vi "myRIO_BRig_RT_v0,75__PortC.vi"() -> ()   [LabVIEW 2014]
uses:
  <vilib>/Platform/TimedLoop/XDataNode/XDataNode.xnode
  <vilib>/Platform/TimedLoop/XDataNode/nitl_modes.ctl
  <vilib>/Platform/TimedLoop/XDataNode/XDNodeRunTimeDep.lvlib
  <vilib>/Platform/TimedLoop/XDataNode/wakeup.ctl
  <vilib>/Platform/TimedLoop/XDataNode/timing_clust.ctl
  <vilib>/rvi/interface/nirviReadWriteControl/nirviReadWriteControl.xnode
  <vilib>/rvi/interface/Simulation/niFpgaSimulationCallBeginRW.vi
  <vilib>/rvi/errors/niLvFpgaAdjustHostInterfaceError.vi
  <vilib>/rvi/interface/nirviCloseFPGA/nirviCloseFPGA.xnode
  <vilib>/myRIO/Instrument Drivers/Utilities/Utilities.lvlib
  <vilib>/rvi/interface/nirviOpenFPGA/nirviOpenFPGA.xnode
  myRIO_BRig_RT__Case_Exp_stateList.ctl
  <vilib>/WebDAVClient/Advanced/SessionHandle.ctl
  <vilib>/WebDAVClient/NI_WebDAV.lvlib
  myRIO_BRig_RT__Case_NonExp_stateList.ctl
  NiFpgaLv.dll
  <vilib>/Utility/error.llb/Error Cluster From Error Code.vi
  myRIO_BRig_FPGA_v3,60__PortC__build.lvbitx
  myRIO_BRig_FPGA_v3,60__PortC.vi
  <vilib>/FPGAPlugInAG/myRIO-1900/niLvFpga_Open_myRIO-1900.vi
  <vilib>/rvi/interface/common/dynamic/niFpgaDynamicAddResources.vi
  <vilib>/FPGAPlugInAG/Dynamic/niLvFpga_Close_Dynamic.vi
panel:
  in  "LC_Sel_All_Count":u16
  in  "LC_Sel_First_Count":u16
  in  "LC_Sel_All_Probability":u16
  in  "LC_Sel_All_Block":u16(slide) max=2 step=1 scale=0.0..2.0
  in  "LC_Sel_All_OnOff":bool
  in  "LC_Sel_First_Probability":u16
  in  "LC_Sel_First_Block":u16(slide) max=2 step=1 scale=0.0..2.0
  in  "LC_Sel_First_OnOff":bool
  in  "LC_Sel_All_Tdelay":u16
  in  "LC_Sel_First_Tdelay":u16
  out "I_connect_TCP":bool
  out "error out 5":errorcluster
  in  "get_countPerMS":bool
  in  "count_warmup_R_reset":bool
  in  "count_warmup_L_reset":bool
  out "count_warmup_R":u16
  out "count_warmup_L":u16
  out "SolenoidReward":bool
  in  "SolenoidProbability_L":u16=50 caption="Reward Time [ms]" min=1 max=1000 step=1
  in  "SolenoidProbability_R":u16=50 caption="Reward Time [ms]" min=1 max=1000 step=1
  out "output_PortA":dbl caption="LaserPower"
  out "error out 4":errorcluster
  in  "laser_power_step":dbl
  in  "laser_power_max":dbl
  in  "Recording":bool
  out "error out 3":errorcluster
  out "error out 2":errorcluster
  in  "laser_power_min":dbl
  in  "f_millisec2count":dbl=159.0
  in  "laser_Tshutter":dbl=2.0
  in  "laser_Freq":dbl=10.0
  in  "laser_Tpeak":dbl=2.0
  in  "laser_duration":u16
  out "error out":errorcluster
  in  "LC_Cue1_All_Count":u16
  in  "LC_Cue1_First_Count":u16
  in  "LC_Cue1_All_delayOpt":bool
  in  "LC_ENL1_All_delayOpt":bool
  in  "LC_ENL1_All_Count":u16
  in  "LC_ENL1_First_Count":u16
  in  "LC_Cue1_First_delayOpt":bool
  in  "LC_ENL1_First_delayOpt":bool
  in  "Tcycle_Cue_max":u16=1000 caption="Max" min=5 max=5000 step=5
  in  "Tcycle_Cue_min":u16=1000 caption="Min" min=5 max=5000 step=5
  in  "SendData":bool
  out "cSpout":enum16{"Left", "Right"}(ring) caption="Left or Right Spout"
  out "A4":u32 caption="LickCounter_Right"
  out "A2":u32 caption="LickCounter_Left"
  in  "laserResponse_wrong_LED":bool
  out "error_initTrial":errorcluster
  out "error_Selection_pre":errorcluster
  out "error_Selection":errorcluster
  out "SelectWrong":bool
  out "SelectReward":bool
  in  "Left(F)_or_Right(T)":bool
  in  "ignoreWrong":bool
  in  "SelectionState":bool
  in  "laserResponse_wrong":bool
  in  "laserResponse_reward":bool
  in  "laserResponse_reward_LED":bool
  out "nRewards_Right":u16 caption="# Rewards Total (Right)"
  out "nRewards_Left":u16 caption="# Rewards Total (Left)"
  out "nRewards_cur":u16 caption="# Rewards in Current Block"
  out "TpB_target":u16 caption="Target Trials Per Block"
  out "cState_NonExp":T1 caption="WarmUp State"
  out "iBlock":u16 caption="Current Block"
  out "cState":T2 caption="Experimental State"
  out "iTrial":u16 caption="Current Trial"
  in  "warmupType":u8(slide) max=2 step=1 scale=0.0..2.0
  in  "TestConnection":bool
  in  "warmup":bool caption="WarmUp"
  in  "Data Set Prefix":string="Exp1_TM2"
  out "Connected To Host?":bool
  in  "Host Password":string="sabalab"
  in  "Host UserName":string="Test2"
  in  "sp_RightSpout":u16(slide)=2 max=2 step=1 scale=0.0..2.0
  in  "sp_LeftSpout":u16(slide)=2 max=2 step=1 scale=0.0..2.0
  in  "BUR_max":u16 caption="Count Reward Structure  (0 = off)"
  in  "LC_Wrong_Probability":u16
  in  "LC_Wrong_Trial":u16(slide) max=2 step=1 scale=0.0..2.0
  in  "LC_Wrong_Block":u16(slide) max=2 step=1 scale=0.0..2.0
  in  "LC_Wrong_OnOff":bool
  in  "LC_Reward_Probability":u16
  in  "LC_Reward_Trial":u16(slide) max=2 step=1 scale=0.0..2.0
  in  "LC_Reward_Block":u16(slide) max=2 step=1 scale=0.0..2.0
  in  "LC_Reward_OnOff":bool
  in  "LC_Cue1_All_Probability":u16
  in  "LC_Cue1_All_Block":u16(slide) max=2 step=1 scale=0.0..2.0
  in  "LC_Cue1_All_OnOff":bool
  in  "LC_Cue1_First_Probability":u16
  in  "LC_Cue1_First_Block":u16(slide) max=2 step=1 scale=0.0..2.0
  in  "LC_Cue1_First_OnOff":bool
  in  "LC_ENL1_All_Probability":u16 max=100 step=1
  in  "LC_ENL1_All_Block":u16(slide) max=2 step=1 scale=0.0..2.0
  in  "LC_ENL1_All_OnOff":bool
  in  "LC_ENL1_First_Probability":u16 max=100 step=1
  in  "LC_ENL1_First_Block":u16(slide) max=2 step=1 scale=0.0..2.0
  in  "Tcycle_Timeout":u16=1000 caption="Timeout Time [ms]" min=10 max=10000 step=1
  in  "Tcycle_Wrong":u16=1000 caption="Wrong Time [ms]" min=10 max=10000 step=1
  in  "Tcycle_Selection":u16=1000 caption="Answer Time [ms]" min=1 max=10000 step=1
  in  "Tcycle_RewardPost":u16=1000 caption="Consumption Time [ms]" min=250 max=10000 step=250
  in  "Tcycle_Reward_L":u16=500 caption="Reward Time [ms]" min=1 max=1000 step=1
  in  "Tcycle_Reward_R":u16=500 caption="Reward Time [ms]" min=1 max=1000 step=1
  in  "TpB_Max_R":u16=4 caption="Max TrialsPerBlock" min=1 max=12 step=1
  in  "TpB_Min_R":u16=4 caption="Min TrialsPerBlock" min=1 max=12 step=1
  in  "TpB_Max_L":u16=4 caption="Max TrialsPerBlock" min=1 max=12 step=1
  in  "TpB_Min_L":u16=4 caption="Min TrialsPerBlock" min=1 max=12 step=1
  in  "BUR_min":u16 caption="Count Reward Structure\n(0 = off)"
  in  "TrialUntilReward":bool caption="Ignore Wrong Selection"
  in  "CueCycles":u16=1 caption="Cue Structure" min=1 max=1 step=1
  in  "MTrig_Laser_Tcycle":u16=10 caption="Time [ms]"
  in  "MTrig_Laser_trig":bool
  in  "MTrig_Audio_trig__R":bool caption="Trigger Audio"
  in  "MTrig_Audio_trig__L":bool caption="Trigger Audio"
  in  "RewCalib_Trig_R":bool caption="Calibrate_R"
  in  "RewCalib_Trig_L":bool caption="Calibrate_L"
  in  "MTrig_Solenoid_Tcycle__R":u16=300 caption="Time [ms]"
  in  "MTrig_Solenoid_Tcycle__L":u16=300 caption="Time [ms]"
  in  "MTrig_Solenoid_trig__R":bool caption="Solenoid"
  in  "MTrig_Solenoid_trig__L":bool caption="Solenoid"
  in  "STOP_abort":bool caption="Stop LabView\n(Stops myRio and FPGA)"
  in  "STOP_endBlock":bool caption="Stop Experiment\n@ End of Block"
  in  "STOP_endTrial":bool caption="Stop Experiment\n@ End of Trial"
  in  "START":bool caption="Start Experiment"
  in  "Tcycle_CuePenalty":u16=1000 caption="Penalty" min=1 max=10000 step=1
  in  "Audio_Amp__R":u16=100 caption="Amp"
  in  "Audio_Freq__R":u8=5 caption="Freq [kHz]" max=14 step=1
  in  "Audio_Amp__L":u16=100 caption="Amp"
  in  "Audio_Freq__L":u8=5 caption="Freq [kHz]" max=14 step=1
  in  "LC_Wrong_Tdelay":u16
  in  "LC_Cue1_All_Tdelay":u16
  in  "LC_ENL1_All_Tdelay":u16
  in  "LC_Reward_Tdelay":u16
  in  "LC_Cue1_First_Tdelay":u16
  in  "LC_ENL1_First_Tdelay":u16
  in  "LC_ENL1_First_OnOff":bool
  in  "Tcycle_ENLPenalty":u16=100 caption="Penalty" min=10 max=10000 step=10
  in  "Tcycle_ENL_max":u16=1000 caption="Max" min=250 max=10000 step=250
  in  "Tcycle_ENL_min":u16=1000 caption="Min" min=250 max=10000 step=250
  # "Communication (Host PC)"
  # "Recording Rig"
  # "Experimental Run"
  # "Current State"
  # "STOP experiment at"
  # "Global Parameters                                                         Trial Parameters"
  # "Left/Right        Give Reward?        Laser Power [V]"
  # "FPGA Count per [ms]"
  # "Experiment Task Structure"
  # "Timing [ms]"
  # "Block                   Trial            Target Trials       # Rewards \n                                                            Per Block             Current"
  # "Min            Max            Penalty"
  # "(1) = Switching\n(2) = Two Choice"
  # "WarmUp State"
  # "Lick Counter"
  # "Enforced\nNonLick"
  # "WarmUp"
  # "Left           Right"
  # "Cue then reward (no lick)\n \nLeft                    Right"
  # "# Rewards Total\n                                                                  Left                    Right"
  # "Cue"
  # "Experimental State"
  # "Selection\n \n\n \nReward\n    Dispense\n    Time\n \n    Dispense\n    Probability\n \n\n    Consumption\n    Time\n\nWrong Choice\n \n \nTimeout Penalty"
  # "Laser Control\n                               On/Off      Block        Probability [%]   Delay [ms]                              Count"
  # "Left                  Right"
  # "Manual Control"
  # "Enforced\nNonLick\n      1"
  # "Min"
  # "Max"
  # "from end"
  # "Solenoid\n \nLeft              Right"
  # "Switch\nTrial"
  # "Speaker\n \nLeft                    Right"
  # "Laser"
  # "from start"
  # "Trial Per Block Structure \n               Left                        Right"
  # "from end"
  # "NonSwitch\nTrials"
  # "from start"
  # "Time\n[ms]"
  # "Time\n[ms]"
  # "Time = Cue Min"
  # "Min"
  # "Cue 1"
  # "Power = Min"
  # "from end"
  # "Switch\nTrial"
  # "Max"
  # "from start"
  # "Speaker Parameters"
  # "Laser Parameters"
  # "Left                  Right"
  # "from end"
  # "Laser Response\n                               On/Off      Block       Trial       Probability [%]   Delay [ms]"
  # "Frequency\n[Hz]"
  # "NonSwitch\nTrials"
  # "Frequency\n[kHz]"
  # "from start"
  # "Timing [ms]\n Duration     Peak Width   Shutter"
  # "Selection Reward"
  # "Selection"
  # "Amp\n(0 - 32,000)"
  # "from start"
  # "Switch\nTrial"
  # "Laser Power [V]\nMin          Max              Step"
  # "Speaker\nPattern\nDuring Cue"
  # "Selection Wrong"
  # "from start"
  # "NonSwitch\nTrials"
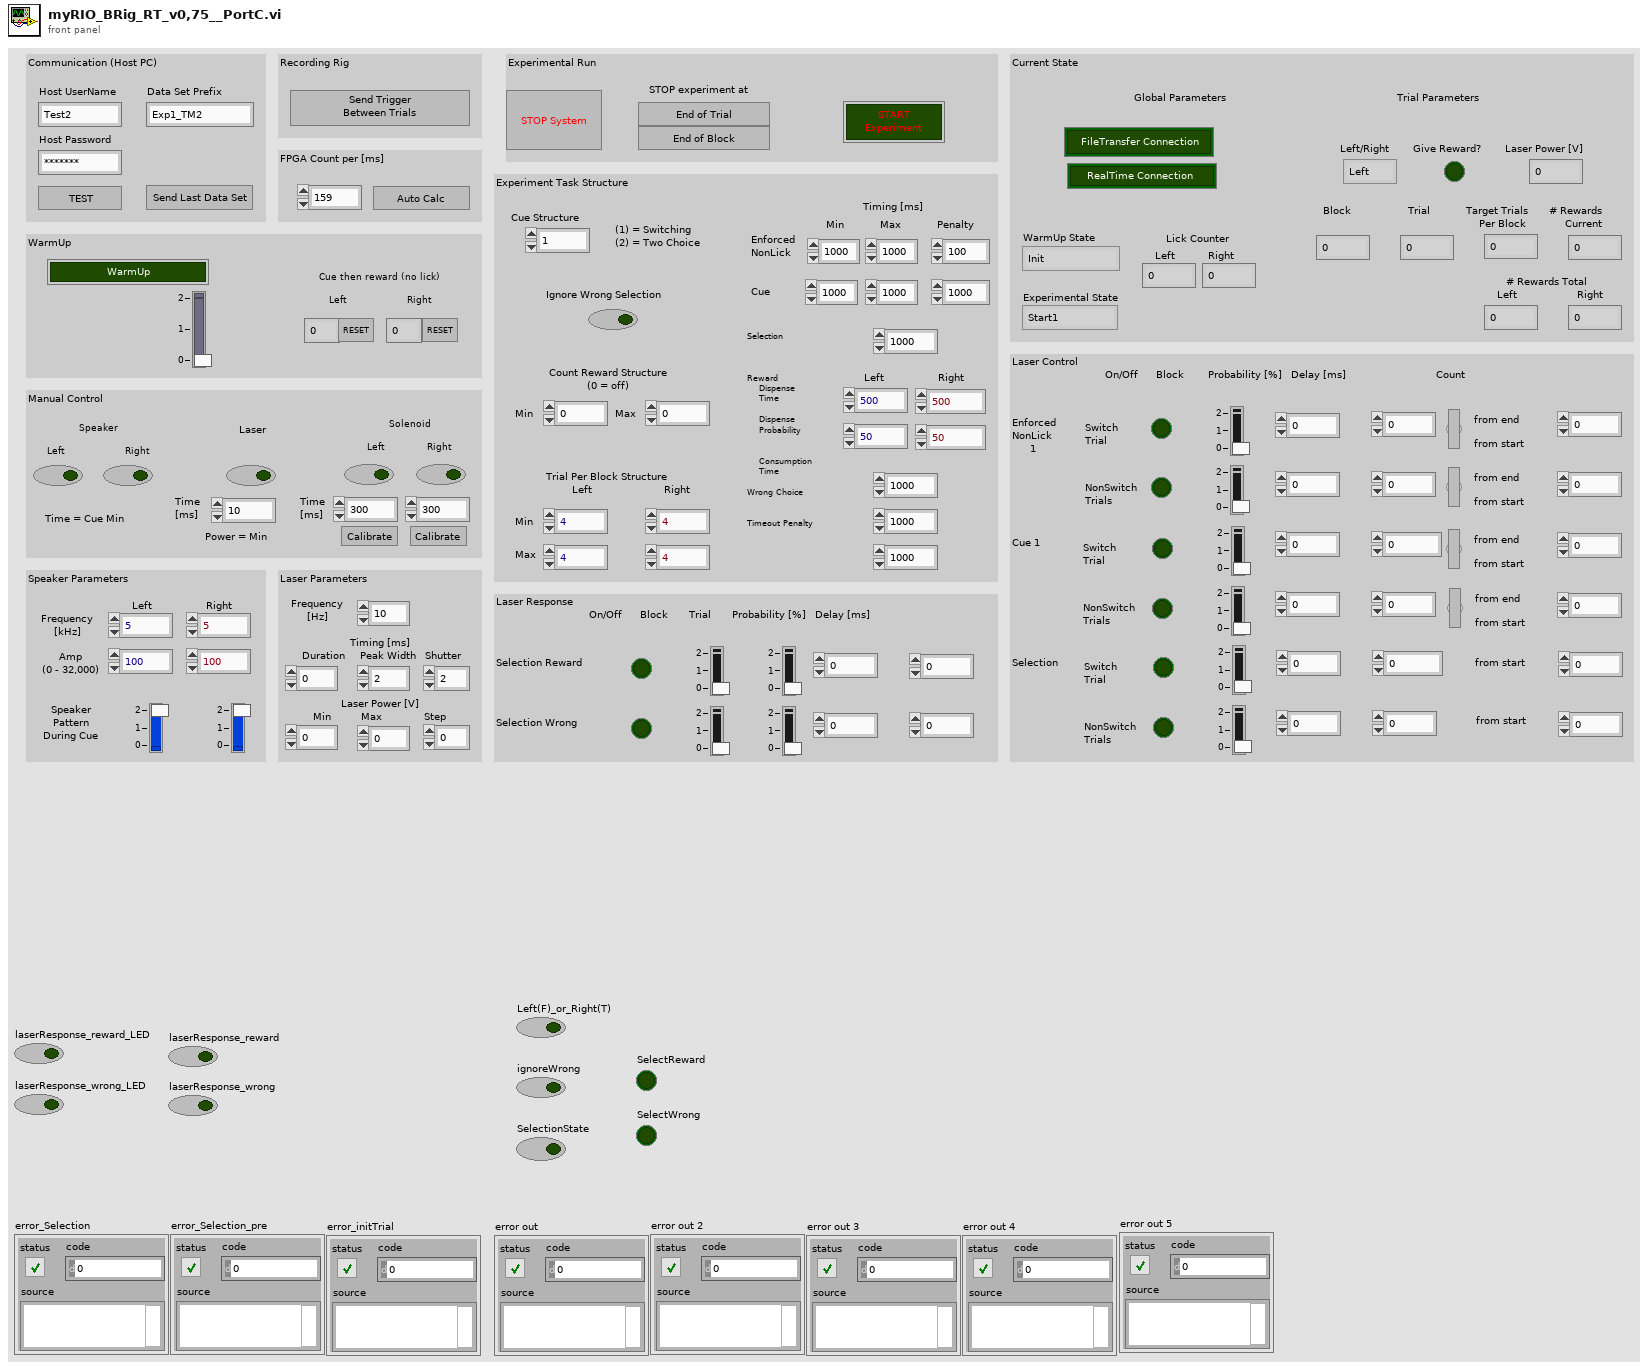
[diagram p1: front panel]
types:
  T1 = typedef "myRIO_BRig_RT__Case_NonExp_stateList.ctl" = enum16{"Init", "UploadSettings_pre", "UploadSettings_Read_dataExp", "UploadSettings_dataExp_1", "UploadSettings_Read_dataLC", "UploadSettings_dataLC_1", "UploadSettings_dataLC_2", "UploadSettings_Read_dataMTrig", "UploadSettings_dataMTrig_1", "UploadSettings_post", "Idle_pre", "IdleEmpty", "IdleEmpty2", "IdleEmpty3", "IdleEmpty4", "Idle", "Idle_2", "Idle_3", "Idle_4", "Idle_post", "Cue_pre__pre", "Cue_pre", "Cue", "Cue_post", "RewardCalibration_pre", "DispenseWater_pre__pre", "DispenseWater_pre", "DispenseWater", "DispenseWater_post", "TestConnection", "SendData", "Get_FPGA_count_per_ms", "End"}
  T2 = typedef "myRIO_BRig_RT__Case_Exp_stateList.ctl" = enum16{"Start1", "Start2", "Start3", "saveSettings1", "saveSettings2", "saveSettings3", "saveSettings4_LC_l1_ENL", "saveSettings4_LC_l2_ENL", "saveSettings5_LC_l1_Cue", "saveSettings5_LC_l2_Cue", "saveSettings6_LC_l1_Other", "SaveSettings6_LC_l2_Other", "setSettings_Audio", "setSettings_Laser", "initBlock_pre", "initBlock", "initBlock2", "initBlock_post", "initTrial_pre", "initTrial", "initTrial2", "initTrial3", "initTrial4", "initTrial_LC_ENL1", "initTrial_LC_Cue1", "initTrial_LC_Sel", "initTrial_post", "ENL1_pre", "ENL1", "ENL1_post", "ENL1Penalty_pre", "ENL1Penalty", "ENL2_pre", "ENL2", "ENL2Penalty_pre", "ENL2Penalty", "Cue1_pre", "Cue1", "Cue1_post", "Cue1Penalty_pre", "Cue1Penalty", "Cue2_pre", "Cue2", "Cue2Penalty_pre", "Cue2Penalty", "Selection_pre", "Selection", "Select_post", "SelectReward_pre", "SelectReward", "SelectRewardPost_pre", "SelectRewardPost", "SelectWrong_pre", "SelectWrong", "SelectWrong_post", "SelectTimeout_pre", "SelectTimeout", "SelectTimeout_post", "endTrial_pre", "endTrial1", "endTrial2", "endTrial3", "endTrial_post", "endBlock_pre", "endBlock", "endBlock_post", "endExp", "commConnect", "commUpload_pre", "commUpload_dataBlock", "commUpload_dataCurrent", "commUpload_dataExp", "commUpload_dataLC", "commUpload_dataTrial", "commUpload_post", "saveData_pre", "saveData_dataBlock", "saveData_dataCurrent", "saveData_dataExp", "saveData_dataLC", "saveData_dataTrial", "saveData_post", "empty_endBlock1", "empty_endBlock2", "empty_endTrial1", "empty_endTrial2", "empty_endTrial3", "empty_endTrial4", "empty_endTrial5", "dummyState", "dummyState_endBlock"}
  T3 = typedef "XDNodeRunTimeDep.lvlib/timing_clust.ctl" = cluster{"Expected End [f-1]":u64, "Actual End [f-1]":u64, "Finished Late? [f-1]":bool, "Expected End [i-1]":u64, "Actual End [i-1]":u64, "Finished Late? [i-1]":bool, "Expected Start [i]":u64, "Actual Start [i]":u64, "Expected Start [f]":u64, "Actual Start [f]":u64, "Source Name":string, "Structure Name":string, "Period":i64, "Deadline":i64, "Offset":i64, "Start":i64, "Priority":i32, "Timeout":i32, "Mode":T4, "Wakeup Reason":T5, "Error":errorcluster, "Source Type":string, "Secondary Source Type":string, "Global End Time":u64, "Global Start Time":u64, "Frame Duration":u64, "Iteration Duration":u64, "Assigned CPU":i32, "I/O Scan Engine Mode":u32}
  T4 = typedef "XDNodeRunTimeDep.lvlib/nitl_modes.ctl" = enum32{"No Change", "Process missed periods, maintain original phase", "Discard missed periods, maintain original phase", "Process missed periods, ignore original phase", "Discard missed periods, ignore original phase"}
  T5 = typedef "XDNodeRunTimeDep.lvlib/wakeup.ctl" = enum32{"Normal", "Aborted", "Asynchronous wakeup", "Timing source error", "Timed loop error", "Timeout"}
  T6 = typedef "myRIO_BRig_RT__Case_Exp_stateList.ctl" = enum16{"Start1", "Start2", "Start3", "saveSettings1", "saveSettings2", "saveSettings3", "saveSettings4_LC_ENL", "saveSettings5_LC_Cue", "saveSettings6_LC_Other", "setSettings_Audio", "setSettings_Laser", "initBlock_pre", "initBlock", "initBlock2", "initBlock_post", "initTrial_pre", "initTrial", "initTrial2", "initTrial3", "initTrial4", "initTrial_LC_ENL1", "initTrial_LC_Cue1", "initTrial_LC_Sel", "initTrial_post", "ENL1_pre", "ENL1", "ENL1_post", "ENL1Penalty_pre", "ENL1Penalty", "ENL2_pre", "ENL2", "ENL2Penalty_pre", "ENL2Penalty", "Cue1_pre", "Cue1", "Cue1_post", "Cue1Penalty_pre", "Cue1Penalty", "Cue2_pre", "Cue2", "Cue2Penalty_pre", "Cue2Penalty", "Selection_pre", "Selection", "Select_post", "SelectReward_pre", "SelectReward", "SelectRewardPost_pre", "SelectRewardPost", "SelectWrong_pre", "SelectWrong", "SelectWrong_post", "SelectTimeout_pre", "SelectTimeout", "SelectTimeout_post", "endTrial_pre", "endTrial1", "endTrial2", "endTrial3", "endTrial_post", "endBlock_pre", "endBlock", "endBlock_post", "endExp", "commConnect", "commUpload_pre", "commUpload_dataBlock", "commUpload_dataCurrent", "commUpload_dataExp", "commUpload_dataLC", "commUpload_dataTrial", "commUpload_post", "saveData_pre", "saveData_dataBlock", "saveData_dataCurrent", "saveData_dataExp", "saveData_dataLC", "saveData_dataTrial", "saveData_post", "empty_endBlock1", "empty_endBlock2", "empty_endTrial1", "empty_endTrial2", "empty_endTrial3", "empty_endTrial4", "empty_endTrial5", "dummyState", "dummyState_endBlock"}
  T7 = typedef "NI_WebDAV.lvlib/SessionHandle.ctl" = refnum<k1>
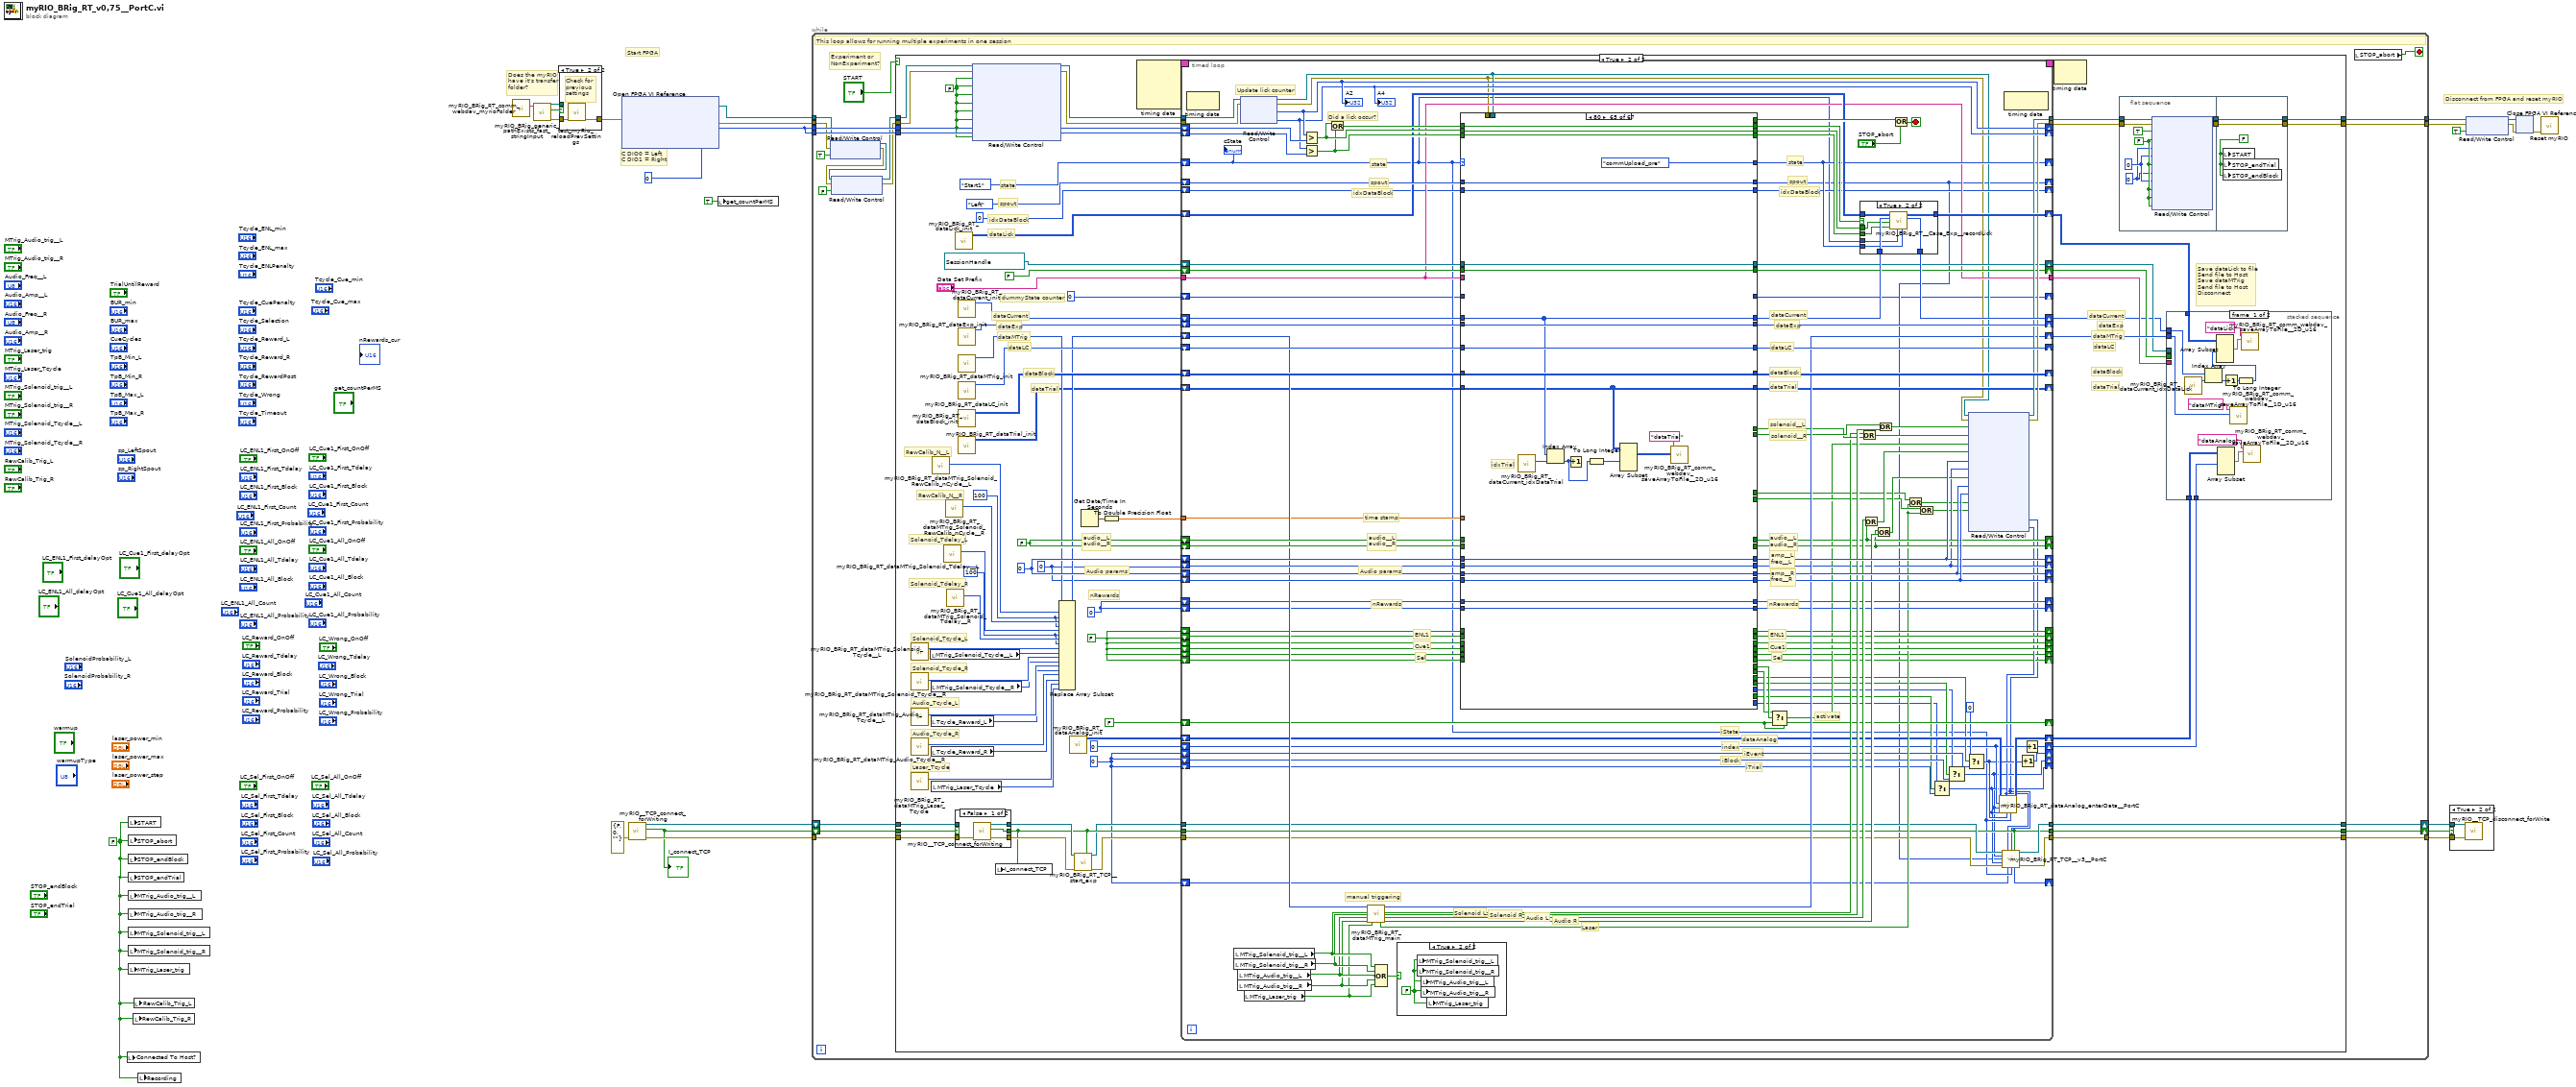
[diagram p0: block diagram]
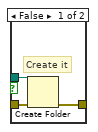
[diagram p3: hidden frame]
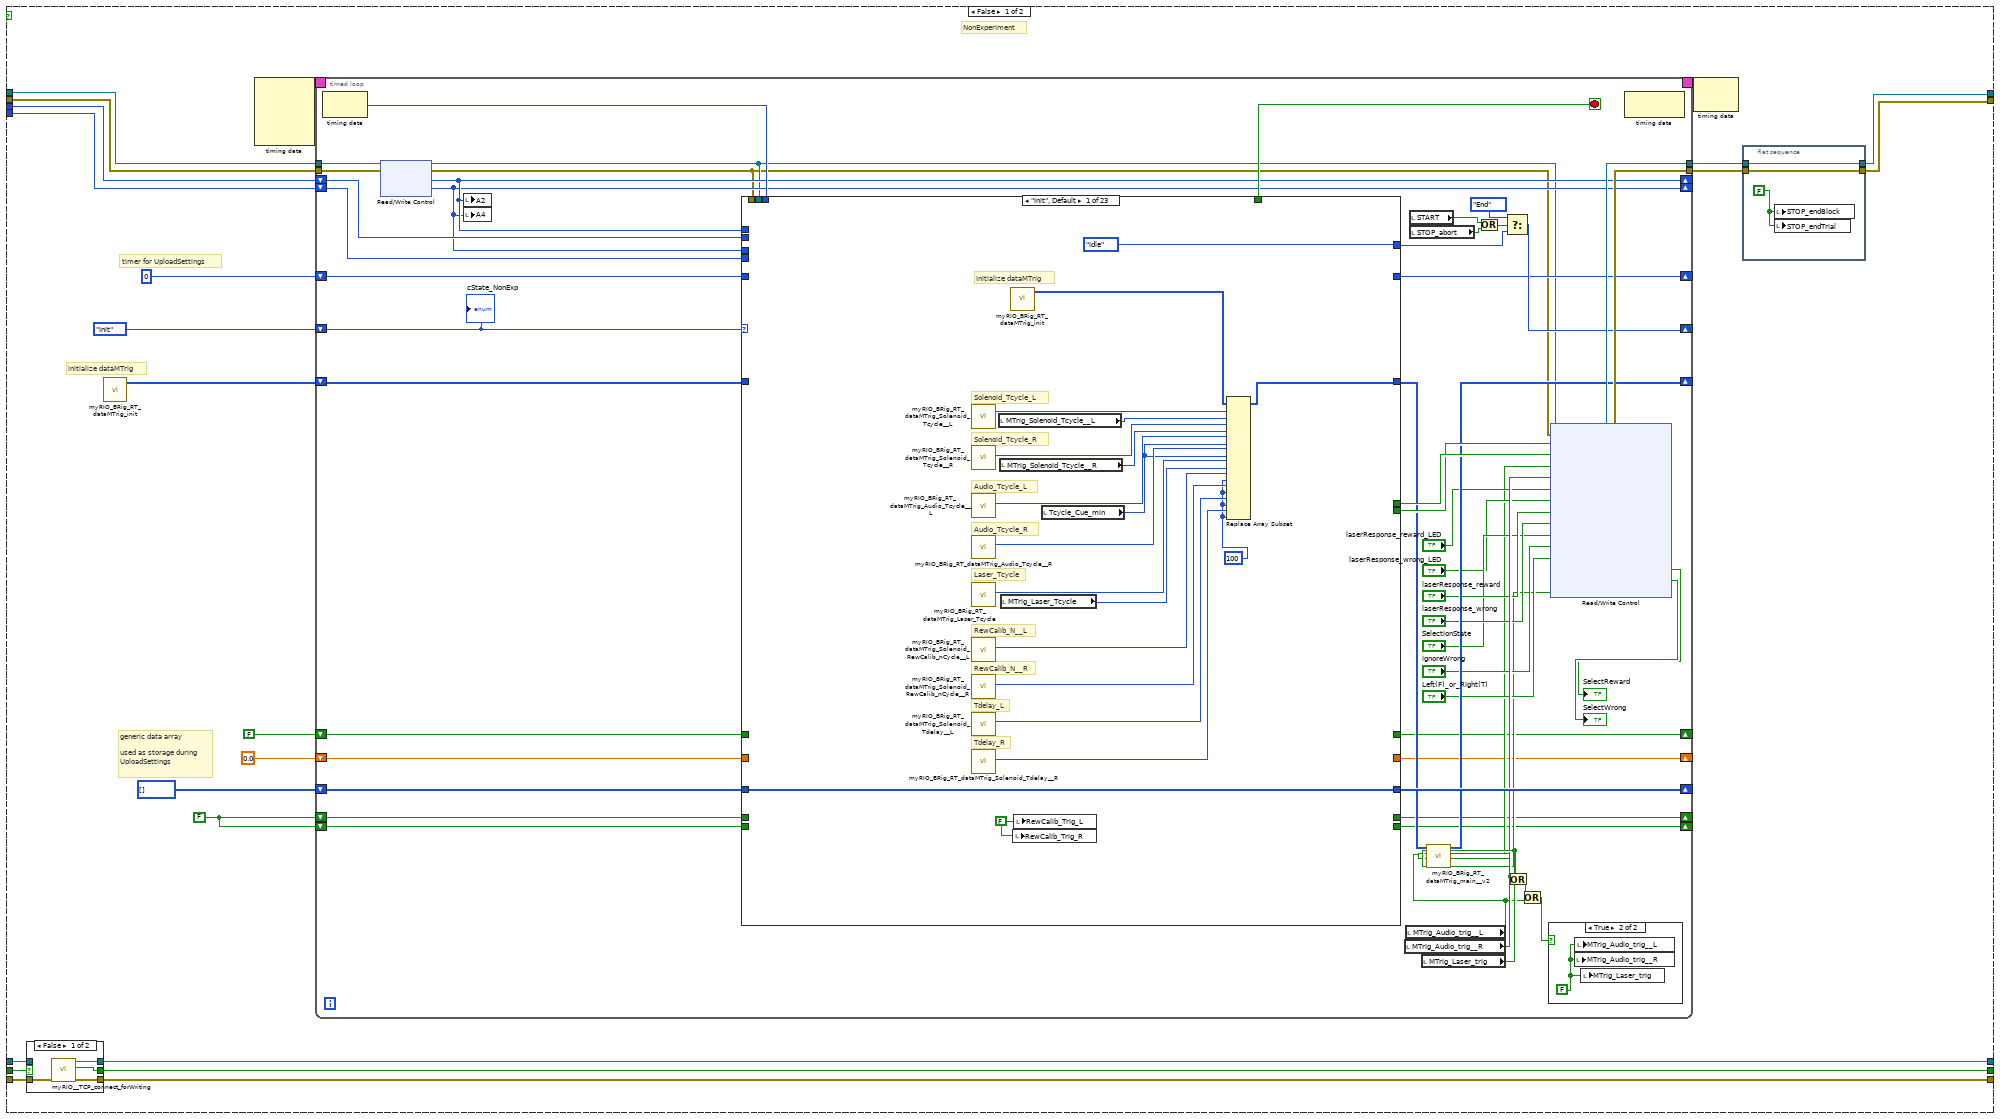
[diagram p4: hidden frame]
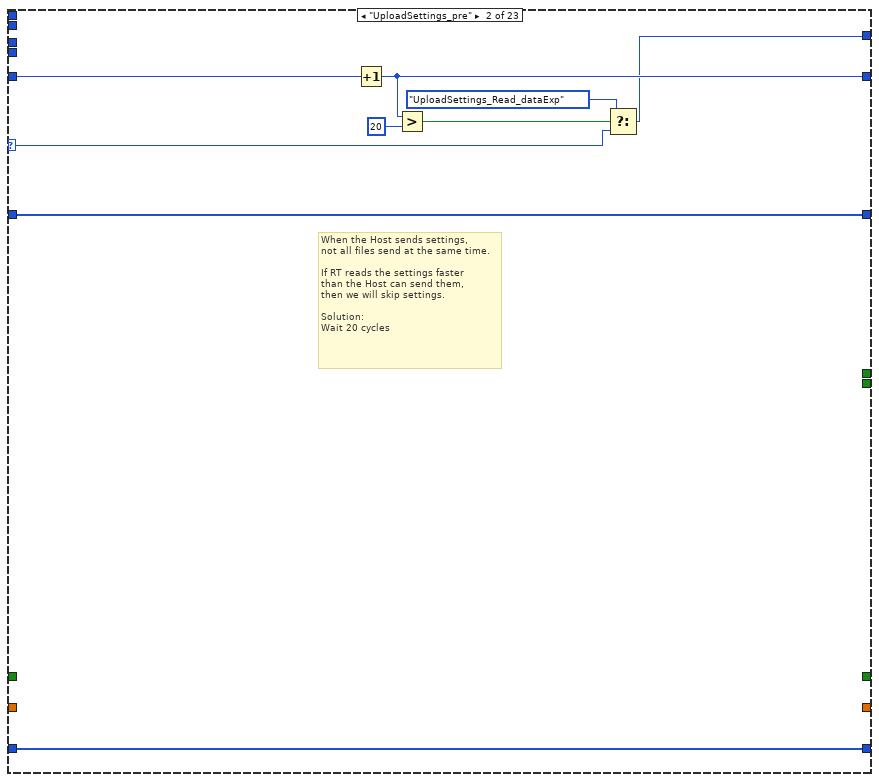
[diagram p7: hidden frame]
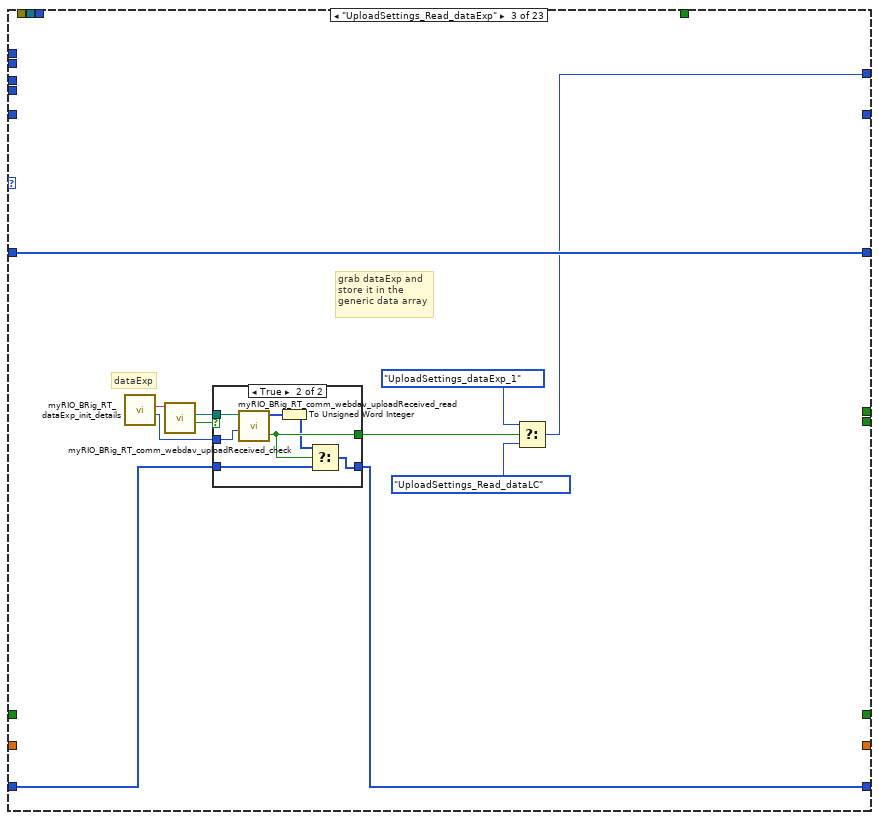
[diagram p8: hidden frame]
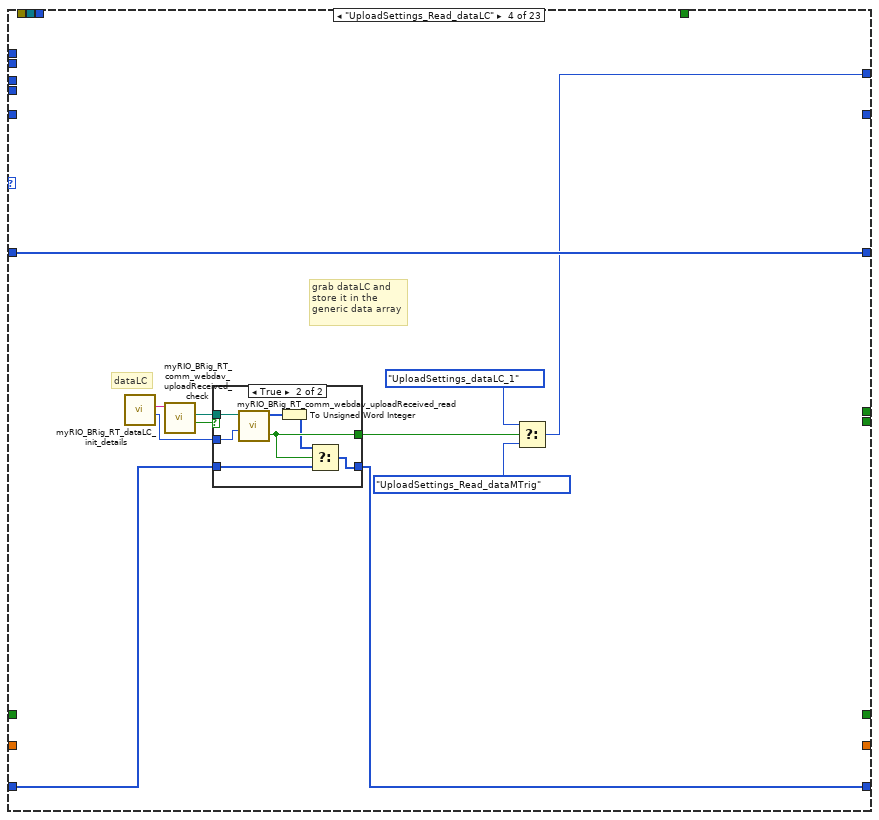
[diagram p10: hidden frame]
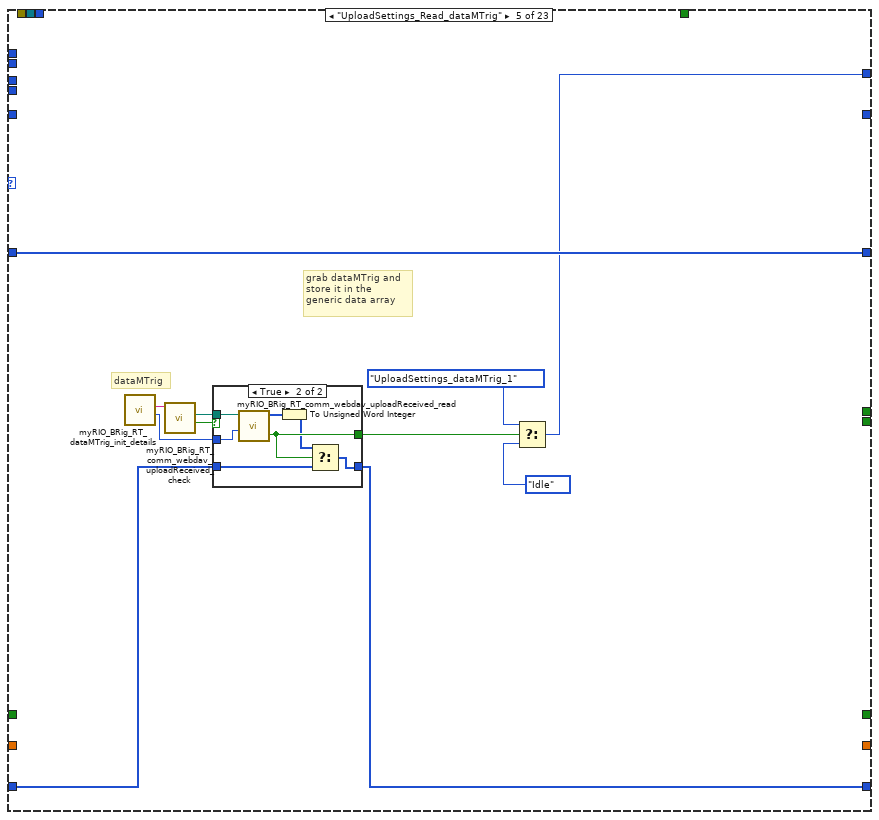
[diagram p12: hidden frame]
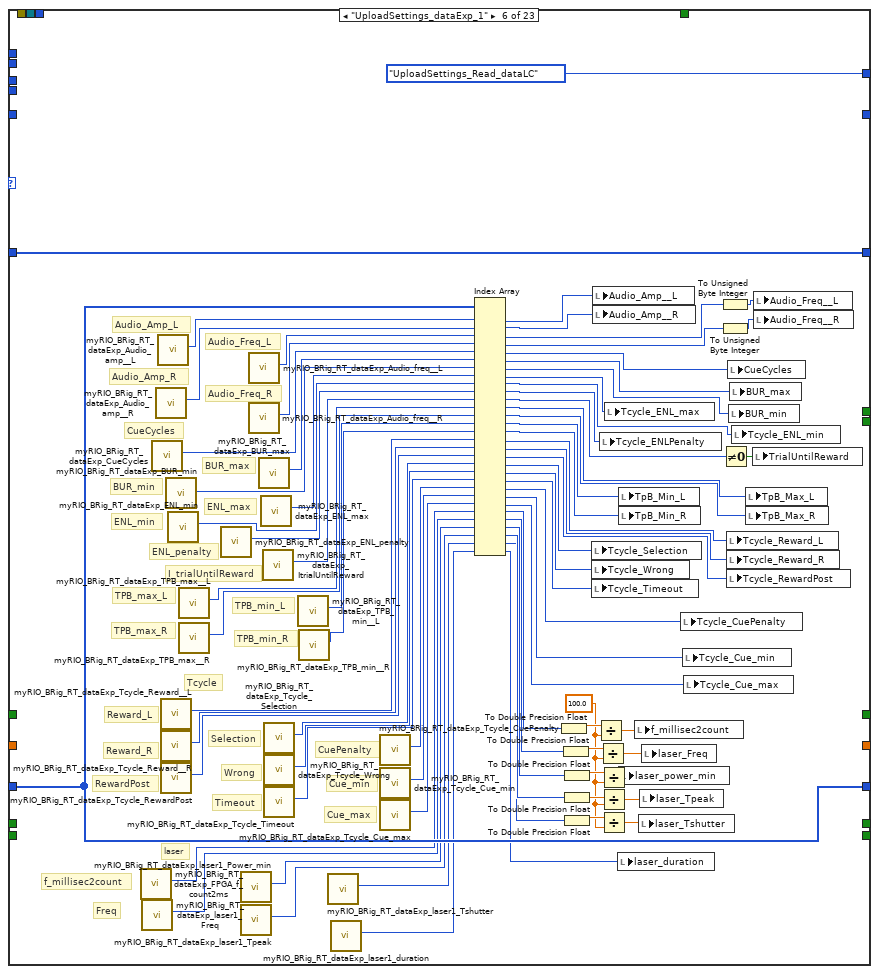
[diagram p14: hidden frame]
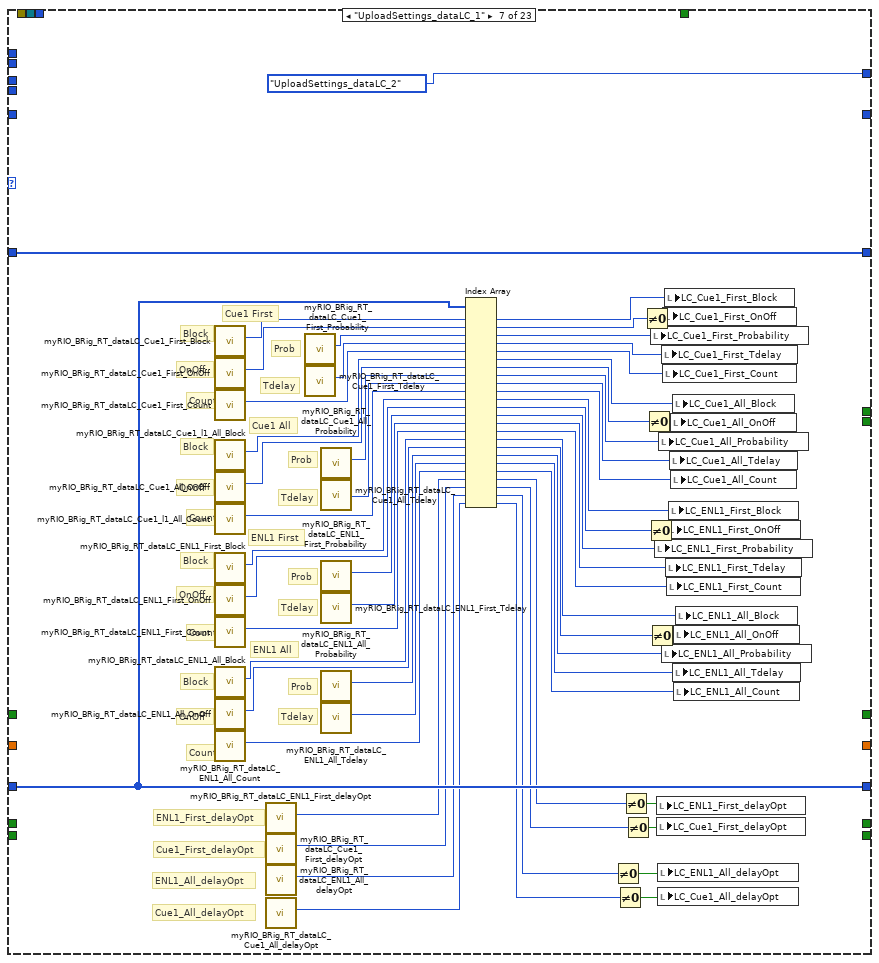
[diagram p15: hidden frame]
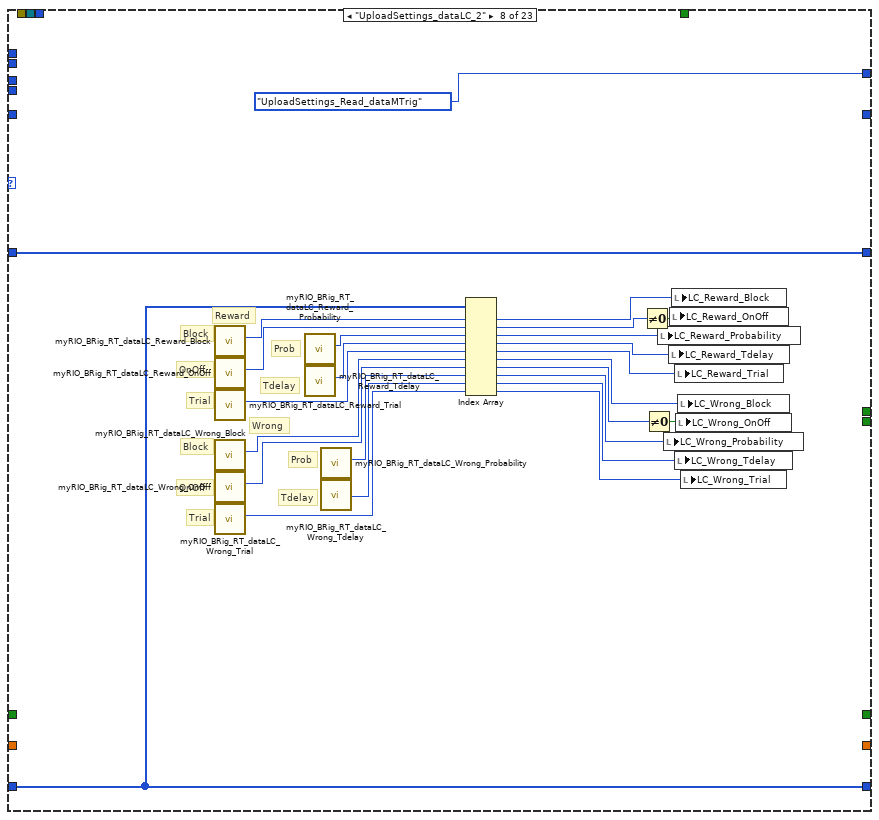
[diagram p16: hidden frame]
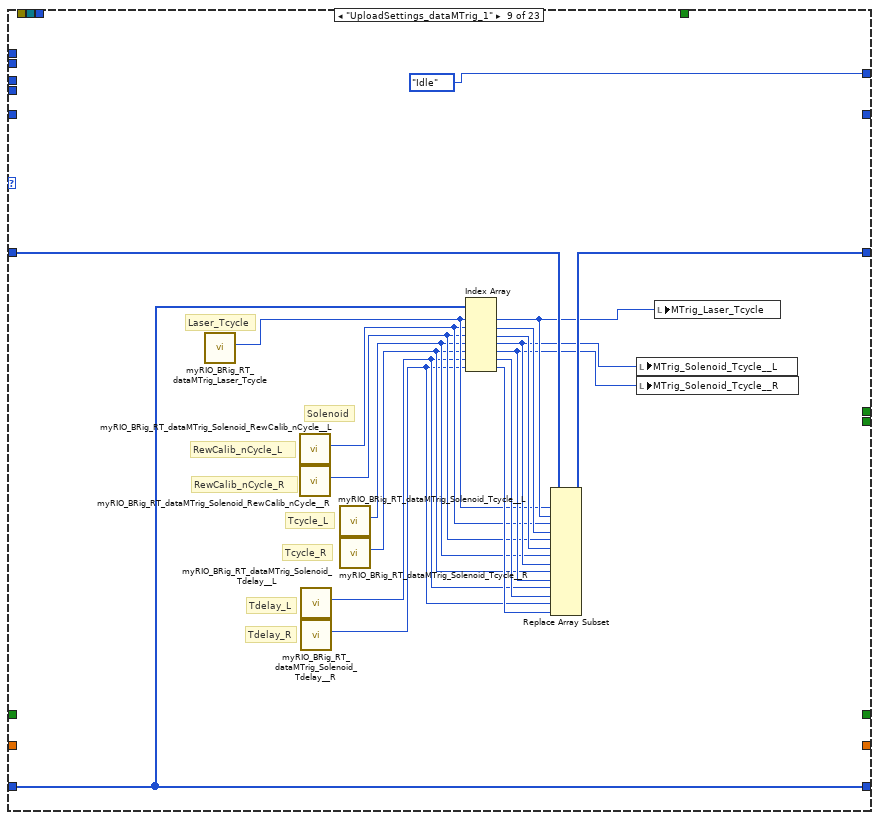
[diagram p17: hidden frame]
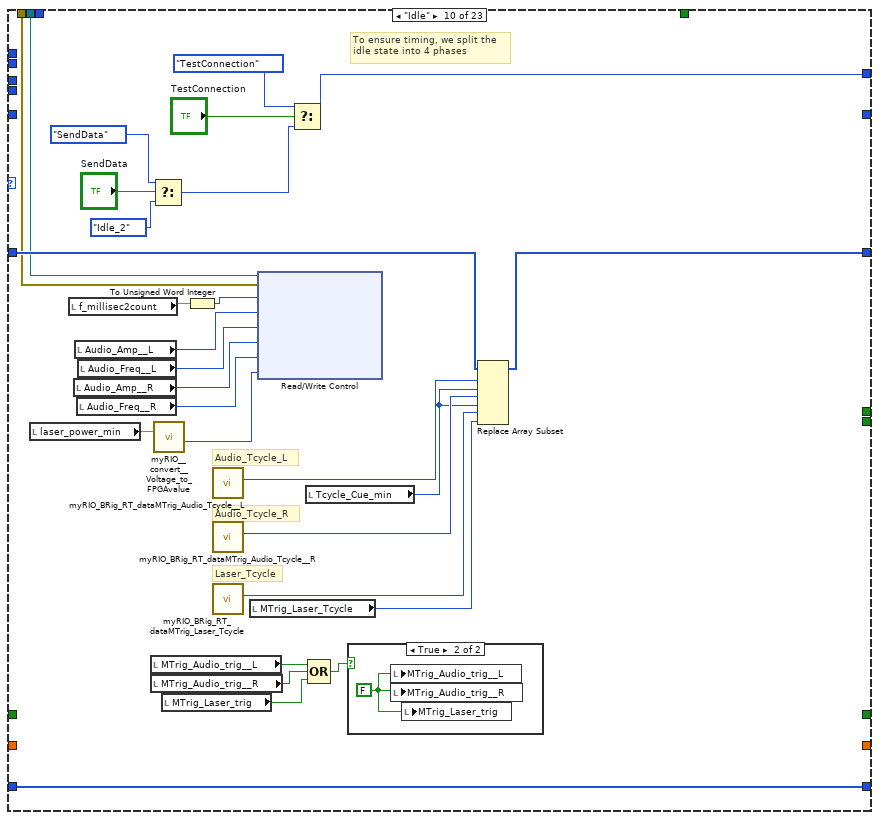
[diagram p18: hidden frame]
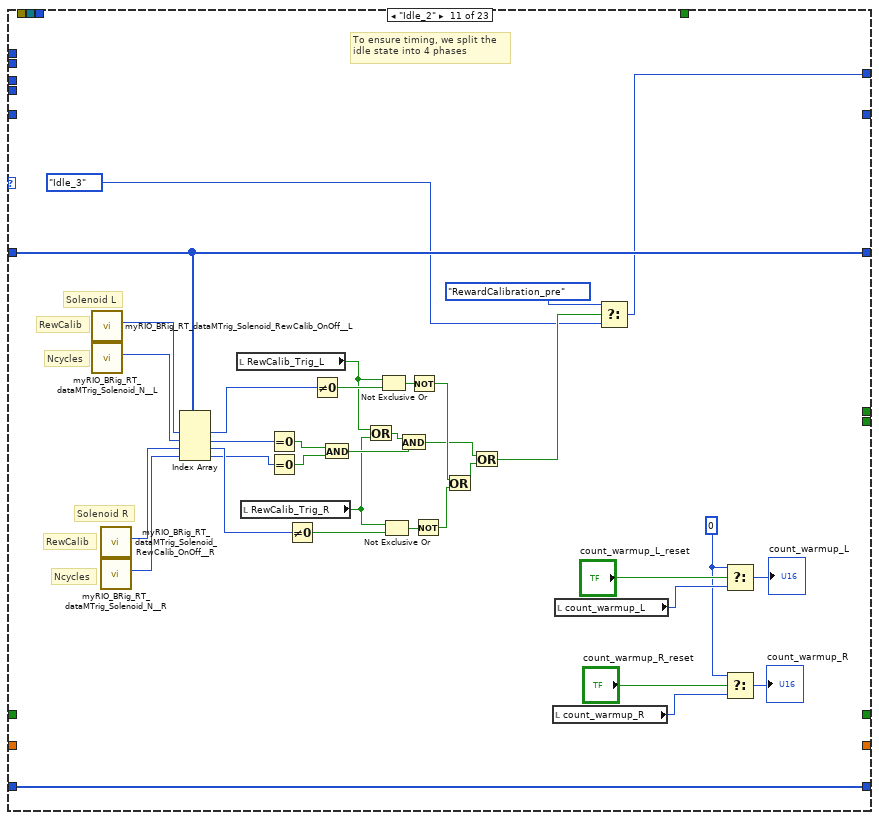
[diagram p20: hidden frame]
diagram:
  w17 = u32 0
  w1 = FALSE
  # "Does the myRIO\nhave it's transfer\nfolder?"
  # "C DIO0 = Left\nC DIO1 = Right"
  # "Start FPGA"
  # "Disconnect from FPGA and reset myRIO"
  n1 = local write "Connected To Host?"(w1) -> ()
  n2 = local write "START"(w1) -> ()
  n3 = local write "STOP_abort"(w1) -> ()
  n4 = local write "STOP_endBlock"(w1) -> ()
  n5 = local write "STOP_endTrial"(w1) -> ()
  n6 = local write "MTrig_Audio_trig__L"(w1) -> ()
  n7 = local write "MTrig_Audio_trig__R"(w1) -> ()
  n8 = local write "MTrig_Solenoid_trig__L"(w1) -> ()
  n9 = local write "MTrig_Solenoid_trig__R"(w1) -> ()
  n10 = local write "MTrig_Laser_trig"(w1) -> ()
  n11 = local write "RewCalib_Trig_R"(w1) -> ()
  n12 = local write "RewCalib_Trig_L"(w1) -> ()
  n13 = local write "Recording"(w1) -> ()
  n14 = call "myRIO_BRig_RT_comm_webdav_myrioFolder.vi"() -> ("output_myrioFolder"=w14:string)  [unwired: 11 in]
  n15 = call "myRIO_BRig_generic_pathExists_fast_stringInput.vi"("input_filePath"=w14) -> ("output_error"=w13:errorcluster, "output_Iexist"=w12:bool, "output_filePath"=w11:path)  [unwired: 8 in]
  n16 = case shown="True" w12 {
    tunnel: w11 -> [w26 _]
    tunnel: w13 -> [w25 w28]
    tunnel: [w24 w27] -> w9
    frame False {
      # "Create it"
      n17 = Create Folder(path (use dialog)=w26, error in=w25) -> (error out=w24:errorcluster)  [unwired: 1 in, 2 out]
    }
    frame True {
      # "Check for\nprevious\nsettings"
      n18 = call "test_myRio_reloadPrevSettings.vi"("input_error"=w28) -> ("output_error"=w27:errorcluster)  [unwired: 10 in]
    }
  }
  n19 = xnode "Open FPGA VI Reference"("error in"=w9) -> ("FPGA VI Reference Out"=w19:refnum<k20>, "error out"=w18:errorcluster)  [unwired: 1 in]
  n20 = call "myRIO__TCP_connect_forWriting.vi"("input_error"=errorcluster {"status"=FALSE, "code"=0, "source"=""}) -> ("output_error"=w7:errorcluster, "output_connected"=w6:bool, "output_hTCP"=w10:refnum<k5>)  [unwired: 8 in]
  "I_connect_TCP" <- w6
  n21 = local write "get_countPerMS"(TRUE ("get_countPerMS")) -> ()
  n22 = while {
    tunnel: w19 -> [w38]
    tunnel: w18 -> [w43]
    tunnel: w17 -> [w46]
    tunnel: w17 -> [w45]
    tunnel: [w36] -> w16
    tunnel: [w35] -> w15
    shift-right: [w32] -> w5
    shift-left: w6 -> [w33]
    tunnel: w7 -> [w31]
    shift-right: [w30] -> w4
    shift-left: w10 -> [w34]
    tunnel: [w29] -> w3
    stop <- w44 stop-if-true
    # "Experiment or\nNonExperiment?"
    # "This loop allows for running multiple experiments in one session"
    n23 = xnode "Read/Write Control"("FPGA VI Reference In"=w38, "error in"=w43, "Counts_Reset"=TRUE) -> ("FPGA VI Reference Out"=w40:refnum<k20>, "error out"=w41:errorcluster)
    n24 = xnode "Read/Write Control"("FPGA VI Reference In"=w40, "error in"=w41, "Counts_Reset"=FALSE) -> ("FPGA VI Reference Out"=w37:refnum<k20>, "error out"=w39:errorcluster)
    n25 = case shown="True" "START" {
      tunnel: w46 -> [w67 w995]
      tunnel: w45 -> [w66 w994]
      tunnel: w39 -> [w64 w945]
      tunnel: w37 -> [w65 w944]
      tunnel: [w62 w991] -> w36
      tunnel: [w60 w986] -> w35
      tunnel: w34 -> [w53 w932]
      tunnel: [w51 w936] -> w30
      tunnel: w33 -> [w52 w934]
      tunnel: [w50 w935] -> w32
      tunnel: w31 -> [w54 w933]
      tunnel: [w49 w931] -> w29
      frame False {
        w57 = FALSE
        # "generic data array\n\nused as storage during\nUploadSettings"
        # "timer for UploadSettings"
        # "initialize dataMTrig"
        # "NonExperiment"
        n26 = case shown="False" w52 {
          selector: w52 -> [_ w76]
          tunnel: w54 -> [w73 w78]
          tunnel: [w74 w78] -> w49
          tunnel: w53 -> [_ w77]
          tunnel: [w75 w77] -> w51
          tunnel: [w72 w76] -> w50
          frame False {
            n27 = call "myRIO__TCP_connect_forWriting.vi"("input_error"=w73) -> ("output_error"=w74:errorcluster, "output_connected"=w72:bool, "output_hTCP"=w75:refnum<k5>)  [unwired: 8 in]
          }
          frame True {
          }
        }
        n28 = call "myRIO_BRig_RT_dataMTrig_init.vi"() -> ("output_dataMTrig"=w68:u16[])  [unwired: 5 in]
        n29 = node-c288() -> (w71:T3)  [unwired: 4 in]
        n30 = timed-loop {
          timing: w71 -> [_]
          timing-out: [_] -> w70
          shift-right: [w121] -> _
          shift-left: w68 -> [w133]
          shift-right: [w110] -> _
          shift-left: myRIO_BRig_RT__Case_NonExp_stateList."Init" ("Enum") -> [w127]
          shift-right: [w94] -> _
          shift-left: w67 -> [w95]
          shift-right: [w92] -> _
          shift-left: w66 -> [w93]
          tunnel: [w129] -> w63
          tunnel: [w128] -> w61
          tunnel: w64 -> [w131]
          tunnel: w65 -> [w130]
          shift-right: [w126] -> _
          shift-left: u16[] [] ("output_data") -> [w125]
          shift-right: [w96] -> _
          shift-left: u16 0 ("Audio_Amp__L") -> [w97]
          shift-right: [w89] -> _
          shift-left: w57 -> [w91]
          shift-right: [w88] -> _
          shift-left: w57 -> [w90]
          shift-right: [w84] -> _
          shift-left: FALSE -> [w85]
          shift-right: [w82] -> _
          shift-left: 0.0 -> [w83]
          stop <- w134 stop-if-true
          n31 = node-c288() -> (w132:i64)  [unwired: 1 in]
          n32 = xnode "Read/Write Control"("FPGA VI Reference In"=w130, "error in"=w131) -> ("FPGA VI Reference Out"=w87:refnum<k20>, "error out"=w86:errorcluster, "A2_LickL"=w94:u32, "A4_LickR"=w92:u32)
          n33 = local write "A2"(w94) -> ()
          n34 = local write "A4"(w92) -> ()
          n35 = case shown="\"Init\", Default" w127 {
            selector: w127 -> [_ w159 _ _ _ _ _ _ _ _ _ _ _ _ w590 _ _ w798 _ _ _ w873 w917]
            tunnel: [myRIO_BRig_RT__Case_NonExp_stateList."Idle" ("Enum") w157 w164 w183 w202 myRIO_BRig_RT__Case_NonExp_stateList."UploadSettings_Read_dataLC" ("Enum") myRIO_BRig_RT__Case_NonExp_stateList."UploadSettings_dataLC_2" ("Enum") myRIO_BRig_RT__Case_NonExp_stateList."UploadSettings_Read_dataMTrig" ("f") myRIO_BRig_RT__Case_NonExp_stateList."Idle" ("Enum") w421 w438 w477 w558 myRIO_BRig_RT__Case_NonExp_stateList."Cue" ("t") w585 myRIO_BRig_RT__Case_NonExp_stateList."DispenseWater_pre" ("Enum") w743 w796 w819 myRIO_BRig_RT__Case_NonExp_stateList."Idle" ("Enum") myRIO_BRig_RT__Case_NonExp_stateList."Idle" ("Enum") w872 w917] -> w111
            tunnel: [w146 w156 w174 w193 w212 w297 w356 w381 w397 w425 w453 w482 w556 w574 w591 w653 w780 w803 w830 w865 w871 w884 w915] -> w122
            tunnel: [_ _ _ _ _ _ _ _ _ _ _ _ _ _ _ _ _ _ _ _ _ _ TRUE] -> w134
            tunnel: w133 -> [_ w156 w174 w193 w212 w297 w356 w381 w398 w424 w453 w483 w556 w575 w592 w639 w776 w804 w831 w865 w871 w884 w915]
            tunnel: w132 -> [_ _ _ _ _ _ _ _ _ _ _ _ _ _ _ _ _ w808 _ _ _ _ _]
            tunnel: [w139 w155 w165 w184 w203 w246 w312 w357 w382 w416 w437 w471 w555 w564 w599 w634 w728 w781 w812 w857 w869 w883 w914] -> w126
            tunnel: w125 -> [w139 w155 w166 w185 w204 w246 w312 w357 w382 w416 w437 w471 w555 w564 w599 w634 w728 w781 w812 w857 w869 w883 w914]
            tunnel: [_ _ _ _ _ _ _ _ _ _ _ _ _ _ _ _ _ w805 _ _ _ _ _] -> w124
            tunnel: [_ _ _ _ _ _ _ _ _ _ _ _ _ _ _ _ _ w787 _ _ _ _ _] -> w123
            tunnel: w97 -> [_ w163 _ _ _ _ _ _ _ _ _ _ _ _ _ _ _ _ _ _ _ _ _]
            tunnel: [_ w162 _ _ _ _ _ _ _ _ _ _ _ _ _ _ _ _ _ _ _ _ _] -> w96
            tunnel: w95 -> [_ _ _ _ _ _ _ _ _ _ _ _ _ _ w596 _ _ _ _ _ _ _ _]
            tunnel: w94 -> [_ _ _ _ _ _ _ _ _ _ _ _ _ _ w597 _ _ _ _ _ _ _ _]
            tunnel: w93 -> [_ _ _ _ _ _ _ _ _ _ _ _ _ _ w594 _ _ _ _ _ _ _ _]
            tunnel: w92 -> [_ _ _ _ _ _ _ _ _ _ _ _ _ _ w595 _ _ _ _ _ _ _ _]
            tunnel: w91 -> [_ _ _ _ _ _ _ _ _ _ _ _ _ _ w582 _ _ _ _ _ _ _ _]
            tunnel: w90 -> [_ _ _ _ _ _ _ _ _ _ _ _ _ _ w581 _ _ _ _ _ _ _ _]
            tunnel: [_ _ _ _ _ _ _ _ _ _ _ _ _ w563 w582 _ _ _ _ _ _ _ _] -> w89
            tunnel: [_ _ _ _ _ _ _ _ _ _ _ _ _ w562 w581 _ _ _ _ _ _ _ _] -> w88
            tunnel: w87 -> [_ _ _ _ _ _ _ _ _ w407 _ _ _ _ _ _ _ _ _ _ _ w878 _]
            tunnel: w86 -> [_ _ _ _ _ _ _ _ _ w406 _ _ _ _ _ _ _ _ _ _ _ w877 _]
            tunnel: w85 -> [_ _ _ _ _ _ _ _ _ _ _ _ _ _ _ _ _ _ _ _ _ w882 _]
            tunnel: [_ _ _ _ _ _ _ _ _ _ _ _ _ _ _ _ _ _ _ _ _ TRUE _] -> w84
            tunnel: w83 -> [_ _ _ _ _ _ _ _ _ _ _ _ _ _ _ _ _ _ _ _ _ w880 _]
            tunnel: [_ _ _ _ _ _ _ _ _ _ _ _ _ _ _ _ _ _ _ _ _ w879 _] -> w82
            frame "Init", Default {
              w140 = FALSE ("RewCalib_Trig_L")
              w136 = u16 100 ("new element/subarray")
              # "Tdelay_R"
              # "Tdelay_L"
              # "RewCalib_N__R"
              # "RewCalib_N__L"
              # "Solenoid_Tcycle_R"
              # "Solenoid_Tcycle_L"
              # "Laser_Tcycle"
              # "Audio_Tcycle_R"
              # "Audio_Tcycle_L"
              # "initialize dataMTrig"
              n36 = call "myRIO_BRig_RT_dataMTrig_Solenoid_Tcycle__L.vi"() -> ("output_Solenoid_Tcycle__L"=w148:i32)  [unwired: 11 in]
              n37 = call "myRIO_BRig_RT_dataMTrig_Solenoid_Tcycle__R.vi"() -> ("output_Solenoid_Tcycle__R"=w149:i32)  [unwired: 11 in]
              n38 = call "myRIO_BRig_RT_dataMTrig_Audio_Tcycle__L.vi"() -> ("output_Audio_Tcycle__L"=w150:i32)  [unwired: 11 in]
              n39 = call "myRIO_BRig_RT_dataMTrig_Audio_Tcycle__R.vi"() -> ("output_Audio_Tcycle__R"=w151:i32)  [unwired: 11 in]
              n40 = call "myRIO_BRig_RT_dataMTrig_Laser_Tcycle.vi"() -> ("output_Laser_Tcycle"=w152:i32)  [unwired: 11 in]
              n41 = call "myRIO_BRig_RT_dataMTrig_Solenoid_RewCalib_nCycle__L.vi"() -> ("output_Solenoid_RewCalib_nCycle__L"=w144:i32)  [unwired: 11 in]
              n42 = call "myRIO_BRig_RT_dataMTrig_Solenoid_RewCalib_nCycle__R.vi"() -> ("output_Solenoid_RewCalib_nCycle__R"=w143:i32)  [unwired: 11 in]
              n43 = call "myRIO_BRig_RT_dataMTrig_Solenoid_Tdelay__L.vi"() -> ("output_Solenoid_Tdelay__L"=w142:i32)  [unwired: 11 in]
              n44 = call "myRIO_BRig_RT_dataMTrig_Solenoid_Tdelay__R.vi"() -> ("output_Solenoid_Tdelay__R"=w141:i32)  [unwired: 11 in]
              n45 = local read "MTrig_Solenoid_Tcycle__L"() -> (w153:u16)
              n46 = local read "MTrig_Solenoid_Tcycle__R"() -> (w154:u16)
              n47 = local read "MTrig_Laser_Tcycle"() -> (w137:u16)
              n48 = call "myRIO_BRig_RT_dataMTrig_init.vi"() -> ("output_dataMTrig"=w147:u16[])  [unwired: 5 in]
              n49 = local write "RewCalib_Trig_R"(w140) -> ()
              n50 = local write "RewCalib_Trig_L"(w140) -> ()
              n51 = local read "Tcycle_Cue_min"() -> (w138:u16)
              n52 = Replace Array Subset(array=w147, new element #1=w153, index #1=w148, new element #2=w154, index #2=w149, new element #3=w138, index #3=w150, new element #4=w138, index #4=w151, new element #5=w137, index #5=w152, new element #6=w136, index #6=w144, new element #7=w136, index #7=w143, new element #8=w136, index #8=w142, new element #9=w136, index #9=w141) -> (w146:u16[])
            }
            frame "UploadSettings_pre" {
              # "When the Host sends settings,\nnot all files send at the same time.\n\nIf RT reads the settings faster\nthan the Host can send them,\nthen we will skip settings.\n\nSolution:\nWait 20 cycles"
              n53 = Increment(x=w163) -> (x+1=w162:u16)
              n54 = Greater?(x=w162, y=u16 20) -> (0:w160:bool)
              n55 = Select(t=myRIO_BRig_RT__Case_NonExp_stateList."UploadSettings_Read_dataExp", s=w160, f=w159) -> (s? t:f=w157:T1)
            }
            frame "UploadSettings_Read_dataExp" {
              # "grab dataExp and\nstore it in the\ngeneric data array"
              # "dataExp"
              n56 = call "myRIO_BRig_RT_dataExp_init_details.vi"() -> ("output_dataSize"=w170:i32, "output_dataName"=w173:string)  [unwired: 10 in]
              n57 = call "myRIO_BRig_RT_comm_webdav_uploadReceived_check.vi"("input_dataName"=w173) -> ("output_Iexist"=w172:bool, "output_dataPath"=w171:path)  [unwired: 9 in]
              n58 = case shown="True" w172 {
                tunnel: w171 -> [_ w182]
                tunnel: w170 -> [_ w181]
                tunnel: [_ w180] -> w169
                tunnel: w166 -> [w175 w179]
                tunnel: [w175 w176] -> w165
                frame False {
                }
                frame True {
                  n59 = call "myRIO_BRig_RT_comm_webdav_uploadReceived_read.vi"("input_dataSize"=w181, "input_filePath"=w182) -> ("output_Ivalid"=w180:bool, "output_data"=w178:i64[])  [unwired: 8 in]
                  n60 = To Unsigned Word Integer(number=w178) -> (unsigned 16bit integer=w177:u16[])
                  n61 = Select(t=w177, s=w180, f=w179) -> (s? t:f=w176:u16[])
                }
              }
              n62 = Select(t=myRIO_BRig_RT__Case_NonExp_stateList."UploadSettings_dataExp_1", s=w169, f=myRIO_BRig_RT__Case_NonExp_stateList."UploadSettings_Read_dataLC" ("t")) -> (s? t:f=w164:T1)
            }
            frame "UploadSettings_Read_dataLC" {
              # "grab dataLC and\nstore it in the\ngeneric data array"
              # "dataLC"
              n63 = call "myRIO_BRig_RT_dataLC_init_details.vi"() -> ("output_dataSize"=w189:i32, "output_dataName"=w192:string)  [unwired: 10 in]
              n64 = call "myRIO_BRig_RT_comm_webdav_uploadReceived_check.vi"("input_dataName"=w192) -> ("output_Iexist"=w191:bool, "output_dataPath"=w190:path)  [unwired: 9 in]
              n65 = case shown="True" w191 {
                tunnel: w190 -> [_ w201]
                tunnel: w189 -> [_ w200]
                tunnel: [_ w199] -> w188
                tunnel: w185 -> [w194 w198]
                tunnel: [w194 w195] -> w184
                frame False {
                }
                frame True {
                  n66 = call "myRIO_BRig_RT_comm_webdav_uploadReceived_read.vi"("input_dataSize"=w200, "input_filePath"=w201) -> ("output_Ivalid"=w199:bool, "output_data"=w197:i64[])  [unwired: 8 in]
                  n67 = To Unsigned Word Integer(number=w197) -> (unsigned 16bit integer=w196:u16[])
                  n68 = Select(t=w196, s=w199, f=w198) -> (s? t:f=w195:u16[])
                }
              }
              n69 = Select(t=myRIO_BRig_RT__Case_NonExp_stateList."UploadSettings_dataLC_1", s=w188, f=myRIO_BRig_RT__Case_NonExp_stateList."UploadSettings_Read_dataMTrig" ("t")) -> (s? t:f=w183:T1)
            }
            frame "UploadSettings_Read_dataMTrig" {
              # "grab dataMTrig and\nstore it in the\ngeneric data array"
              # "dataMTrig"
              n70 = call "myRIO_BRig_RT_dataMTrig_init_details.vi"() -> ("output_dataSize"=w208:i32, "output_dataName"=w211:string)  [unwired: 10 in]
              n71 = call "myRIO_BRig_RT_comm_webdav_uploadReceived_check.vi"("input_dataName"=w211) -> ("output_Iexist"=w210:bool, "output_dataPath"=w209:path)  [unwired: 9 in]
              n72 = case shown="True" w210 {
                tunnel: w209 -> [_ w220]
                tunnel: w208 -> [_ w219]
                tunnel: [_ w218] -> w207
                tunnel: w204 -> [w213 w217]
                tunnel: [w213 w214] -> w203
                frame False {
                }
                frame True {
                  n73 = call "myRIO_BRig_RT_comm_webdav_uploadReceived_read.vi"("input_dataSize"=w219, "input_filePath"=w220) -> ("output_Ivalid"=w218:bool, "output_data"=w216:i64[])  [unwired: 8 in]
                  n74 = To Unsigned Word Integer(number=w216) -> (unsigned 16bit integer=w215:u16[])
                  n75 = Select(t=w215, s=w218, f=w217) -> (s? t:f=w214:u16[])
                }
              }
              n76 = Select(t=myRIO_BRig_RT__Case_NonExp_stateList."UploadSettings_dataMTrig_1", s=w207, f=myRIO_BRig_RT__Case_NonExp_stateList."Idle" ("t")) -> (s? t:f=w202:T1)
            }
            frame "UploadSettings_dataExp_1" {
              w229 = 100.0 ("y")
              # "Freq"
              # "f_millisec2count"
              # "laser"
              # "Cue_max"
              # "Cue_min"
              # "CuePenalty"
              # "Timeout"
              # "Wrong"
              # "Selection"
              # "RewardPost"
              # "Reward_R"
              # "Reward_L"
              # "Tcycle"
              # "TPB_min_R"
              # "TPB_min_L"
              # "TPB_max_R"
              # "TPB_max_L"
              # "I_trialUntilReward"
              # "ENL_penalty"
              # "ENL_min"
              # "ENL_max"
              # "BUR_max"
              # "BUR_min"
              # "CueCycles"
              # "Audio_Freq_R"
              # "Audio_Freq_L"
              # "Audio_Amp_R"
              # "Audio_Amp_L"
              n77 = call "myRIO_BRig_RT_dataExp_FPGA_f_count2ms.vi"() -> ("output_FPGA_f_count2ms"=w243:i32)  [unwired: 11 in]
              n78 = call "myRIO_BRig_RT_dataExp_laser1_Freq.vi"() -> ("output_laser1_Freq"=w242:i32)  [unwired: 11 in]
              n79 = call "myRIO_BRig_RT_dataExp_CueCycles.vi"() -> ("output_CueCycles"=w289:i32)  [unwired: 11 in]
              n80 = call "myRIO_BRig_RT_dataExp_Audio_amp__R.vi"() -> ("output_Audio_amp__R"=w293:i32)  [unwired: 11 in]
              n81 = call "myRIO_BRig_RT_dataExp_Audio_amp__L.vi"() -> ("output_Audio_amp__L"=w295:i32)  [unwired: 11 in]
              n82 = call "myRIO_BRig_RT_dataExp_Tcycle_Reward__L.vi"() -> ("output_Tcycle_Reward__L"=w266:i32)  [unwired: 11 in]
              n83 = call "myRIO_BRig_RT_dataExp_Tcycle_Reward__R.vi"() -> ("output_Tcycle_Reward__R"=w265:i32)  [unwired: 11 in]
              n84 = call "myRIO_BRig_RT_dataExp_Tcycle_RewardPost.vi"() -> ("output_Tcycle_RewardPost"=w264:i32)  [unwired: 11 in]
              n85 = call "myRIO_BRig_RT_dataExp_BUR_min.vi"() -> ("output_BUR_min"=w286:i32)  [unwired: 11 in]
              n86 = call "myRIO_BRig_RT_dataExp_ENL_min.vi"() -> ("output_ENL_min"=w282:i32)  [unwired: 11 in]
              n87 = call "myRIO_BRig_RT_dataExp_TPB_max__L.vi"() -> ("output_TPB_max__L"=w274:i32)  [unwired: 11 in]
              n88 = call "myRIO_BRig_RT_dataExp_TPB_max__R.vi"() -> ("output_TPB_max__R"=w273:i32)  [unwired: 11 in]
              n89 = call "myRIO_BRig_RT_dataExp_ENL_penalty.vi"() -> ("output_ENL_penalty"=w281:i32)  [unwired: 11 in]
              n90 = call "myRIO_BRig_RT_dataExp_laser1_Power_min.vi"() -> ("output_laser1_Power_min"=w241:i32)  [unwired: 11 in]
              n91 = call "myRIO_BRig_RT_dataExp_laser1_Tpeak.vi"() -> ("output_laser1_Tpeak"=w240:i32)  [unwired: 11 in]
              n92 = call "myRIO_BRig_RT_dataExp_Audio_freq__L.vi"() -> ("output_Audio_freq__L"=w291:i32)  [unwired: 11 in]
              n93 = call "myRIO_BRig_RT_dataExp_Audio_freq__R.vi"() -> ("output_Audio_freq__R"=w290:i32)  [unwired: 11 in]
              n94 = call "myRIO_BRig_RT_dataExp_BUR_max.vi"() -> ("output_BUR_max"=w287:i32)  [unwired: 11 in]
              n95 = call "myRIO_BRig_RT_dataExp_ENL_max.vi"() -> ("output_ENL_max"=w283:i32)  [unwired: 11 in]
              n96 = call "myRIO_BRig_RT_dataExp_ItrialUntilReward.vi"() -> ("output_I_trialUntilReward"=w277:i32)  [unwired: 11 in]
              n97 = call "myRIO_BRig_RT_dataExp_Tcycle_Selection.vi"() -> ("output_Tcycle_Selection"=w263:i32)  [unwired: 11 in]
              n98 = call "myRIO_BRig_RT_dataExp_Tcycle_Wrong.vi"() -> ("output_Tcycle_Wrong"=w262:i32)  [unwired: 11 in]
              n99 = call "myRIO_BRig_RT_dataExp_Tcycle_Timeout.vi"() -> ("output_Tcycle_Timeout"=w261:i32)  [unwired: 11 in]
              n100 = call "myRIO_BRig_RT_dataExp_TPB_min__L.vi"() -> ("output_TPB_min__L"=w272:i32)  [unwired: 11 in]
              n101 = call "myRIO_BRig_RT_dataExp_TPB_min__R.vi"() -> ("output_TPB_min__R"=w271:i32)  [unwired: 11 in]
              n102 = call "myRIO_BRig_RT_dataExp_laser1_Tshutter.vi"() -> ("output_laser1_Tshutter"=w239:i32)  [unwired: 11 in]
              n103 = call "myRIO_BRig_RT_dataExp_laser1_duration.vi"() -> ("output_laser1_duration"=w238:i32)  [unwired: 11 in]
              n104 = call "myRIO_BRig_RT_dataExp_Tcycle_CuePenalty.vi"() -> ("output_Tcycle_CuePenalty"=w254:i32)  [unwired: 11 in]
              n105 = call "myRIO_BRig_RT_dataExp_Tcycle_Cue_min.vi"() -> ("output_Tcycle_Cue_min"=w253:i32)  [unwired: 11 in]
              n106 = call "myRIO_BRig_RT_dataExp_Tcycle_Cue_max.vi"() -> ("output_Tcycle_Cue_max"=w252:i32)  [unwired: 11 in]
              n107 = Index Array(array=w246, index #1=w295, index #2=w293, index #3=w291, index #4=w290, index #5=w289, index #6=w287, index #7=w286, index #8=w283, index #9=w282, index #10=w281, index #11=w277, index #12=w274, index #13=w273, index #14=w272, index #15=w271, index #16=w266, index #17=w265, index #18=w264, index #19=w263, index #20=w262, index #21=w261, index #22=w254, index #23=w253, index #24=w252, index #25=w243, index #26=w242, index #27=w241, index #28=w240, index #29=w239, index #30=w238) -> (element #1=w294:u16, element #2=w292:u16, element #3=w249:u16, element #4=w248:u16, element #5=w288:u16, element #6=w285:u16, element #7=w284:u16, element #8=w280:u16, element #9=w279:u16, element #10=w278:u16, element #11=w275:u16, element #12=w270:u16, element #13=w269:u16, element #14=w268:u16, element #15=w267:u16, element #16=w260:u16, element #17=w259:u16, element #18=w258:u16, element #19=w257:u16, element #20=w256:u16, element #21=w255:u16, element #22=w251:u16, element #23=w245:u16, element #24=w244:u16, element #25=w237:u16, element #26=w228:u16, element #27=w227:u16, element #28=w226:u16, element #29=w225:u16, element #30=w221:u16)
              n108 = To Double Precision Float(number=w237) -> (double precision float=w236:dbl)
              n109 = To Double Precision Float(number=w228) -> (double precision float=w234:dbl)
              n110 = To Double Precision Float(number=w227) -> (double precision float=w232:dbl)
              n111 = To Double Precision Float(number=w226) -> (double precision float=w231:dbl)
              n112 = To Double Precision Float(number=w225) -> (double precision float=w230:dbl)
              n113 = local write "Tcycle_Selection"(w257) -> ()
              n114 = local write "Tcycle_Wrong"(w256) -> ()
              n115 = local write "Tcycle_Timeout"(w255) -> ()
              n116 = local write "Audio_Amp__L"(w294) -> ()
              n117 = local write "Audio_Amp__R"(w292) -> ()
              n118 = Divide(x=w236, y=w229) -> (x/y=w235:dbl)
              n119 = Divide(x=w234, y=w229) -> (x/y=w233:dbl)
              n120 = Divide(x=w232, y=w229) -> (x/y=w224:dbl)
              n121 = Divide(x=w231, y=w229) -> (x/y=w223:dbl)
              n122 = Divide(x=w230, y=w229) -> (x/y=w222:dbl)
              n123 = local write "Tcycle_ENLPenalty"(w278) -> ()
              n124 = local write "Tcycle_ENL_max"(w280) -> ()
              n125 = local write "laser_duration"(w221) -> ()
              n126 = local write "TpB_Min_L"(w268) -> ()
              n127 = local write "TpB_Min_R"(w267) -> ()
              n128 = local write "laser_power_min"(w224) -> ()
              n129 = local write "f_millisec2count"(w235) -> ()
              n130 = local write "laser_Tshutter"(w222) -> ()
              n131 = local write "laser_Tpeak"(w223) -> ()
              n132 = local write "laser_Freq"(w233) -> ()
              n133 = local write "Tcycle_CuePenalty"(w251) -> ()
              n134 = local write "Tcycle_Cue_min"(w245) -> ()
              n135 = local write "Tcycle_Cue_max"(w244) -> ()
              n136 = To Unsigned Byte Integer(number=w249) -> (unsigned 8bit integer=w250:u8)
              n137 = To Unsigned Byte Integer(number=w248) -> (unsigned 8bit integer=w247:u8)
              n138 = Not Equal To 0?(x=w275) -> (x != 0?=w276:bool)
              n139 = local write "Tcycle_Reward_L"(w260) -> ()
              n140 = local write "Tcycle_Reward_R"(w259) -> ()
              n141 = local write "Tcycle_RewardPost"(w258) -> ()
              n142 = local write "CueCycles"(w288) -> ()
              n143 = local write "BUR_min"(w284) -> ()
              n144 = local write "BUR_max"(w285) -> ()
              n145 = local write "Tcycle_ENL_min"(w279) -> ()
              n146 = local write "TpB_Max_L"(w270) -> ()
              n147 = local write "TpB_Max_R"(w269) -> ()
              n148 = local write "TrialUntilReward"(w276) -> ()
              n149 = local write "Audio_Freq__L"(w250) -> ()
              n150 = local write "Audio_Freq__R"(w247) -> ()
            }
            frame "UploadSettings_dataLC_1" {
              # "Cue1_All_delayOpt"
              # "ENL1_All_delayOpt"
              # "Cue1_First_delayOpt"
              # "ENL1_First_delayOpt"
              # "ENL1 First"
              # "Cue1 All"
              # "Cue1 First"
              # "Count"
              # "Tdelay"
              # "Prob"
              # "OnOff"
              # "Block"
              # "ENL1 All"
              # "Count"
              # "Tdelay"
              # "Prob"
              # "OnOff"
              # "Block"
              # "Count"
              # "Tdelay"
              # "Prob"
              # "Block"
              # "OnOff"
              # "Count"
              # "Tdelay"
              # "Prob"
              # "OnOff"
              # "Block"
              n151 = call "myRIO_BRig_RT_dataLC_Cue1_First_Block.vi"() -> ("output_Cue1_First_Block"=w354:i32)  [unwired: 11 in]
              n152 = call "myRIO_BRig_RT_dataLC_Cue1_First_OnOff.vi"() -> ("output_Cue1_First_OnOff"=w352:i32)  [unwired: 11 in]
              n153 = call "myRIO_BRig_RT_dataLC_Cue1_First_Count.vi"() -> ("output_Cue1_First_Count"=w349:i32)  [unwired: 11 in]
              n154 = call "myRIO_BRig_RT_dataLC_Cue1_l1_All_Block.vi"() -> ("output_Cue1_l1_All_Block"=w336:i32)  [unwired: 11 in]
              n155 = call "myRIO_BRig_RT_dataLC_Cue1_All_OnOff.vi"() -> ("output_Cue1_All_OnOff"=w335:i32)  [unwired: 11 in]
              n156 = call "myRIO_BRig_RT_dataLC_Cue1_l1_All_Count.vi"() -> ("output_Cue1_All_Count"=w346:i32)  [unwired: 11 in]
              n157 = call "myRIO_BRig_RT_dataLC_ENL1_First_Block.vi"() -> ("output_ENL1_First_Block"=w334:i32)  [unwired: 11 in]
              n158 = call "myRIO_BRig_RT_dataLC_ENL1_First_OnOff.vi"() -> ("output_ENL1_First_OnOff"=w345:i32)  [unwired: 11 in]
              n159 = call "myRIO_BRig_RT_dataLC_ENL1_First_Count.vi"() -> ("output_ENL1_First_Count"=w342:i32)  [unwired: 11 in]
              n160 = call "myRIO_BRig_RT_dataLC_ENL1_All_Block.vi"() -> ("output_ENL1_All_Block"=w341:i32)  [unwired: 11 in]
              n161 = call "myRIO_BRig_RT_dataLC_ENL1_All_OnOff.vi"() -> ("output_ENL1_All_OnOff"=w340:i32)  [unwired: 11 in]
              n162 = call "myRIO_BRig_RT_dataLC_ENL1_All_Count.vi"() -> ("output_ENL1_All_Count"=w337:i32)  [unwired: 11 in]
              n163 = call "myRIO_BRig_RT_dataLC_ENL1_First_delayOpt.vi"() -> ("output_ENL1_First_delayOpt"=w311:i32)  [unwired: 11 in]
              n164 = call "myRIO_BRig_RT_dataLC_Cue1_First_delayOpt.vi"() -> ("output_Cue1_First_delayOpt"=w310:i32)  [unwired: 11 in]
              n165 = call "myRIO_BRig_RT_dataLC_ENL1_All_delayOpt.vi"() -> ("output_ENL1_All_delayOpt"=w303:i32)  [unwired: 11 in]
              n166 = call "myRIO_BRig_RT_dataLC_Cue1_All_delayOpt.vi"() -> ("output_Cue1_All_delayOpt"=w302:i32)  [unwired: 11 in]
              n167 = call "myRIO_BRig_RT_dataLC_Cue1_First_Probability.vi"() -> ("output_Cue1_First_Probability"=w351:i32)  [unwired: 11 in]
              n168 = call "myRIO_BRig_RT_dataLC_Cue1_First_Tdelay.vi"() -> ("output_Cue1_First_Tdelay"=w350:i32)  [unwired: 11 in]
              n169 = call "myRIO_BRig_RT_dataLC_Cue1_All_Probability.vi"() -> ("output_Cue1_All_Probability"=w348:i32)  [unwired: 11 in]
              n170 = call "myRIO_BRig_RT_dataLC_Cue1_All_Tdelay.vi"() -> ("output_Cue1_All_Tdelay"=w347:i32)  [unwired: 11 in]
              n171 = call "myRIO_BRig_RT_dataLC_ENL1_First_Probability.vi"() -> ("output_ENL1_First_Probability"=w344:i32)  [unwired: 11 in]
              n172 = call "myRIO_BRig_RT_dataLC_ENL1_First_Tdelay.vi"() -> ("output_ENL1_First_Tdelay"=w343:i32)  [unwired: 11 in]
              n173 = call "myRIO_BRig_RT_dataLC_ENL1_All_Probability.vi"() -> ("output_ENL1_All_Probability"=w339:i32)  [unwired: 11 in]
              n174 = call "myRIO_BRig_RT_dataLC_ENL1_All_Tdelay.vi"() -> ("output_ENL1_All_Tdelay"=w338:i32)  [unwired: 11 in]
              n175 = Index Array(array=w312, index #1=w354, index #2=w352, index #3=w351, index #4=w350, index #5=w349, index #6=w336, index #7=w335, index #8=w348, index #9=w347, index #10=w346, index #11=w334, index #12=w345, index #13=w344, index #14=w343, index #15=w342, index #16=w341, index #17=w340, index #18=w339, index #19=w338, index #20=w337, index #21=w311, index #22=w310, index #23=w303, index #24=w302) -> (element #1=w353:u16, element #2=w332:u16, element #3=w331:u16, element #4=w330:u16, element #5=w329:u16, element #6=w325:u16, element #7=w324:u16, element #8=w323:u16, element #9=w322:u16, element #10=w321:u16, element #11=w320:u16, element #12=w319:u16, element #13=w318:u16, element #14=w317:u16, element #15=w304:u16, element #16=w316:u16, element #17=w315:u16, element #18=w314:u16, element #19=w313:u16, element #20=w305:u16, element #21=w308:u16, element #22=w306:u16, element #23=w299:u16, element #24=w298:u16)
              n176 = Not Equal To 0?(x=w299) -> (x != 0?=w301:bool)
              n177 = Not Equal To 0?(x=w298) -> (x != 0?=w300:bool)
              n178 = Not Equal To 0?(x=w308) -> (x != 0?=w309:bool)
              n179 = Not Equal To 0?(x=w306) -> (x != 0?=w307:bool)
              n180 = Not Equal To 0?(x=w332) -> (x != 0?=w333:bool)
              n181 = Not Equal To 0?(x=w324) -> (x != 0?=w328:bool)
              n182 = Not Equal To 0?(x=w319) -> (x != 0?=w327:bool)
              n183 = Not Equal To 0?(x=w315) -> (x != 0?=w326:bool)
              n184 = local write "LC_Cue1_First_Probability"(w331) -> ()
              n185 = local write "LC_ENL1_First_Probability"(w318) -> ()
              n186 = local write "LC_ENL1_First_delayOpt"(w309) -> ()
              n187 = local write "LC_Cue1_First_delayOpt"(w307) -> ()
              n188 = local write "LC_ENL1_All_delayOpt"(w301) -> ()
              n189 = local write "LC_Cue1_All_delayOpt"(w300) -> ()
              n190 = local write "LC_Cue1_All_Probability"(w323) -> ()
              n191 = local write "LC_Cue1_First_Tdelay"(w330) -> ()
              n192 = local write "LC_ENL1_All_Probability"(w314) -> ()
              n193 = local write "LC_Cue1_First_OnOff"(w333) -> ()
              n194 = local write "LC_Cue1_First_Count"(w329) -> ()
              n195 = local write "LC_Cue1_First_Block"(w353) -> ()
              n196 = local write "LC_ENL1_First_Tdelay"(w317) -> ()
              n197 = local write "LC_ENL1_First_OnOff"(w327) -> ()
              n198 = local write "LC_ENL1_First_Count"(w304) -> ()
              n199 = local write "LC_ENL1_First_Block"(w320) -> ()
              n200 = local write "LC_Cue1_All_Tdelay"(w322) -> ()
              n201 = local write "LC_Cue1_All_OnOff"(w328) -> ()
              n202 = local write "LC_Cue1_All_Count"(w321) -> ()
              n203 = local write "LC_Cue1_All_Block"(w325) -> ()
              n204 = local write "LC_ENL1_All_Tdelay"(w313) -> ()
              n205 = local write "LC_ENL1_All_OnOff"(w326) -> ()
              n206 = local write "LC_ENL1_All_Count"(w305) -> ()
              n207 = local write "LC_ENL1_All_Block"(w316) -> ()
            }
            frame "UploadSettings_dataLC_2" {
              # "Wrong"
              # "Reward"
              # "Trial"
              # "Tdelay"
              # "Prob"
              # "Block"
              # "OnOff"
              # "Trial"
              # "Tdelay"
              # "Prob"
              # "OnOff"
              # "Block"
              n208 = call "myRIO_BRig_RT_dataLC_Reward_Block.vi"() -> ("output_Reward_Block"=w379:i32)  [unwired: 11 in]
              n209 = call "myRIO_BRig_RT_dataLC_Reward_OnOff.vi"() -> ("output_Reward_OnOff"=w377:i32)  [unwired: 11 in]
              n210 = call "myRIO_BRig_RT_dataLC_Reward_Trial.vi"() -> ("output_Reward_Trial"=w374:i32)  [unwired: 11 in]
              n211 = call "myRIO_BRig_RT_dataLC_Wrong_Block.vi"() -> ("output_Wrong_Block"=w370:i32)  [unwired: 11 in]
              n212 = call "myRIO_BRig_RT_dataLC_Wrong_OnOff.vi"() -> ("output_Wrong_OnOff"=w369:i32)  [unwired: 11 in]
              n213 = call "myRIO_BRig_RT_dataLC_Wrong_Trial.vi"() -> ("output_Wrong_Trial"=w371:i32)  [unwired: 11 in]
              n214 = call "myRIO_BRig_RT_dataLC_Reward_Probability.vi"() -> ("output_Reward_Probability"=w376:i32)  [unwired: 11 in]
              n215 = call "myRIO_BRig_RT_dataLC_Reward_Tdelay.vi"() -> ("output_Reward_Tdelay"=w375:i32)  [unwired: 11 in]
              n216 = call "myRIO_BRig_RT_dataLC_Wrong_Probability.vi"() -> ("output_Wrong_Probability"=w373:i32)  [unwired: 11 in]
              n217 = call "myRIO_BRig_RT_dataLC_Wrong_Tdelay.vi"() -> ("output_Wrong_Tdelay"=w372:i32)  [unwired: 11 in]
              n218 = Index Array(array=w357, index #1=w379, index #2=w377, index #3=w376, index #4=w375, index #5=w374, index #6=w370, index #7=w369, index #8=w373, index #9=w372, index #10=w371) -> (element #1=w378:u16, element #2=w367:u16, element #3=w366:u16, element #4=w365:u16, element #5=w364:u16, element #6=w362:u16, element #7=w361:u16, element #8=w360:u16, element #9=w359:u16, element #10=w358:u16)
              n219 = Not Equal To 0?(x=w367) -> (x != 0?=w368:bool)
              n220 = Not Equal To 0?(x=w361) -> (x != 0?=w363:bool)
              n221 = local write "LC_Reward_Probability"(w366) -> ()
              n222 = local write "LC_Wrong_Probability"(w360) -> ()
              n223 = local write "LC_Reward_Tdelay"(w365) -> ()
              n224 = local write "LC_Reward_OnOff"(w368) -> ()
              n225 = local write "LC_Reward_Block"(w378) -> ()
              n226 = local write "LC_Reward_Trial"(w364) -> ()
              n227 = local write "LC_Wrong_Tdelay"(w359) -> ()
              n228 = local write "LC_Wrong_OnOff"(w363) -> ()
              n229 = local write "LC_Wrong_Block"(w362) -> ()
              n230 = local write "LC_Wrong_Trial"(w358) -> ()
            }
            frame "UploadSettings_dataMTrig_1" {
              # "Tdelay_R"
              # "Tdelay_L"
              # "Tcycle_R"
              # "Tcycle_L"
              # "RewCalib_nCycle_R"
              # "RewCalib_nCycle_L"
              # "Solenoid"
              # "Laser_Tcycle"
              n231 = call "myRIO_BRig_RT_dataMTrig_Laser_Tcycle.vi"() -> ("output_Laser_Tcycle"=w389:i32)  [unwired: 11 in]
              n232 = call "myRIO_BRig_RT_dataMTrig_Solenoid_RewCalib_nCycle__L.vi"() -> ("output_Solenoid_RewCalib_nCycle__L"=w388:i32)  [unwired: 11 in]
              n233 = call "myRIO_BRig_RT_dataMTrig_Solenoid_RewCalib_nCycle__R.vi"() -> ("output_Solenoid_RewCalib_nCycle__R"=w387:i32)  [unwired: 11 in]
              n234 = call "myRIO_BRig_RT_dataMTrig_Solenoid_Tdelay__L.vi"() -> ("output_Solenoid_Tdelay__L"=w384:i32)  [unwired: 11 in]
              n235 = call "myRIO_BRig_RT_dataMTrig_Solenoid_Tdelay__R.vi"() -> ("output_Solenoid_Tdelay__R"=w383:i32)  [unwired: 11 in]
              n236 = call "myRIO_BRig_RT_dataMTrig_Solenoid_Tcycle__L.vi"() -> ("output_Solenoid_Tcycle__L"=w386:i32)  [unwired: 11 in]
              n237 = call "myRIO_BRig_RT_dataMTrig_Solenoid_Tcycle__R.vi"() -> ("output_Solenoid_Tcycle__R"=w385:i32)  [unwired: 11 in]
              n238 = Index Array(array=w382, index #1=w389, index #2=w388, index #3=w387, index #4=w386, index #5=w385, index #6=w384, index #7=w383) -> (element #1=w396:u16, element #2=w395:u16, element #3=w394:u16, element #4=w393:u16, element #5=w392:u16, element #6=w391:u16, element #7=w390:u16)
              n239 = Replace Array Subset(array=w398, new element #1=w396, index #1=w389, new element #2=w395, index #2=w388, new element #3=w394, index #3=w387, new element #4=w393, index #4=w386, new element #5=w392, index #5=w385, new element #6=w391, index #6=w384, new element #7=w390, index #7=w383) -> (w397:u16[])
              n240 = local write "MTrig_Solenoid_Tcycle__L"(w393) -> ()
              n241 = local write "MTrig_Solenoid_Tcycle__R"(w392) -> ()
              n242 = local write "MTrig_Laser_Tcycle"(w396) -> ()
            }
            frame "Idle" {
              # "To ensure timing, we split the\nidle state into 4 phases"
              # "Laser_Tcycle"
              # "Audio_Tcycle_R"
              # "Audio_Tcycle_L"
              n243 = local read "laser_power_min"() -> (w401:dbl)
              n244 = local read "f_millisec2count"() -> (w409:dbl)
              n245 = local read "Audio_Amp__R"() -> (w403:u16)
              n246 = local read "Audio_Amp__L"() -> (w405:u16)
              n247 = local read "Audio_Freq__R"() -> (w402:u8)
              n248 = local read "Audio_Freq__L"() -> (w404:u8)
              n249 = local read "MTrig_Audio_trig__L"() -> (w417:bool)
              n250 = local read "MTrig_Audio_trig__R"() -> (w419:bool)
              n251 = Select(t=myRIO_BRig_RT__Case_NonExp_stateList."SendData" ("Enum"), s="SendData", f=myRIO_BRig_RT__Case_NonExp_stateList."Idle_2" ("Enum")) -> (s? t:f=w412:T1)
              n252 = call "myRIO__convert__Voltage_to_FPGAvalue.vi"("input_voltage"=w401) -> ("output_PortC"=w400:i16)  [unwired: 9 in, 1 out]
              n253 = local read "MTrig_Laser_trig"() -> (w418:bool)
              n254 = To Unsigned Word Integer(number=w409) -> (unsigned 16bit integer=w408:u16)
              n255 = call "myRIO_BRig_RT_dataMTrig_Audio_Tcycle__L.vi"() -> ("output_Audio_Tcycle__L"=w428:i32)  [unwired: 11 in]
              n256 = call "myRIO_BRig_RT_dataMTrig_Audio_Tcycle__R.vi"() -> ("output_Audio_Tcycle__R"=w427:i32)  [unwired: 11 in]
              n257 = call "myRIO_BRig_RT_dataMTrig_Laser_Tcycle.vi"() -> ("output_Laser_Tcycle"=w426:i32)  [unwired: 11 in]
              n258 = local read "MTrig_Laser_Tcycle"() -> (w410:u16)
              n259 = xnode "Read/Write Control"("FPGA VI Reference In"=w407, "error in"=w406, "k1__counter_per_ms"=w408, "audioAmp_L"=w405, "audioFreq_L_kHz"=w404, "audioAmp_R"=w403, "audioFreq_R_kHz"=w402, "AnaOut_0"=w400) -> ()  [unwired: 2 out]
              n260 = Select(t=myRIO_BRig_RT__Case_NonExp_stateList."TestConnection" ("Enum"), s="TestConnection", f=w412) -> (s? t:f=w421:T1)
              n261 = local read "Tcycle_Cue_min"() -> (w411:u16)
              n262 = Compound Arithmetic op=OR(w417, w419, w418) -> (w420:bool)
              n263 = case shown="True" w420 {
                frame False {
                }
                frame True {
                  w429 = FALSE
                  n264 = local write "MTrig_Audio_trig__L"(w429) -> ()
                  n265 = local write "MTrig_Audio_trig__R"(w429) -> ()
                  n266 = local write "MTrig_Laser_trig"(w429) -> ()
                }
              }
              n267 = Replace Array Subset(array=w424, new element #1=w411, index #1=w428, new element #2=w411, index #2=w427, new element #3=w410, index #3=w426) -> (w425:u16[])
            }
            frame "Idle_2" {
              w431 = u16 0 ("t")
              # "To ensure timing, we split the\nidle state into 4 phases"
              # "Ncycles"
              # "Ncycles"
              # "RewCalib"
              # "RewCalib"
              # "Solenoid R"
              # "Solenoid L"
              n268 = call "myRIO_BRig_RT_dataMTrig_Solenoid_RewCalib_OnOff__L.vi"() -> ("output_Solenoid_RewCalib_OnOff__L"=w462:i32)  [unwired: 11 in]
              n269 = call "myRIO_BRig_RT_dataMTrig_Solenoid_N__L.vi"() -> ("output_Solenoid_N__L"=w450:i32)  [unwired: 11 in]
              n270 = call "myRIO_BRig_RT_dataMTrig_Solenoid_RewCalib_OnOff__R.vi"() -> ("output_Solenoid_RewCalib_OnOff__R"=w447:i32)  [unwired: 11 in]
              n271 = call "myRIO_BRig_RT_dataMTrig_Solenoid_N__R.vi"() -> ("output_Solenoid_N__R"=w446:i32)  [unwired: 11 in]
              n272 = Index Array(array=w453, index #1=w462, index #2=w450, index #3=w447, index #4=w446) -> (element #1=w449:u16, element #2=w444:u16, element #3=w445:u16, element #4=w443:u16)
              n273 = local read "RewCalib_Trig_L"() -> (w442:bool)
              n274 = local read "RewCalib_Trig_R"() -> (w441:bool)
              n275 = Equal To 0?(x=w444) -> (x = 0?=w452:bool)
              n276 = Equal To 0?(x=w443) -> (x = 0?=w451:bool)
              n277 = Not Equal To 0?(x=w445) -> (x != 0?=w463:bool)
              n278 = Not Equal To 0?(x=w449) -> (x != 0?=w464:bool)
              n279 = And(x=w452, y=w451) -> (x .and. y?=w456:bool)
              n280 = Or(x=w442, y=w441) -> (x .or. y?=w457:bool)
              n281 = Not Exclusive Or(1:w464, 2:w442) -> (0:w459:bool)
              n282 = Not Exclusive Or(1:w463, 2:w441) -> (0:w461:bool)
              n283 = And(x=w457, y=w456) -> (x .and. y?=w439:bool)
              n284 = Not(x=w459) -> (.not. x?=w458:bool)
              n285 = Not(x=w461) -> (.not. x?=w460:bool)
              n286 = Or(x=w458, y=w460) -> (x .or. y?=w440:bool)
              n287 = Or(x=w439, y=w440) -> (x .or. y?=w455:bool)
              n288 = local read "count_warmup_R"() -> (w430:u16)
              n289 = local read "count_warmup_L"() -> (w435:u16)
              n290 = Select(t=myRIO_BRig_RT__Case_NonExp_stateList."RewardCalibration_pre" ("Enum"), s=w455, f=myRIO_BRig_RT__Case_NonExp_stateList."Idle_3" ("Enum")) -> (s? t:f=w438:T1)
              n291 = Select(t=w431, s="count_warmup_L_reset", f=w435) -> (s? t:f=→"count_warmup_L":u16)
              n292 = Select(t=w431, s="count_warmup_R_reset", f=w430) -> (s? t:f=→"count_warmup_R":u16)
            }
            frame "Idle_3" {
              w487 = u8 0 ("f")
              # "To ensure timing, we split the\nidle state into 4 phases"
              n293 = local read "MTrig_Solenoid_trig__L"() -> (w478:bool)
              n294 = local read "MTrig_Solenoid_trig__R"() -> (w488:bool)
              n295 = local read "warmupType"() -> (w470:u8)
              n296 = local read "warmup"() -> (w480:bool)
              n297 = Not Equal To 0?(x=w470) -> (x != 0?=w469:bool)
              n298 = Not(x=w469) -> (.not. x?=w481:bool)
              n299 = Select(t=u8 1, s=w478, f=w487) -> (s? t:f=w486:u8)
              n300 = Select(t=u8 2, s=w488, f=w487) -> (s? t:f=w485:u8)
              n301 = And(x=w480, y=w481) -> (x .and. y?=w479:bool)
              n302 = And(x=w480, y=w469) -> (x .and. y?=w474:bool)
              n303 = Add(x=w486, y=w485) -> (x+y=w484:u8)
              n304 = case shown="3" w484 {
                tunnel: w483 -> [w491 w495 w513 w531]
                tunnel: [w491 w494 w512 w530] -> w482
                tunnel: w479 -> [_ w493 w511 w529]
                tunnel: [_ TRUE TRUE TRUE] -> w476
                frame 0, Default {
                }
                frame 1 {
                  n305 = case shown="True" w493 {
                    tunnel: w495 -> [w504 w509]
                    tunnel: [w503 w508] -> w494
                    frame True {
                      # "Audio_L"
                      # "Solenoid_L"
                      n306 = call "myRIO_BRig_RT_dataMTrig_Solenoid_N__L.vi"() -> ("output_Solenoid_N__L"=w500:i32)  [unwired: 11 in]
                      n307 = call "myRIO_BRig_RT_dataMTrig_Audio_N__L.vi"() -> ("output_Audio_N__L"=w498:i32)  [unwired: 11 in]
                      n308 = Index Array(array=w504, index #1=w500, index #2=w498) -> (element #1=w502:u16, element #2=w501:u16)
                      n309 = Increment(x=w502) -> (x+1=w499:u16)
                      n310 = Increment(x=w501) -> (x+1=w497:u16)
                      n311 = Replace Array Subset(array=w504, new element #1=w499, index #1=w500, new element #2=w497, index #2=w498) -> (w503:u16[])
                    }
                    frame False {
                      # "Solenoid_L"
                      n312 = call "myRIO_BRig_RT_dataMTrig_Solenoid_N__L.vi"() -> ("output_Solenoid_N__L"=w506:i32)  [unwired: 11 in]
                      n313 = Index Array(array=w509, index=w506) -> (element=w507:u16)
                      n314 = Increment(x=w507) -> (x+1=w505:u16)
                      n315 = Replace Array Subset(array=w509, new element=w505, index=w506) -> (w508:u16[])
                    }
                  }
                  n316 = local write "MTrig_Solenoid_trig__L"(FALSE) -> ()
                }
                frame 2 {
                  n317 = case shown="True" w511 {
                    tunnel: w513 -> [w522 w527]
                    tunnel: [w521 w526] -> w512
                    frame True {
                      # "Audio_R"
                      # "Solenoid_R"
                      n318 = call "myRIO_BRig_RT_dataMTrig_Solenoid_N__R.vi"() -> ("output_Solenoid_N__R"=w518:i32)  [unwired: 11 in]
                      n319 = call "myRIO_BRig_RT_dataMTrig_Audio_N__R.vi"() -> ("output_Audio_N__R"=w517:i32)  [unwired: 11 in]
                      n320 = Index Array(array=w522, index #1=w518, index #2=w517) -> (element #1=w520:u16, element #2=w519:u16)
                      n321 = Increment(x=w519) -> (x+1=w515:u16)
                      n322 = Increment(x=w520) -> (x+1=w516:u16)
                      n323 = Replace Array Subset(array=w522, new element #1=w516, index #1=w518, new element #2=w515, index #2=w517) -> (w521:u16[])
                    }
                    frame False {
                      # "Solenoid_R"
                      n324 = call "myRIO_BRig_RT_dataMTrig_Solenoid_N__R.vi"() -> ("output_Solenoid_N__R"=w523:i32)  [unwired: 11 in]
                      n325 = Index Array(array=w527, index=w523) -> (element=w525:u16)
                      n326 = Increment(x=w525) -> (x+1=w524:u16)
                      n327 = Replace Array Subset(array=w527, new element=w524, index=w523) -> (w526:u16[])
                    }
                  }
                  n328 = local write "MTrig_Solenoid_trig__R"(FALSE) -> ()
                }
                frame 3 {
                  w532 = FALSE
                  n329 = case shown="True" w529 {
                    tunnel: w531 -> [w546 w554]
                    tunnel: [w545 w553] -> w530
                    frame True {
                      # "Audio_R"
                      # "Solenoid_R"
                      # "Audio_L"
                      # "Solenoid_L"
                      n330 = call "myRIO_BRig_RT_dataMTrig_Solenoid_N__L.vi"() -> ("output_Solenoid_N__L"=w540:i32)  [unwired: 11 in]
                      n331 = call "myRIO_BRig_RT_dataMTrig_Audio_N__L.vi"() -> ("output_Audio_N__L"=w538:i32)  [unwired: 11 in]
                      n332 = call "myRIO_BRig_RT_dataMTrig_Solenoid_N__R.vi"() -> ("output_Solenoid_N__R"=w536:i32)  [unwired: 11 in]
                      n333 = call "myRIO_BRig_RT_dataMTrig_Audio_N__R.vi"() -> ("output_Audio_N__R"=w535:i32)  [unwired: 11 in]
                      n334 = Index Array(array=w546, index #1=w540, index #2=w538, index #3=w536, index #4=w535) -> (element #1=w544:u16, element #2=w543:u16, element #3=w542:u16, element #4=w541:u16)
                      n335 = Increment(x=w541) -> (x+1=w533:u16)
                      n336 = Increment(x=w544) -> (x+1=w539:u16)
                      n337 = Increment(x=w543) -> (x+1=w537:u16)
                      n338 = Increment(x=w542) -> (x+1=w534:u16)
                      n339 = Replace Array Subset(array=w546, new element #1=w539, index #1=w540, new element #2=w537, index #2=w538, new element #3=w534, index #3=w536, new element #4=w533, index #4=w535) -> (w545:u16[])
                    }
                    frame False {
                      # "Solenoid_R"
                      # "Solenoid_L"
                      n340 = call "myRIO_BRig_RT_dataMTrig_Solenoid_N__L.vi"() -> ("output_Solenoid_N__L"=w550:i32)  [unwired: 11 in]
                      n341 = call "myRIO_BRig_RT_dataMTrig_Solenoid_N__R.vi"() -> ("output_Solenoid_N__R"=w547:i32)  [unwired: 11 in]
                      n342 = Index Array(array=w554, index #1=w550, index #2=w547) -> (element #1=w552:u16, element #2=w551:u16)
                      n343 = Increment(x=w552) -> (x+1=w549:u16)
                      n344 = Increment(x=w551) -> (x+1=w548:u16)
                      n345 = Replace Array Subset(array=w554, new element #1=w549, index #1=w550, new element #2=w548, index #2=w547) -> (w553:u16[])
                    }
                  }
                  n346 = local write "MTrig_Solenoid_trig__L"(w532) -> ()
                  n347 = local write "MTrig_Solenoid_trig__R"(w532) -> ()
                }
              }
              n348 = local read "get_countPerMS"() -> (w468:bool)
              n349 = Select(t=myRIO_BRig_RT__Case_NonExp_stateList."Get_FPGA_count_per_ms" ("Enum"), s=w468, f=myRIO_BRig_RT__Case_NonExp_stateList."Idle_4" ("Enum")) -> (s? t:f=w466:T1)
              n350 = Select(t=myRIO_BRig_RT__Case_NonExp_stateList."Cue_pre", s=w474, f=myRIO_BRig_RT__Case_NonExp_stateList."DispenseWater_pre" ("Enum")) -> (s? t:f=w472:T1)
              n351 = Select(t=w472, s=w476, f=w466) -> (s? t:f=w477:T1)
            }
            frame "Idle_4" {
              # "use dataMTrig as it is one of the last to transfer"
              # "To ensure timing, we split the\nidle state into 4 phases"
              n352 = call "myRIO_BRig_RT_comm_webdav_uploadReceived_check_v2,0.vi"("input_dataName"="dataMTrig") -> ("output_Iexist"=w560:bool)  [unwired: 9 in, 1 out]
              n353 = Select(t=myRIO_BRig_RT__Case_NonExp_stateList."UploadSettings_pre" ("Enum"), s=w560, f=myRIO_BRig_RT__Case_NonExp_stateList."Idle") -> (s? t:f=w558:T1)
            }
            frame "Cue_pre" {
              w570 = u16 1 ("t")
              w569 = u16 0 ("new element/subarray")
              w566 = u16 0 ("new element/subarray")
              # "Ncycle"
              # "count"
              # "Audio_R"
              # "Solenoid_R"
              # "Solenoid_L"
              # "Ncycle"
              # "count"
              # "Audio_L"
              n354 = call "myRIO_BRig_RT_dataMTrig_Solenoid_N__L.vi"() -> ("output_Solenoid_N__L"=w579:i32)  [unwired: 11 in]
              n355 = call "myRIO_BRig_RT_dataMTrig_Solenoid_N__R.vi"() -> ("output_Solenoid_N__R"=w578:i32)  [unwired: 11 in]
              n356 = Index Array(array=w575, index #1=w579, index #2=w578) -> (element #1=w577:u16, element #2=w576:u16)
              n357 = Not Equal To 0?(x=w576) -> (x != 0?=w562:bool)
              n358 = Not Equal To 0?(x=w577) -> (x != 0?=w563:bool)
              n359 = Select(t=w570, s=w563, f=w569) -> (s? t:f=w571:u16)
              n360 = Select(t=w570, s=w562, f=w569) -> (s? t:f=w565:u16)
              n361 = call "myRIO_BRig_RT_dataMTrig_Audio_c__L.vi"() -> ("output_Audio_c__L"=w573:i32)  [unwired: 11 in]
              n362 = call "myRIO_BRig_RT_dataMTrig_Audio_N__L.vi"() -> ("output_Audio_N__L"=w572:i32)  [unwired: 11 in]
              n363 = call "myRIO_BRig_RT_dataMTrig_Audio_c__R.vi"() -> ("output_Audio_c__R"=w568:i32)  [unwired: 11 in]
              n364 = call "myRIO_BRig_RT_dataMTrig_Audio_N__R.vi"() -> ("output_Audio_N__R"=w567:i32)  [unwired: 11 in]
              n365 = Replace Array Subset(array=w575, new element #1=w566, index #1=w573, new element #2=w571, index #2=w572, new element #3=w566, index #3=w568, new element #4=w565, index #4=w567) -> (w574:u16[])
            }
            frame "Cue" {
              # "lick did not occur or warmupType==1"
              # "lick occurred?"
              # "Ncycle"
              # "Audio_R"
              # "Ncycle"
              # "Audio_L"
              n366 = local read "warmupType"() -> (w589:u8)
              n367 = Greater?(x=w595, y=w594) -> (0:w598:bool)
              n368 = Greater?(x=w597, y=w596) -> (0:w593:bool)
              n369 = Or(x=w593, y=w598) -> (x .or. y?=w587:bool)
              n370 = Equal?(x=w589, y=u8 1) -> (x = y?=w583:bool)
              n371 = Not(x=w587) -> (.not. x?=w586:bool)
              n372 = call "myRIO_BRig_RT_dataMTrig_Audio_N__L.vi"() -> ("output_Audio_N__L"=w601:i32)  [unwired: 11 in]
              n373 = call "myRIO_BRig_RT_dataMTrig_Audio_N__R.vi"() -> ("output_Audio_N__R"=w600:i32)  [unwired: 11 in]
              n374 = Or(x=w586, y=w583) -> (x .or. y?=w584:bool)
              n375 = case shown="True" w584 {
                tunnel: w601 -> [w607 w625]
                tunnel: w600 -> [w606 w624]
                tunnel: w592 -> [w609 w619]
                tunnel: [w608 w619] -> w591
                tunnel: w590 -> [_ w617]
                tunnel: [myRIO_BRig_RT__Case_NonExp_stateList."Idle" ("t") w616] -> w585
                tunnel: w583 -> [_ w615]
                tunnel: w582 -> [_ w611]
                tunnel: w581 -> [_ w610]
                frame False {
                  w602 = u16 0 ("new element/subarray")
                  # "lick occurred and warmupType==2"
                  n376 = call "myRIO_BRig_RT_dataMTrig_Solenoid_N__R.vi"() -> ("output_Solenoid_N__R"=w603:i32)  [unwired: 11 in]
                  n377 = call "myRIO_BRig_RT_dataMTrig_Solenoid_N__L.vi"() -> ("output_Solenoid_N__L"=w604:i32)  [unwired: 11 in]
                  n378 = Replace Array Subset(array=w609, new element #1=w602, index #1=w607, new element #2=w602, index #2=w606, new element #3=w602, index #3=w604, new element #4=w602, index #4=w603) -> (w608:u16[])
                }
                frame True {
                  n379 = Not(x=w615) -> (.not. x?=w614:bool)
                  n380 = Index Array(array=w619, index #1=w625, index #2=w624) -> (element #1=w623:u16, element #2=w622:u16)
                  n381 = Equal To 0?(x=w623) -> (x = 0?=w621:bool)
                  n382 = Equal To 0?(x=w622) -> (x = 0?=w620:bool)
                  n383 = And(x=w621, y=w620) -> (x .and. y?=w613:bool)
                  n384 = And(x=w613, y=w614) -> (x .and. y?=w612:bool)
                  n385 = case shown="True" w612 {
                    tunnel: w611 -> [_ w633]
                    tunnel: w610 -> [_ w628]
                    frame False {
                    }
                    frame True {
                      n386 = local read "count_warmup_R"() -> (w626:u16)
                      n387 = local read "count_warmup_L"() -> (w631:u16)
                      n388 = Increment(x=w626) -> (x+1=w629:u16)
                      n389 = Increment(x=w631) -> (x+1=w632:u16)
                      n390 = Select(t=w629, s=w628, f=w626) -> (s? t:f=w627:u16)
                      n391 = Select(t=w632, s=w633, f=w631) -> (s? t:f=w630:u16)
                      n392 = local write "count_warmup_R"(w627) -> ()
                      n393 = local write "count_warmup_L"(w630) -> ()
                    }
                  }
                  n394 = Select(t=myRIO_BRig_RT__Case_NonExp_stateList."DispenseWater_pre", s=w613, f=w617) -> (s? t:f=w616:T1)
                }
              }
            }
            frame "RewardCalibration_pre" {
              (unwired) FALSE
              w635 = FALSE
              w646 = u8 0
              w662 = u8 0
              # "Are we starting a RewardCalibration?\nOr are we stopping a RewardCalibration?\nOr is a RewardCalibration over?"
              # "RewCalib\nOnOff"
              # "N"
              # "Solenoid R"
              # "RewCalib\nOnOff"
              # "N"
              # "Solenoid L"
              n395 = local read "RewCalib_Trig_L"() -> (w669:bool)
              n396 = local read "RewCalib_Trig_R"() -> (w638:bool)
              n397 = call "myRIO_BRig_RT_dataMTrig_Solenoid_N__R.vi"() -> ("output_Solenoid_N__R"=w640:i32)  [unwired: 11 in]
              n398 = call "myRIO_BRig_RT_dataMTrig_Solenoid_RewCalib_OnOff__R.vi"() -> ("output_Solenoid_RewCalib_OnOff__R"=w637:i32)  [unwired: 11 in]
              n399 = call "myRIO_BRig_RT_dataMTrig_Solenoid_N__L.vi"() -> ("output_Solenoid_N__L"=w655:i32)  [unwired: 11 in]
              n400 = call "myRIO_BRig_RT_dataMTrig_Solenoid_RewCalib_OnOff__L.vi"() -> ("output_Solenoid_RewCalib_OnOff__L"=w656:i32)  [unwired: 11 in]
              n401 = Index Array(array=w639, index #1=w640, index #2=w637) -> (element #1=w650:u16, element #2=w645:u16)
              n402 = Index Array(array=w639, index #1=w655, index #2=w656) -> (element #1=w666:u16, element #2=w661:u16)
              n403 = Equal To 0?(x=w650) -> (x = 0?=w651:bool)
              n404 = Not Equal To 0?(x=w645) -> (x != 0?=w648:bool)
              n405 = Equal To 0?(x=w666) -> (x = 0?=w667:bool)
              n406 = Not Equal To 0?(x=w661) -> (x != 0?=w664:bool)
              n407 = local write "MTrig_Solenoid_trig__L"(w635) -> ()
              n408 = local write "MTrig_Solenoid_trig__R"(w635) -> ()
              n409 = Select(t=u8 1, s=w638, f=w646) -> (s? t:f=w642:u8)
              n410 = Select(t=u8 1, s=w669, f=w662) -> (s? t:f=w658:u8)
              n411 = Select(t=u8 2, s=w651, f=w646) -> (s? t:f=w643:u8)
              n412 = Select(t=u8 4, s=w648, f=w646) -> (s? t:f=w644:u8)
              n413 = Select(t=u8 2, s=w667, f=w662) -> (s? t:f=w659:u8)
              n414 = Select(t=u8 4, s=w664, f=w662) -> (s? t:f=w660:u8)
              n415 = Compound Arithmetic op=ADD(w642, w643, w644) -> (w641:u8)
              n416 = Compound Arithmetic op=ADD(w658, w659, w660) -> (w657:u8)
              n417 = case shown="7" w657 {
                tunnel: w639 -> [w699 w704 w706 w711 w716 w718 w721 w726]
                tunnel: [w699 w705 w706 w712 w717 w718 w722 w727] -> w654
                tunnel: w656 -> [_ w702 _ w709 w714 _ w720 w725]
                tunnel: w655 -> [_ w703 _ w710 w715 _ _ _]
                frame 0, Default {
                }
                frame 1 {
                  n418 = Replace Array Subset(array=w704, new element #1=u16 100 ("new element/subarray"), index #1=w703, new element #2=u16 1 ("new element/subarray"), index #2=w702) -> (w705:u16[])
                }
                frame 2 {
                }
                frame 3 {
                  n419 = Replace Array Subset(array=w711, new element #1=u16 100 ("new element/subarray"), index #1=w710, new element #2=u16 1 ("new element/subarray"), index #2=w709) -> (w712:u16[])
                }
                frame 4 {
                  w713 = u16 0 ("new element/subarray")
                  n420 = Replace Array Subset(array=w716, new element #1=w713, index #1=w715, new element #2=w713, index #2=w714) -> (w717:u16[])
                }
                frame 5 {
                }
                frame 6 {
                  n421 = Replace Array Subset(array=w721, new element=u16 0 ("new element/subarray"), index=w720) -> (w722:u16[])
                }
                frame 7 {
                  n422 = local write "RewCalib_Trig_L"(FALSE ("RewCalib_Trig_L")) -> ()
                  n423 = Replace Array Subset(array=w726, new element=u16 0 ("new element/subarray"), index=w725) -> (w727:u16[])
                }
              }
              n424 = case shown="7" w641 {
                tunnel: w654 -> [w670 w675 w677 w682 w687 w689 w692 w697]
                tunnel: [w670 w676 w677 w683 w688 w689 w693 w698] -> w653
                tunnel: w637 -> [_ w673 _ w680 w685 _ w691 w696]
                tunnel: w640 -> [_ w674 _ w681 w686 _ _ _]
                frame 0, Default {
                }
                frame 1 {
                  n425 = Replace Array Subset(array=w675, new element #1=u16 100 ("new element/subarray"), index #1=w674, new element #2=u16 1 ("new element/subarray"), index #2=w673) -> (w676:u16[])
                }
                frame 2 {
                }
                frame 3 {
                  n426 = Replace Array Subset(array=w682, new element #1=u16 100 ("new element/subarray"), index #1=w681, new element #2=u16 1 ("new element/subarray"), index #2=w680) -> (w683:u16[])
                }
                frame 4 {
                  w684 = u16 0 ("new element/subarray")
                  n427 = Replace Array Subset(array=w687, new element #1=w684, index #1=w686, new element #2=w684, index #2=w685) -> (w688:u16[])
                }
                frame 5 {
                }
                frame 6 {
                  n428 = Replace Array Subset(array=w692, new element=u16 0 ("new element/subarray"), index=w691) -> (w693:u16[])
                }
                frame 7 {
                  n429 = local write "RewCalib_Trig_R"(FALSE ("RewCalib_Trig_L")) -> ()
                  n430 = Replace Array Subset(array=w697, new element=u16 0 ("new element/subarray"), index=w696) -> (w698:u16[])
                }
              }
            }
            frame "DispenseWater_pre" {
              w734 = u16 0 ("t")
              w777 = u16 0 ("new element/subarray")
              # "just trust me on this one"
              # "RewCalib\nOnOff"
              # "RewCalib\nOnOff"
              # "nCycle"
              # "Solenoid__R"
              # "Tdelay"
              # "delay"
              # "nCycle"
              # "Solenoid__L"
              # "Tdelay"
              # "delay"
              # "Solenoid__R"
              # "count"
              # "Solenoid_Tcycle_R"
              # "Solenoid_Tcycle_L"
              # "Solenoid__L"
              # "count"
              n431 = call "myRIO_BRig_RT_dataMTrig_Solenoid_RewCalib_OnOff__L.vi"() -> ("output_Solenoid_RewCalib_OnOff__L"=w741:i32)  [unwired: 11 in]
              n432 = call "myRIO_BRig_RT_dataMTrig_Solenoid_N__L.vi"() -> ("output_Solenoid_N__L"=w732:i32)  [unwired: 11 in]
              n433 = call "myRIO_BRig_RT_dataMTrig_Solenoid_delay__L.vi"() -> ("output_Solenoid_delay__L"=w775:i32)  [unwired: 11 in]
              n434 = call "myRIO_BRig_RT_dataMTrig_Solenoid_Tdelay__L.vi"() -> ("output_Solenoid_Tdelay__L"=w774:i32)  [unwired: 11 in]
              n435 = call "myRIO_BRig_RT_dataMTrig_Solenoid_N__R.vi"() -> ("output_Solenoid_N__R"=w730:i32)  [unwired: 11 in]
              n436 = call "myRIO_BRig_RT_dataMTrig_Solenoid_delay__R.vi"() -> ("output_Solenoid_delay__R"=w764:i32)  [unwired: 11 in]
              n437 = call "myRIO_BRig_RT_dataMTrig_Solenoid_Tdelay__R.vi"() -> ("output_Solenoid_Tdelay__R"=w763:i32)  [unwired: 11 in]
              n438 = call "myRIO_BRig_RT_dataMTrig_Solenoid_RewCalib_OnOff__R.vi"() -> ("output_Solenoid_RewCalib_OnOff__R"=w737:i32)  [unwired: 11 in]
              n439 = Index Array(array=w776, index #1=w732, index #2=w775, index #3=w774, index #4=w730, index #5=w764, index #6=w763, index #7=w741, index #8=w737) -> (element #1=w733:u16, element #2=w773:u16, element #3=w768:u16, element #4=w736:u16, element #5=w758:u16, element #6=w757:u16, element #7=w742:u16, element #8=w739:u16)
              n440 = Equal To 0?(x=w773) -> (x = 0?=w772:bool)
              n441 = Equal To 0?(x=w758) -> (x = 0?=w762:bool)
              n442 = local read "RewCalib_Trig_L"() -> (w753:bool)
              n443 = local read "RewCalib_Trig_R"() -> (w748:bool)
              n444 = Not Equal To 0?(x=w733) -> (x != 0?=w771:bool)
              n445 = Not Equal To 0?(x=w736) -> (x != 0?=w761:bool)
              n446 = local read "MTrig_Solenoid_Tcycle__L"() -> (w770:u16)
              n447 = local read "MTrig_Solenoid_Tcycle__R"() -> (w756:u16)
              n448 = Not Equal To 0?(x=w742) -> (x != 0?=w752:bool)
              n449 = Not Equal To 0?(x=w739) -> (x != 0?=w750:bool)
              n450 = Not(x=w753) -> (.not. x?=w751:bool)
              n451 = Not(x=w748) -> (.not. x?=w749:bool)
              n452 = And(x=w752, y=w751) -> (x .and. y?=w747:bool)
              n453 = And(x=w750, y=w749) -> (x .and. y?=w746:bool)
              n454 = call "myRIO_BRig_RT_dataMTrig_Solenoid_c__L.vi"() -> ("output_Solenoid_c__L"=w779:i32)  [unwired: 11 in]
              n455 = call "myRIO_BRig_RT_dataMTrig_Solenoid_c__R.vi"() -> ("output_Solenoid_c__R"=w778:i32)  [unwired: 11 in]
              n456 = Select(t=w770, s=w771, f=u16 0) -> (s? t:f=w767:u16)
              n457 = Or(x=w747, y=w746) -> (x .or. y?=w735:bool)
              n458 = Select(t=w756, s=w761, f=u16 0) -> (s? t:f=w759:u16)
              n459 = Select(t=w767, s=w772, f=w768) -> (s? t:f=w765:u16)
              n460 = Select(t=w759, s=w762, f=w757) -> (s? t:f=w754:u16)
              n461 = call "myRIO_BRig_RT_dataMTrig_Solenoid_Tcycle__L.vi"() -> ("output_Solenoid_Tcycle__L"=w766:i32)  [unwired: 11 in]
              n462 = call "myRIO_BRig_RT_dataMTrig_Solenoid_Tcycle__R.vi"() -> ("output_Solenoid_Tcycle__R"=w755:i32)  [unwired: 11 in]
              n463 = Select(t=w734, s=w735, f=w733) -> (s? t:f=w731:u16)
              n464 = Select(t=w734, s=w735, f=w736) -> (s? t:f=w729:u16)
              n465 = Select(t=myRIO_BRig_RT__Case_NonExp_stateList."Idle" ("Enum"), s=w735, f=myRIO_BRig_RT__Case_NonExp_stateList."DispenseWater" ("Enum")) -> (s? t:f=w743:T1)
              n466 = Select(t=w734, s=w735, f=w742) -> (s? t:f=w740:u16)
              n467 = Select(t=w734, s=w735, f=w739) -> (s? t:f=w738:u16)
              n468 = Replace Array Subset(array=w776, new element #1=w777, index #1=w779, new element #2=w777, index #2=w778, new element #3=w765, index #3=w766, new element #4=w754, index #4=w755, new element #5=w740, index #5=w741, new element #6=w738, index #6=w737, new element #7=w731, index #7=w732, new element #8=w729, index #8=w730) -> (w780:u16[])
            }
            frame "DispenseWater" {
              # "D"
              # "C"
              # "B"
              # "A"
              # "(A) Add COUNT and INCREMENT\n(B) Is (A) smaller than Tcycle?\n(C) Are we dispensing water or in the delay phase?\n(D) If (A) is smaller than Tcycle   AND   if we are dispensing water\n      then send TRUE to solenoid"
              # "delay"
              # "Tcycle"
              # "Solenoid__R"
              # "count"
              # "delay"
              # "Tcycle"
              # "Solenoid__L"
              # "count"
              n469 = To Unsigned Word Integer(number=w808) -> (unsigned 16bit integer=w790:u16)
              n470 = call "myRIO_BRig_RT_dataMTrig_Solenoid_delay__R.vi"() -> ("output_Solenoid_delay__R"=w794:i32)  [unwired: 11 in]
              n471 = call "myRIO_BRig_RT_dataMTrig_Solenoid_c__R.vi"() -> ("output_Solenoid_c__R"=w793:i32)  [unwired: 11 in]
              n472 = call "myRIO_BRig_RT_dataMTrig_Solenoid_Tcycle__R.vi"() -> ("output_Solenoid_Tcycle__R"=w795:i32)  [unwired: 11 in]
              n473 = call "myRIO_BRig_RT_dataMTrig_Solenoid_delay__L.vi"() -> ("output_Solenoid_delay__L"=w810:i32)  [unwired: 11 in]
              n474 = call "myRIO_BRig_RT_dataMTrig_Solenoid_c__L.vi"() -> ("output_Solenoid_c__L"=w802:i32)  [unwired: 11 in]
              n475 = call "myRIO_BRig_RT_dataMTrig_Solenoid_Tcycle__L.vi"() -> ("output_Solenoid_Tcycle__L"=w811:i32)  [unwired: 11 in]
              n476 = Index Array(array=w804, index #1=w802, index #2=w811, index #3=w810, index #4=w793, index #5=w795, index #6=w794) -> (element #1=w809:u16, element #2=w799:u16, element #3=w807:u16, element #4=w789:u16, element #5=w786:u16, element #6=w785:u16)
              n477 = Add(x=w809, y=w790) -> (x+y=w800:u16)
              n478 = Add(x=w789, y=w790) -> (x+y=w791:u16)
              n479 = Less?(x=w800, y=w799) -> (x < y?=w783:bool)
              n480 = Equal To 0?(x=w807) -> (x = 0?=w806:bool)
              n481 = Less?(x=w791, y=w786) -> (x < y?=w784:bool)
              n482 = Equal To 0?(x=w785) -> (x = 0?=w792:bool)
              n483 = And(x=w783, y=w806) -> (x .and. y?=w805:bool)
              n484 = Or(x=w783, y=w784) -> (x .or. y?=w782:bool)
              n485 = And(x=w784, y=w792) -> (x .and. y?=w787:bool)
              n486 = Select(t=w800, s=w783, f=w799) -> (s? t:f=w801:u16)
              n487 = Select(t=w791, s=w784, f=w786) -> (s? t:f=w788:u16)
              n488 = Replace Array Subset(array=w804, new element #1=w801, index #1=w802, new element #2=w788, index #2=w793) -> (w803:u16[])
              n489 = Select(t=w798, s=w782, f=myRIO_BRig_RT__Case_NonExp_stateList."DispenseWater_post" ("Enum")) -> (s? t:f=w796:T1)
            }
            frame "DispenseWater_post" {
              # "nCycle"
              # "delay"
              # "Solenoid__R"
              # "nCycle"
              # "delay"
              # "Solenoid__L"
              n490 = call "myRIO_BRig_RT_dataMTrig_Solenoid_N__L.vi"() -> ("output_Solenoid_N__L"=w829:i32)  [unwired: 11 in]
              n491 = call "myRIO_BRig_RT_dataMTrig_Solenoid_delay__L.vi"() -> ("output_Solenoid_delay__L"=w828:i32)  [unwired: 11 in]
              n492 = call "myRIO_BRig_RT_dataMTrig_Solenoid_N__R.vi"() -> ("output_Solenoid_N__R"=w825:i32)  [unwired: 11 in]
              n493 = call "myRIO_BRig_RT_dataMTrig_Solenoid_delay__R.vi"() -> ("output_Solenoid_delay__R"=w824:i32)  [unwired: 11 in]
              n494 = Index Array(array=w831, index #1=w829, index #2=w828, index #3=w825, index #4=w824) -> (element #1=w833:u16, element #2=w832:u16, element #3=w816:u16, element #4=w818:u16)
              n495 = Not Equal To 0?(x=w833) -> (x != 0?=w834:bool)
              n496 = Not Equal To 0?(x=w816) -> (x != 0?=w817:bool)
              n497 = case shown="True" w817 {
                selector: w817 -> [_ w838]
                tunnel: w816 -> [w836 w844]
                tunnel: w818 -> [_ w845]
                tunnel: [w836 w842] -> w815
                tunnel: [u16 0 w841] -> w814
                tunnel: [_ w838] -> w813
                frame False {
                }
                frame True {
                  n498 = Equal To 0?(x=w845) -> (x = 0?=w837:bool)
                  n499 = Decrement(x=w844) -> (x-1=w843:u16)
                  n500 = Select(t=w843, s=w837, f=w844) -> (s? t:f=w842:u16)
                  n501 = Select(t=u16 1, s=w837, f=u16 0) -> (s? t:f=w841:u16)
                }
              }
              n502 = case shown="True" w834 {
                selector: w834 -> [_ w849]
                tunnel: w833 -> [w847 w855]
                tunnel: w832 -> [_ w856]
                tunnel: [w847 w853] -> w827
                tunnel: [u16 0 w852] -> w826
                tunnel: [_ w849] -> w823
                frame False {
                }
                frame True {
                  n503 = Equal To 0?(x=w856) -> (x = 0?=w848:bool)
                  n504 = Decrement(x=w855) -> (x-1=w854:u16)
                  n505 = Select(t=w854, s=w848, f=w855) -> (s? t:f=w853:u16)
                  n506 = Select(t=u16 1, s=w848, f=u16 0) -> (s? t:f=w852:u16)
                }
              }
              n507 = Or(x=w823, y=w813) -> (x .or. y?=w822:bool)
              n508 = Replace Array Subset(array=w831, new element #1=w827, index #1=w829, new element #2=w826, index #2=w828, new element #3=w815, index #3=w825, new element #4=w814, index #4=w824) -> (w830:u16[])
              n509 = Select(t=myRIO_BRig_RT__Case_NonExp_stateList."DispenseWater_pre" ("Enum"), s=w822, f=myRIO_BRig_RT__Case_NonExp_stateList."Idle" ("Enum")) -> (s? t:f=w819:T1)
            }
            frame "TestConnection" {
              n510 = local read "Host Password"() -> (w863:string)
              n511 = local read "Host UserName"() -> (w864:string)
              n512 = call "myRIO_BRig_RT_comm_webdav_testConnect.vi"("input_password"=w863, "input_username"=w864) -> ("output_Iconnected"=w861:bool)  [unwired: 9 in]
              n513 = Select(t="Connection accepted!" ("message"), s=w861, f="Error!") -> (s? t:f=w859:string)
              n514 = One Button Dialog(message=w859) -> ()  [unwired: 1 in, 1 out]
            }
            frame "SendData" {
              n515 = local read "Data Set Prefix"() -> (w866:string)
              n516 = local read "Host Password"() -> (w867:string)
              n517 = local read "Host UserName"() -> (w868:string)
              n518 = call "myRIO_BRig_RT_comm_webdav_sendData_all.vi"("Host Filename Prefix"=w866, "Host Password"=w867, "Host UserName"=w868) -> ()  [unwired: 9 in]
            }
            frame "Get_FPGA_count_per_ms" {
              n519 = case shown="False" w882 {
                selector: w882 -> [w885 _]
                tunnel: w880 -> [_ w898]
                tunnel: [w889 w898] -> w879
                tunnel: w878 -> [w888 w896]
                tunnel: w877 -> [w887 w895]
                tunnel: [w886 w893] -> w876
                tunnel: [w885 w892] -> w875
                frame False {
                  n520 = Get Date/Time In Seconds() -> (seconds since 1Jan1904=w890:timestamp)
                  n521 = xnode "Read/Write Control"("FPGA VI Reference In"=w888, "error in"=w887, "timeTrial"=TRUE) -> ("error out"=w886:errorcluster)  [unwired: 1 out]
                  n522 = To Double Precision Float(number=w890) -> (double precision float=w889:dbl)
                  n523 = local write "get_countPerMS"(w885) -> ()
                }
                frame True {
                  w894 = 1.0
                  n524 = Get Date/Time In Seconds() -> (seconds since 1Jan1904=w899:timestamp)
                  n525 = To Double Precision Float(number=w899) -> (double precision float=w900:dbl)
                  n526 = Subtract(x=w900, y=w898) -> (x-y=w897:dbl)
                  n527 = Less Or Equal?(x=w894, y=w897) -> (x <= y?=w892:bool)
                  n528 = case shown="True" w892 {
                    tunnel: w896 -> [_ w913]
                    tunnel: w895 -> [w901 w912]
                    tunnel: w894 -> [_ w903]
                    tunnel: [w901 w902] -> w893
                    frame False {
                    }
                    frame True {
                      n529 = xnode "Read/Write Control"("FPGA VI Reference In"=w913, "error in"=w912) -> ("FPGA VI Reference Out"=w910:refnum<k20>, "error out"=w909:errorcluster, "count_timeTrial"=w904:u32)
                      n530 = Multiply(x=w903, y=1000.0) -> (x*y=w907:dbl)
                      n531 = To Double Precision Float(number=w904) -> (double precision float=w906:dbl)
                      n532 = Divide(x=w906, y=w907) -> (x/y=w908:dbl)
                      n533 = local write "f_millisec2count"(w908) -> ()
                      n534 = xnode "Read/Write Control"("FPGA VI Reference In"=w910, "error in"=w909, "timeTrial"=FALSE) -> ("error out"=w902:errorcluster)  [unwired: 1 out]
                    }
                  }
                }
              }
              "error out 5" <- w876
              n535 = Select(t=myRIO_BRig_RT__Case_NonExp_stateList."Idle" ("Enum"), s=w875, f=w873) -> (s? t:f=w872:T1)
            }
            frame "End" {
            }
          }
          n536 = local read "MTrig_Audio_trig__R"() -> (w119:bool)
          n537 = local read "MTrig_Audio_trig__L"() -> (w118:bool)
          n538 = local read "START"() -> (w114:bool)
          n539 = local read "STOP_abort"() -> (w113:bool)
          n540 = local read "MTrig_Laser_trig"() -> (w120:bool)
          n541 = call "myRIO_BRig_RT_dataMTrig_main__v2.vi"("input_dataMTrig"=w122, "input_Audio_trig_L"=w118, "input_Audio_trig_R"=w119, "input_Laser_trig"=w120) -> ("output_dataMTrig"=w121:u16[], "output_Audio_L"=w98:bool, "output_Audio_R"=w109:bool, "output_Laser"=w101:bool)  [unwired: 12 in]
          n542 = Or(x=w114, y=w113) -> (x .or. y?=w112:bool)
          n543 = Select(t=myRIO_BRig_RT__Case_NonExp_stateList."End" ("Enum"), s=w112, f=w111) -> (s? t:f=w110:T1)
          n544 = Or(x=w119, y=w120) -> (x .or. y?=w117:bool)
          n545 = Or(x=w117, y=w118) -> (x .or. y?=w116:bool)
          n546 = case shown="True" w116 {
            frame False {
            }
            frame True {
              w135 = FALSE
              n547 = local write "MTrig_Audio_trig__R"(w135) -> ()
              n548 = local write "MTrig_Audio_trig__L"(w135) -> ()
              n549 = local write "MTrig_Laser_trig"(w135) -> ()
            }
          }
          n550 = xnode "Read/Write Control"("FPGA VI Reference In"=w87, "error in"=w86, "A1_SR"=w123, "A3_SL"=w124, "audioTrigger_L"=w98, "audioTrigger_R"=w109, "laserResponse_reward_LED"="laserResponse_reward_LED", "laserResponse_wrong_LED"="laserResponse_wrong_LED", "laserResponse_reward"="laserResponse_reward", "laserResponse_wrong"="laserResponse_wrong", "SelectionState"="SelectionState", "ignoreWrong"="ignoreWrong", "Left(F)_or_Right(T)"="Left(F)_or_Right(T)", "laserMTrig"=w101) -> ("FPGA VI Reference Out"=w129:refnum<k20>, "error out"=w128:errorcluster, "SelectReward"=→"SelectReward":bool, "SelectWrong"=→"SelectWrong":bool)
          n551 = node-c288() -> ()  [unwired: 1 in, 1 out]
          "cState_NonExp" <- w127
        }
        n552 = node-c288(w70) -> ()  [unwired: 1 out]
        n553 = flat-sequence {
          tunnel: w63 -> [w81]
          tunnel: [w81] -> w62
          tunnel: w61 -> [w80]
          tunnel: [w80] -> w60
          frame #0 {
            w79 = FALSE
            n554 = local write "STOP_endBlock"(w79) -> ()
            n555 = local write "STOP_endTrial"(w79) -> ()
          }
        }
      }
      frame True {
        w923 = u16 0
        w942 = u8 0
        w943 = FALSE ("SelectionState")
        w948 = u16 0 ("idxDataBlock")
        w950 = u16 100 ("new element/subarray")
        w951 = u16 100 ("new element/subarray")
        w971 = T7 refnum items=["Session NI_WebDAV"] ("output_hSession")
        w980 = FALSE
        w981 = u16 0
        w930 = FALSE
        # "dummyState counter"
        # "audio__L\naudio__R"
        # "Audio params"
        # "nRewards"
        # "idxDataBlock"
        # "Solenoid_Tdelay_R"
        # "Solenoid_Tdelay_L"
        # "RewCalib_N__R"
        # "RewCalib_N__L"
        # "Save dataLick to file\nSend file to Host\nSave dataMTrig\nSend file to Host\nDisconnect"
        # "dataTrial"
        # "dataTrial"
        # "Solenoid_Tcycle_R"
        # "Solenoid_Tcycle_L"
        # "Laser_Tcycle"
        # "Audio_Tcycle_R"
        # "Audio_Tcycle_L"
        # "dataLick"
        # "dataLC"
        # "dataLC"
        # "dataBlock"
        # "dataBlock"
        # "dataMTrig"
        # "dataMTrig"
        # "dataExp"
        # "dataCurrent"
        # "dataExp"
        # "dataCurrent"
        # "spout"
        # "state"
        n556 = call "myRIO_BRig_RT_dataMTrig_Solenoid_Tcycle__L.vi"() -> ("output_Solenoid_Tcycle__L"=w977:i32)  [unwired: 11 in]
        n557 = call "myRIO_BRig_RT_dataMTrig_Solenoid_Tcycle__R.vi"() -> ("output_Solenoid_Tcycle__R"=w976:i32)  [unwired: 11 in]
        n558 = call "myRIO_BRig_RT_dataMTrig_Audio_Tcycle__L.vi"() -> ("output_Audio_Tcycle__L"=w975:i32)  [unwired: 11 in]
        n559 = call "myRIO_BRig_RT_dataMTrig_Audio_Tcycle__R.vi"() -> ("output_Audio_Tcycle__R"=w974:i32)  [unwired: 11 in]
        n560 = call "myRIO_BRig_RT_dataMTrig_Laser_Tcycle.vi"() -> ("output_Laser_Tcycle"=w973:i32)  [unwired: 11 in]
        n561 = local read "MTrig_Solenoid_Tcycle__L"() -> (w956:u16)
        n562 = local read "MTrig_Solenoid_Tcycle__R"() -> (w955:u16)
        n563 = local read "Tcycle_Reward_L"() -> (w952:u16)
        n564 = local read "Tcycle_Reward_R"() -> (w953:u16)
        n565 = local read "MTrig_Laser_Tcycle"() -> (w954:u16)
        n566 = call "myRIO_BRig_RT_dataMTrig_Solenoid_RewCalib_nCycle__L.vi"() -> ("output_Solenoid_RewCalib_nCycle__L"=w959:i32)  [unwired: 11 in]
        n567 = call "myRIO_BRig_RT_dataMTrig_Solenoid_Tdelay__L.vi"() -> ("output_Solenoid_Tdelay__L"=w961:i32)  [unwired: 11 in]
        n568 = call "myRIO_BRig_RT_dataMTrig_Solenoid_RewCalib_nCycle__R.vi"() -> ("output_Solenoid_RewCalib_nCycle__R"=w960:i32)  [unwired: 11 in]
        n569 = call "myRIO_BRig_RT_dataMTrig_Solenoid_Tdelay__R.vi"() -> ("output_Solenoid_Tdelay__R"=w962:i32)  [unwired: 11 in]
        n570 = case shown="False" w934 {
          selector: w934 -> [_ w1003]
          tunnel: w933 -> [w1000 w1005]
          tunnel: [w1001 w1005] -> w928
          tunnel: w932 -> [_ w1004]
          tunnel: [w1002 w1004] -> w929
          tunnel: [w999 w1003] -> w927
          frame False {
            n571 = call "myRIO__TCP_connect_forWriting.vi"("input_error"=w1000) -> ("output_error"=w1001:errorcluster, "output_connected"=w999:bool, "output_hTCP"=w1002:refnum<k5>)  [unwired: 8 in]
          }
          frame True {
          }
        }
        n572 = call "myRIO_BRig_RT_dataLick_init.vi"() -> ("output_dataLick"=w983:u16[][])  [unwired: 11 in]
        n573 = call "myRIO_BRig_RT_dataCurrent_init.vi"() -> ("output_dataCurrent"=w990:u16[])  [unwired: 11 in]
        n574 = call "myRIO_BRig_RT_dataExp_init.vi"() -> ("output_dataExp"=w989:u16[])  [unwired: 11 in]
        n575 = call "myRIO_BRig_RT_dataMTrig_init.vi"() -> ("output_dataMTrig"=w979:u16[])  [unwired: 5 in]
        n576 = call "myRIO_BRig_RT_dataLC_init.vi"() -> ("output_dataLC"=w987:u16[])  [unwired: 11 in]
        n577 = call "myRIO_BRig_RT_dataBlock_init.vi"() -> ("output_dataBlock"=w988:u16[][])  [unwired: 11 in]
        n578 = call "myRIO_BRig_RT_dataTrial_init.vi"() -> ("output_dataTrial"=w972:u16[][])  [unwired: 11 in]
        n579 = xnode "Read/Write Control"("FPGA VI Reference In"=w944, "error in"=w945, "SelectionState"=w943, "laserResponse_reward"=w943, "laserResponse_wrong"=w943, "laserResponse_reward_LED"=w943, "laserResponse_wrong_LED"=w943, "Left(F)_or_Right(T)"=w943, "ignoreWrong"=w943, "SelectionState"=w943) -> ("FPGA VI Reference Out"=w946:refnum<k20>, "error out"=w947:errorcluster)
        n580 = local write "I_connect_TCP"(w927) -> ()
        n581 = Replace Array Subset(array=w979, new element #1=w951, index #1=w959, new element #2=w951, index #2=w960, new element #3=w950, index #3=w961, new element #4=w950, index #4=w962, new element #5=w956, index #5=w977, new element #6=w955, index #6=w976, new element #7=w952, index #7=w975, new element #8=w953, index #8=w974, new element #9=w954, index #9=w973) -> (w978:u16[])
        n582 = call "myRIO_BRig_RT_dataAnalog_init.vi"() -> ("output_dataAnalog"=w939:u16[][])  [unwired: 11 in]
        n583 = call "myRIO_BRig_RT_TCP__start_exp.vi"("input_hTCP"=w929, "input_I_connected_TCP"=w927, "input_error"=w928) -> ("output_hTCP"=w926:refnum<k5>, "output_error"=w925:errorcluster)  [unwired: 11 in]
        n584 = Get Date/Time In Seconds() -> (seconds since 1Jan1904=w958:timestamp)
        n585 = To Double Precision Float(number=w958) -> (double precision float=w957:dbl)
        n586 = node-c288() -> (w998:T3)  [unwired: 4 in]
        n587 = timed-loop {
          timing: w998 -> [_]
          timing-out: [_] -> w997
          shift-right: [w1122] -> _
          shift-left: myRIO_BRig_RT__Case_Exp_stateList."Start1" ("Enum") -> [w1055]
          shift-right: [w1052] -> _
          shift-left: enum16{"Left", "Right"}."Left" -> [w1173]
          tunnel: w946 -> [w1171]
          tunnel: w947 -> [w1170]
          shift-right: [w1165] -> _
          shift-left: w995 -> [w1169]
          shift-right: [w1164] -> _
          shift-left: w994 -> [w1168]
          tunnel: [w1147] -> w992
          tunnel: [w1148] -> w993
          shift-right: [w1149] -> w963
          shift-left: w990 -> [w1114]
          shift-right: [w1163] -> _
          shift-left: w989 -> [w1109]
          shift-right: [w1136] -> w967
          shift-left: w978 -> [w1137]
          shift-right: [w1161] -> _
          shift-left: w988 -> [w1162]
          shift-right: [w1159] -> _
          shift-left: w987 -> [w1160]
          shift-right: [w1151] -> w969
          shift-left: w983 -> [w1152]
          shift-right: [w1138] -> _
          shift-left: w981 -> [w1146]
          shift-right: [w1106] -> _
          shift-left: w942 -> [w1145]
          shift-right: [w1139] -> _
          shift-left: w981 -> [w1144]
          shift-right: [w1140] -> _
          shift-left: w942 -> [w1143]
          shift-right: [w1107] -> _
          shift-left: w980 -> [w1141]
          shift-right: [w1108] -> _
          shift-left: w980 -> [w1142]
          shift-right: [w1120] -> _
          shift-left: w972 -> [w1121]
          shift-right: [w1119] -> w965
          shift-left: w971 -> [w1117]
          shift-right: [w1118] -> w966
          shift-left: FALSE ("output_Iconnected") -> [w1116]
          tunnel: "Data Set Prefix" -> [w1115]
          tunnel: [w1115] -> w964
          shift-right: [w1091] -> _
          shift-left: w930 -> [w1113]
          tunnel: w957 -> [w1110]
          shift-right: [w1104] -> _
          shift-left: 0 ("idxDataBlock") -> [w1105]
          shift-right: [w1101] -> _
          shift-left: w948 -> [w1103]
          shift-right: [w1100] -> _
          shift-left: w948 -> [w1102]
          shift-right: [w1090] -> _
          shift-left: w930 -> [w1096]
          shift-right: [w1093] -> _
          shift-left: w930 -> [w1095]
          shift-right: [w1092] -> _
          shift-left: w930 -> [w1094]
          shift-right: [w1078] -> w937
          shift-left: 0 -> [w1062]
          shift-right: [w1053] -> _
          shift-left: w923 -> [w1073]
          shift-right: [w1054] -> _
          shift-left: w923 -> [w1069]
          shift-right: [w1082] -> _
          shift-left: FALSE -> [w1082]
          shift-right: [w1068] -> _
          shift-left: w923 -> [w1076]
          shift-right: [w1079] -> w938
          shift-left: w939 -> [w1080]
          tunnel: w926 -> [w1067]
          tunnel: [w1066] -> w936
          tunnel: w927 -> [w1063]
          tunnel: [w1063] -> w935
          tunnel: w925 -> [w1065]
          tunnel: [w1064] -> w931
          shift-right: [w1058] -> _
          shift-left: w930 -> [w1059]
          shift-right: [w1056] -> _
          shift-left: w930 -> [w1057]
          shift-right: [w1050] -> _
          shift-left: u16 0 -> [w1051]
          shift-right: [w1048] -> _
          shift-left: w923 -> [w1049]
          stop <- w1158 stop-if-true
          # "Sel"
          # "Sel"
          # "Cue1"
          # "Cue1"
          # "ENL1"
          # "ENL1"
          # "iState"
          # "dataAnalog"
          # "index"
          # "iEvent"
          # "iBlock"
          # "iTrial"
          # "Laser"
          # "Audio R"
          # "Audio L"
          # "Solenoid R"
          # "Solenoid L"
          # "manual triggering"
          # "dataTrial"
          # "dataBlock"
          # "nRewards"
          # "dataExp"
          # "dataCurrent"
          # "audio__L\naudio__R"
          # "time stamp"
          # "Audio params"
          # "nRewards"
          # "idxDataBlock"
          # "idxDataBlock"
          # "activate"
          # "audio__L\naudio__R"
          # "amp__R\nfreq__R"
          # "amp__L\nfreq__L"
          # "dataLC"
          # "solenoid__R"
          # "solenoid__L"
          # "Did a lick occur?"
          # "Update lick counter"
          # "spout"
          # "spout"
          # "state"
          # "state"
          n588 = node-c288() -> ()  [unwired: 1 in, 1 out]
          n589 = local read "MTrig_Solenoid_trig__L"() -> (w1134:bool)
          n590 = local read "MTrig_Solenoid_trig__R"() -> (w1133:bool)
          n591 = local read "MTrig_Audio_trig__L"() -> (w1132:bool)
          n592 = local read "MTrig_Audio_trig__R"() -> (w1131:bool)
          n593 = xnode "Read/Write Control"("FPGA VI Reference In"=w1171, "error in"=w1170) -> ("FPGA VI Reference Out"=w1099:refnum<k20>, "error out"=w1098:errorcluster, "A2_LickL"=w1165:u32, "A4_LickR"=w1164:u32)
          "A2" <- w1165
          "A4" <- w1164
          n594 = local read "MTrig_Laser_trig"() -> (w1130:bool)
          n595 = Greater?(x=w1165, y=w1169) -> (0:w1167:bool)
          n596 = Greater?(x=w1164, y=w1168) -> (0:w1166:bool)
          n597 = Or(x=w1167, y=w1166) -> (x .or. y?=w1172:bool)
          n598 = call "myRIO_BRig_RT_dataMTrig_main.vi"("input_dataMTrig"=w1137, "input_Solenoid_trig_L"=w1134, "input_Solenoid_trig_R"=w1133, "input_Audio_trig_L"=w1132, "input_Audio_trig_R"=w1131, "input_Laser_trig"=w1130) -> ("output_Laser"=w1088:bool, "output_dataMTrig"=w1136:u16[], "output_Solenoid_L"=w1124:bool, "output_Solenoid_R"=w1126:bool, "output_Audio_L"=w1128:bool, "output_Audio_R"=w1129:bool)  [unwired: 8 in]
          n599 = Compound Arithmetic op=OR(w1134, w1133, w1132, w1131, w1130) -> (w1135:bool)
          n600 = case shown="True" w1135 {
            frame False {
            }
            frame True {
              w1174 = FALSE
              n601 = local write "MTrig_Solenoid_trig__L"(w1174) -> ()
              n602 = local write "MTrig_Solenoid_trig__R"(w1174) -> ()
              n603 = local write "MTrig_Audio_trig__L"(w1174) -> ()
              n604 = local write "MTrig_Audio_trig__R"(w1174) -> ()
              n605 = local write "MTrig_Laser_trig"(w1174) -> ()
            }
          }
          n606 = case shown="80" w1055 {
            selector: w1055 -> [_ _ _ _ _ _ _ _ _ _ _ _ _ _ _ _ _ _ _ _ _ w1967 _ w2032 _ _ _ _ _ w2173 _ w2250 _ _ _ _ _ w2405 _ w2479 _ w2543 _ w2587 _ _ w2657 _ _ _ _ _ w2828 _ _ _ _ _ _ _ _ _ _ _ _ w3109 w3142]
            tunnel: [myRIO_BRig_RT__Case_Exp_stateList."Start2" ("Enum") myRIO_BRig_RT__Case_Exp_stateList."Start3" ("Enum") myRIO_BRig_RT__Case_Exp_stateList."saveSettings1" ("Enum") myRIO_BRig_RT__Case_Exp_stateList."saveSettings2" ("Enum") myRIO_BRig_RT__Case_Exp_stateList."saveSettings3" ("Enum") myRIO_BRig_RT__Case_Exp_stateList."saveSettings4_LC_ENL" ("Enum") myRIO_BRig_RT__Case_Exp_stateList."saveSettings5_LC_Cue" ("Enum") myRIO_BRig_RT__Case_Exp_stateList."saveSettings6_LC_Other" ("Enum") myRIO_BRig_RT__Case_Exp_stateList."setSettings_Audio" ("Enum") myRIO_BRig_RT__Case_Exp_stateList."setSettings_Laser" ("Enum") myRIO_BRig_RT__Case_Exp_stateList."commConnect" ("Enum") w1697 myRIO_BRig_RT__Case_Exp_stateList."initTrial" ("Enum") w1742 myRIO_BRig_RT__Case_Exp_stateList."initTrial3" ("Enum") myRIO_BRig_RT__Case_Exp_stateList."initTrial_LC_ENL1" ("Enum") myRIO_BRig_RT__Case_Exp_stateList."ENL1_pre" ("Enum") myRIO_BRig_RT__Case_Exp_stateList."initTrial_LC_Cue1" ("Enum") myRIO_BRig_RT__Case_Exp_stateList."initTrial_LC_Sel" ("Enum") myRIO_BRig_RT__Case_Exp_stateList."initTrial4" ("Enum") w1927 w1964 myRIO_BRig_RT__Case_Exp_stateList."ENL1Penalty" ("Enum") w2033 myRIO_BRig_RT__Case_Exp_stateList."endExp" ("Enum") myRIO_BRig_RT__Case_Exp_stateList."endExp" ("Enum") myRIO_BRig_RT__Case_Exp_stateList."endExp" ("Enum") myRIO_BRig_RT__Case_Exp_stateList."endExp" ("Enum") w2128 w2172 myRIO_BRig_RT__Case_Exp_stateList."Cue1Penalty" ("Enum") w2248 myRIO_BRig_RT__Case_Exp_stateList."endExp" ("Enum") myRIO_BRig_RT__Case_Exp_stateList."endExp" ("Enum") myRIO_BRig_RT__Case_Exp_stateList."endExp" ("Enum") myRIO_BRig_RT__Case_Exp_stateList."endExp" ("Enum") w2345 w2411 myRIO_BRig_RT__Case_Exp_stateList."SelectReward" ("Enum") w2480 myRIO_BRig_RT__Case_Exp_stateList."SelectRewardPost" ("Enum") w2544 myRIO_BRig_RT__Case_Exp_stateList."SelectWrong" ("Enum") w2583 myRIO_BRig_RT__Case_Exp_stateList."endTrial1" ("Enum") myRIO_BRig_RT__Case_Exp_stateList."SelectTimeout" ("Enum") w2659 myRIO_BRig_RT__Case_Exp_stateList."endTrial1" ("Enum") myRIO_BRig_RT__Case_Exp_stateList."endTrial2" ("Enum") myRIO_BRig_RT__Case_Exp_stateList."endTrial3" ("Enum") w2745 w2811 w2828 myRIO_BRig_RT__Case_Exp_stateList."initBlock" ("Enum") w2855 myRIO_BRig_RT__Case_Exp_stateList."commUpload_dataExp" ("Enum") myRIO_BRig_RT__Case_Exp_stateList."endBlock" ("Enum") myRIO_BRig_RT__Case_Exp_stateList."commUpload_dataLC" ("Enum") myRIO_BRig_RT__Case_Exp_stateList."commUpload_dataTrial" ("Enum") myRIO_BRig_RT__Case_Exp_stateList."commUpload_dataCurrent" ("Enum") myRIO_BRig_RT__Case_Exp_stateList."saveData_dataCurrent" ("Enum") myRIO_BRig_RT__Case_Exp_stateList."saveData_dataExp" ("Enum") myRIO_BRig_RT__Case_Exp_stateList."saveData_dataLC" ("Enum") myRIO_BRig_RT__Case_Exp_stateList."saveData_dataTrial" ("Enum") myRIO_BRig_RT__Case_Exp_stateList."commUpload_pre" ("Enum") w3108 w3141] -> w1122
            tunnel: [w1200 w1219 w1241 w1296 w1344 w1411 w1475 w1539 w1583 w1609 w1668 w1674 w1705 w1724 w1758 w1788 w1823 w1847 w1873 w1902 w1943 w1980 w2010 w2037 w2053 w2075 w2094 w2113 w2147 w2194 w2219 w2247 w2268 w2289 w2308 w2327 w2356 w2429 w2454 w2477 w2491 w2541 w2565 w2597 w2618 w2638 w2669 w2692 w2704 w2723 w2765 w2784 w2827 w2844 w2858 w2892 w2913 w2934 w2955 w2976 w3004 w3024 w3051 w3071 w3095 w3129 w3162] -> w1052
            tunnel: w1173 -> [w1200 w1219 w1241 w1296 w1344 w1411 w1475 w1539 w1583 w1609 w1668 w1696 w1705 w1724 w1758 w1788 w1823 w1847 w1873 w1902 w1943 w1980 w2010 w2037 w2053 w2075 w2094 w2113 w2147 w2194 w2219 w2247 w2268 w2289 w2308 w2327 w2356 w2429 w2454 w2477 w2491 w2541 w2565 w2597 w2618 w2638 w2669 w2692 w2704 w2723 w2765 w2784 w2827 w2844 w2858 w2892 w2913 w2934 w2955 w2976 w3004 w3024 w3051 w3071 w3095 w3129 w3162]
            tunnel: w1172 -> [w1203 w1222 w1238 w1299 w1347 w1414 w1478 w1542 w1586 w1612 w1671 w1690 w1716 w1743 w1776 w1804 w1837 w1860 w1886 w1915 w1930 w1961 w2013 w2040 w2059 w2078 w2097 w2116 w2127 w2171 w2227 w2254 w2273 w2292 w2311 w2330 w2354 w2427 w2464 w2487 w2522 w2549 w2576 w2600 w2617 w2650 w2674 w2689 w2712 w2722 w2776 w2810 w2831 w2841 w2867 w2895 w2916 w2937 w2958 w2979 w3007 w3027 w3054 w3074 w3098 w3132 w3165]
            tunnel: w1167 -> [w1202 w1221 w1239 w1298 w1346 w1413 w1477 w1541 w1585 w1611 w1670 w1689 w1715 w1744 w1775 w1805 w1838 w1861 w1887 w1916 w1953 w1982 w2012 w2039 w2058 w2077 w2096 w2115 w2161 w2195 w2226 w2253 w2272 w2291 w2310 w2329 w2355 w2426 w2463 w2486 w2521 w2548 w2575 w2599 w2616 w2649 w2673 w2690 w2713 w2721 w2775 w2809 w2830 w2842 w2868 w2894 w2915 w2936 w2957 w2978 w3006 w3026 w3053 w3073 w3097 w3131 w3164]
            tunnel: w1166 -> [w1201 w1220 w1240 w1297 w1345 w1412 w1476 w1540 w1584 w1610 w1669 w1688 w1714 w1745 w1774 w1806 w1839 w1862 w1888 w1917 w1952 w1981 w2011 w2038 w2057 w2076 w2095 w2114 w2160 w2196 w2225 w2252 w2271 w2290 w2309 w2328 w2373 w2430 w2462 w2485 w2520 w2547 w2574 w2598 w2615 w2648 w2672 w2691 w2714 w2720 w2774 w2808 w2829 w2843 w2869 w2893 w2914 w2935 w2956 w2977 w3005 w3025 w3052 w3072 w3096 w3130 w3163]
            tunnel: [w1203 w1222 w1238 w1299 w1347 w1414 w1478 w1542 w1586 w1612 w1671 w1690 w1716 w1743 w1776 w1804 w1837 w1860 w1886 w1915 w1930 w1961 w2013 w2040 w2059 w2078 w2097 w2116 w2127 w2171 w2227 w2254 w2273 w2292 w2311 w2330 w2354 w2427 w2464 w2487 w2522 w2549 w2576 w2600 w2617 w2650 w2674 w2689 w2712 w2722 w2776 w2810 w2831 w2841 w2867 w2895 w2916 w2937 w2958 w2979 w3007 w3027 w3054 w3074 w3098 w3132 w3165] -> w1155
            tunnel: [w1202 w1221 w1239 w1298 w1346 w1413 w1477 w1541 w1585 w1611 w1670 w1689 w1715 w1744 w1775 w1805 w1838 w1861 w1887 w1916 w1953 w1982 w2012 w2039 w2058 w2077 w2096 w2115 w2161 w2195 w2226 w2253 w2272 w2291 w2310 w2329 w2355 w2426 w2463 w2486 w2521 w2548 w2575 w2599 w2616 w2649 w2673 w2690 w2713 w2721 w2775 w2809 w2830 w2842 w2868 w2894 w2915 w2936 w2957 w2978 w3006 w3026 w3053 w3073 w3097 w3131 w3164] -> w1154
            tunnel: [w1201 w1220 w1240 w1297 w1345 w1412 w1476 w1540 w1584 w1610 w1669 w1688 w1714 w1745 w1774 w1806 w1839 w1862 w1888 w1917 w1952 w1981 w2011 w2038 w2057 w2076 w2095 w2114 w2160 w2196 w2225 w2252 w2271 w2290 w2309 w2328 w2373 w2430 w2462 w2485 w2520 w2547 w2574 w2598 w2615 w2648 w2672 w2691 w2714 w2720 w2774 w2808 w2829 w2843 w2869 w2893 w2914 w2935 w2956 w2977 w3005 w3025 w3052 w3072 w3096 w3130 w3163] -> w1153
            tunnel: w1114 -> [w1199 w1218 w1237 w1263 w1320 w1388 w1474 w1538 w1582 w1607 w1628 w1695 w1704 w1741 w1747 w1789 w1818 w1844 w1872 w1901 w1942 w1966 w2004 w2036 w2054 w2074 w2093 w2112 w2131 w2191 w2218 w2251 w2269 w2288 w2307 w2326 w2340 w2407 w2446 w2482 w2493 w2546 w2566 w2596 w2614 w2639 w2671 w2688 w2701 w2725 w2747 w2782 w2826 w2845 w2870 w2889 w2910 w2931 w2952 w2963 w2993 w3012 w3036 w3068 w3084 w3107 w3140]
            tunnel: w1109 -> [w1198 w1217 w1236 w1294 w1342 w1408 w1472 w1536 w1580 w1600 w1664 w1694 w1713 w1740 w1755 w1787 w1825 w1850 w1876 w1905 w1945 w1979 w2003 w2034 w2056 w2073 w2092 w2111 w2149 w2193 w2216 w2246 w2270 w2287 w2306 w2325 w2366 w2428 w2460 w2484 w2514 w2542 w2567 w2594 w2613 w2641 w2668 w2687 w2711 w2728 w2746 w2801 w2825 w2846 w2871 w2888 w2909 w2930 w2951 w2964 w3001 w3021 w3032 w3067 w3092 w3126 w3159]
            tunnel: [w1199 w1218 w1237 w1263 w1320 w1387 w1474 w1538 w1582 w1607 w1650 w1679 w1704 w1729 w1747 w1789 w1818 w1843 w1871 w1900 w1946 w1965 w2005 w2035 w2054 w2074 w2093 w2112 w2156 w2190 w2217 w2249 w2269 w2288 w2307 w2326 w2367 w2404 w2461 w2481 w2515 w2545 w2568 w2595 w2614 w2642 w2670 w2688 w2700 w2724 w2747 w2780 w2826 w2845 w2870 w2889 w2910 w2931 w2952 w2963 w2993 w3012 w3036 w3068 w3084 w3107 w3140] -> w1150
            tunnel: [w1198 w1217 w1236 w1293 w1341 w1403 w1472 w1536 w1580 w1600 w1664 w1693 w1713 w1739 w1755 w1787 w1825 w1850 w1876 w1905 w1945 w1979 w2003 w2034 w2056 w2073 w2092 w2111 w2149 w2193 w2216 w2246 w2270 w2287 w2306 w2325 w2366 w2428 w2460 w2484 w2514 w2542 w2567 w2594 w2613 w2641 w2668 w2687 w2711 w2728 w2746 w2801 w2825 w2846 w2871 w2888 w2909 w2930 w2951 w2964 w3001 w3021 w3035 w3067 w3092 w3126 w3159] -> w1163
            tunnel: [_ _ _ _ _ _ _ _ _ _ _ _ _ _ _ _ _ _ _ _ _ _ _ _ _ _ _ _ _ _ _ _ _ _ _ _ _ _ _ w2475 _ _ _ _ _ _ _ _ _ _ _ _ _ _ _ _ _ _ _ _ _ _ _ _ _ _ _] -> w1125
            tunnel: [_ _ _ _ _ _ _ _ _ _ _ _ _ _ _ _ _ _ _ _ _ _ _ _ _ _ _ _ _ _ _ _ _ _ _ _ _ _ _ w2476 _ _ _ _ _ _ _ _ _ _ _ _ _ _ _ _ _ _ _ _ _ _ _ _ _ _ _] -> w1127
            tunnel: w1162 -> [w1196 w1215 w1234 w1265 w1322 w1409 w1473 w1537 w1581 w1605 w1665 w1691 w1706 w1737 w1767 w1802 w1835 w1840 w1868 w1897 w1944 w1978 w2000 w2030 w2055 w2071 w2090 w2109 w2155 w2192 w2215 w2244 w2266 w2285 w2304 w2323 w2365 w2424 w2452 w2483 w2495 w2539 w2564 w2592 w2611 w2640 w2667 w2685 w2703 w2730 w2772 w2793 w2823 w2848 w2873 w2886 w2907 w2928 w2949 w2973 w2987 w3014 w3042 w3061 w3086 w3120 w3153]
            tunnel: [w1196 w1215 w1234 w1265 w1322 w1409 w1473 w1537 w1581 w1605 w1665 w1691 w1703 w1737 w1767 w1802 w1835 w1840 w1868 w1897 w1944 w1978 w2000 w2030 w2055 w2071 w2090 w2109 w2155 w2192 w2215 w2244 w2266 w2285 w2304 w2323 w2365 w2424 w2452 w2483 w2494 w2539 w2564 w2592 w2611 w2640 w2667 w2685 w2702 w2730 w2772 w2793 w2823 w2848 w2873 w2886 w2907 w2928 w2949 w2973 w2987 w3014 w3042 w3061 w3086 w3120 w3153] -> w1161
            tunnel: w1160 -> [w1197 w1216 w1235 w1264 w1321 w1410 w1470 w1534 w1578 w1606 w1666 w1692 w1712 w1738 w1746 w1803 w1836 w1848 w1874 w1903 w1941 w1960 w2001 w2031 w2052 w2072 w2091 w2110 w2154 w2170 w2214 w2245 w2267 w2286 w2305 w2324 w2364 w2425 w2453 w2478 w2512 w2540 w2563 w2593 w2612 w2637 w2666 w2686 w2710 w2729 w2773 w2800 w2824 w2847 w2872 w2887 w2908 w2929 w2950 w2974 w3000 w3020 w3048 w3059 w3091 w3125 w3158]
            tunnel: [w1197 w1216 w1235 w1264 w1321 w1410 w1471 w1535 w1579 w1606 w1666 w1692 w1712 w1738 w1746 w1803 w1836 w1848 w1874 w1903 w1941 w1960 w2001 w2031 w2052 w2072 w2091 w2110 w2154 w2170 w2214 w2245 w2267 w2286 w2305 w2324 w2364 w2425 w2453 w2478 w2512 w2540 w2563 w2593 w2612 w2637 w2666 w2686 w2710 w2729 w2773 w2800 w2824 w2847 w2872 w2887 w2908 w2929 w2950 w2974 w3000 w3020 w3048 w3059 w3091 w3125 w3158] -> w1159
            tunnel: [_ _ _ _ _ _ _ _ _ _ _ _ _ _ _ _ _ _ _ _ _ _ _ _ _ _ _ _ _ _ _ _ _ _ _ _ _ _ _ _ _ _ _ _ _ _ _ _ _ _ _ _ TRUE _ _ _ _ _ _ _ _ _ _ _ _ _ _] -> w1156
            tunnel: w1146 -> [w1194 w1213 w1232 w1255 w1315 w1398 w1457 w1521 w1550 _ w1656 w1687 w1711 w1736 w1766 w1801 w1834 w1859 w1885 w1914 w1940 w1977 w1998 w2029 w2050 w2069 w2088 w2107 w2153 w2187 w2212 w2243 w2264 w2283 w2302 w2321 w2363 w2423 w2442 w2474 w2510 w2538 w2561 w2591 w2610 w2635 w2665 w2684 w2708 w2734 w2771 w2797 w2821 w2839 w2866 w2884 w2905 w2926 w2947 w2971 w2998 w3018 w3046 w3065 w3090 w3124 w3157]
            tunnel: w1145 -> [w1193 w1212 w1231 w1254 w1314 w1397 w1456 w1520 w1551 _ w1655 w1686 w1710 w1735 w1765 w1800 w1833 w1858 w1884 w1913 w1939 w1976 w1997 w2028 w2049 w2068 w2087 w2106 w2152 w2186 w2211 w2242 w2263 w2282 w2301 w2320 w2362 w2422 w2441 w2473 w2509 w2537 w2560 w2590 w2609 w2634 w2664 w2683 w2707 w2733 w2770 w2796 w2820 w2838 w2865 w2883 w2904 w2925 w2946 w2970 w2997 w3017 w3045 w3064 w3089 w3123 w3156]
            tunnel: w1144 -> [w1192 w1211 w1230 w1253 w1313 w1396 w1455 w1519 w1552 _ w1654 w1685 w1709 w1734 w1764 w1799 w1832 w1857 w1883 w1912 w1938 w1975 w1996 w2027 w2048 w2067 w2086 w2105 w2151 w2185 w2210 w2241 w2262 w2281 w2300 w2319 w2361 w2421 w2440 w2472 w2508 w2536 w2559 w2589 w2608 w2633 w2663 w2682 w2706 w2732 w2769 w2795 w2819 w2837 w2864 w2882 w2903 w2924 w2945 w2969 w2996 w3016 w3044 w3063 w3088 w3122 w3155]
            tunnel: w1143 -> [w1191 w1210 w1229 w1252 w1312 w1395 w1454 w1518 w1553 _ w1653 w1684 w1708 w1733 w1763 w1798 w1831 w1856 w1882 w1911 w1937 w1974 w1995 w2026 w2047 w2066 w2085 w2104 w2150 w2184 w2209 w2240 w2261 w2280 w2299 w2318 w2360 w2420 w2439 w2471 w2507 w2535 w2558 w2588 w2607 w2632 w2662 w2681 w2705 w2731 w2768 w2794 w2818 w2836 w2863 w2881 w2902 w2923 w2944 w2968 w2995 w3015 w3043 w3062 w3087 w3121 w3154]
            tunnel: w1142 -> [_ _ _ _ _ _ _ _ _ _ _ _ _ _ _ _ _ _ _ _ _ _ _ _ _ _ _ _ _ w2189 _ _ _ _ _ _ _ _ _ _ _ _ _ _ _ _ _ _ _ _ _ _ _ _ _ _ _ _ _ _ _ _ _ _ _ _ _]
            tunnel: w1141 -> [_ _ _ _ _ _ _ _ _ _ _ _ _ _ _ _ _ _ _ _ _ _ _ _ _ _ _ _ _ w2188 _ _ _ _ _ _ _ _ _ _ _ _ _ _ _ _ _ _ _ _ _ _ _ _ _ _ _ _ _ _ _ _ _ _ _ _ _]
            tunnel: [w1194 w1213 w1232 w1255 w1315 w1398 w1457 w1521 w1550 w1599 w1656 w1687 w1711 w1736 w1766 w1801 w1834 w1859 w1885 w1914 w1940 w1977 w1998 w2029 w2050 w2069 w2088 w2107 w2153 w2187 w2212 w2243 w2264 w2283 w2302 w2321 w2363 w2423 w2442 w2474 w2510 w2538 w2561 w2591 w2610 w2635 w2665 w2684 w2708 w2734 w2771 w2797 w2821 w2839 w2866 w2884 w2905 w2926 w2947 w2971 w2998 w3018 w3046 w3065 w3090 w3124 w3157] -> w1138
            tunnel: [w1193 w1212 w1231 w1254 w1314 w1397 w1456 w1520 w1551 w1590 w1655 w1686 w1710 w1735 w1765 w1800 w1833 w1858 w1884 w1913 w1939 w1976 w1997 w2028 w2049 w2068 w2087 w2106 w2152 w2186 w2211 w2242 w2263 w2282 w2301 w2320 w2362 w2422 w2441 w2473 w2509 w2537 w2560 w2590 w2609 w2634 w2664 w2683 w2707 w2733 w2770 w2796 w2820 w2838 w2865 w2883 w2904 w2925 w2946 w2970 w2997 w3017 w3045 w3064 w3089 w3123 w3156] -> w1106
            tunnel: [w1192 w1211 w1230 w1253 w1313 w1396 w1455 w1519 w1552 w1598 w1654 w1685 w1709 w1734 w1764 w1799 w1832 w1857 w1883 w1912 w1938 w1975 w1996 w2027 w2048 w2067 w2086 w2105 w2151 w2185 w2210 w2241 w2262 w2281 w2300 w2319 w2361 w2421 w2440 w2472 w2508 w2536 w2559 w2589 w2608 w2633 w2663 w2682 w2706 w2732 w2769 w2795 w2819 w2837 w2864 w2882 w2903 w2924 w2945 w2969 w2996 w3016 w3044 w3063 w3088 w3122 w3155] -> w1139
            tunnel: [w1191 w1210 w1229 w1252 w1312 w1395 w1454 w1518 w1553 w1588 w1653 w1684 w1708 w1733 w1763 w1798 w1831 w1856 w1882 w1911 w1937 w1974 w1995 w2026 w2047 w2066 w2085 w2104 w2150 w2184 w2209 w2240 w2261 w2280 w2299 w2318 w2360 w2420 w2439 w2471 w2507 w2535 w2558 w2588 w2607 w2632 w2662 w2681 w2705 w2731 w2768 w2794 w2818 w2836 w2863 w2881 w2902 w2923 w2944 w2968 w2995 w3015 w3043 w3062 w3087 w3121 w3154] -> w1140
            tunnel: [_ _ _ _ _ _ _ _ _ _ _ _ _ _ _ _ _ _ _ _ _ _ _ _ _ _ _ _ w2140 w2189 _ _ _ _ _ _ _ _ _ _ _ _ _ _ _ _ _ _ _ _ _ _ _ _ _ _ _ _ _ _ _ _ _ _ _ _ _] -> w1108
            tunnel: [_ _ _ _ _ _ _ _ _ _ _ _ _ _ _ _ _ _ _ _ _ _ _ _ _ _ _ _ w2139 w2188 _ _ _ _ _ _ _ _ _ _ _ _ _ _ _ _ _ _ _ _ _ _ _ _ _ _ _ _ _ _ _ _ _ _ _ _ _] -> w1107
            tunnel: w1121 -> [w1190 w1209 w1228 w1251 w1311 w1394 w1453 w1517 w1549 w1597 w1663 w1683 w1707 w1732 w1749 w1791 w1817 w1842 w1870 w1899 w1936 w1973 w1994 w2025 w2046 w2065 w2084 w2103 w2138 w2183 w2208 w2239 w2260 w2279 w2298 w2317 w2359 w2419 w2436 w2470 w2506 w2534 w2555 w2582 w2606 w2629 w2656 w2680 w2699 w2727 w2761 w2792 w2817 w2849 w2874 w2885 w2906 w2927 w2948 w2972 w2999 w3019 w3047 w3066 w3081 w3119 w3152]
            tunnel: [w1190 w1209 w1228 w1251 w1311 w1394 w1453 w1517 w1549 w1597 w1663 w1683 w1707 w1732 w1748 w1790 w1810 w1841 w1869 w1898 w1936 w1973 w1994 w2025 w2046 w2065 w2084 w2103 w2138 w2183 w2208 w2239 w2260 w2279 w2298 w2317 w2359 w2419 w2436 w2470 w2506 w2534 w2555 w2582 w2606 w2629 w2656 w2680 w2699 w2726 w2761 w2792 w2817 w2849 w2874 w2885 w2906 w2927 w2948 w2972 w2999 w3019 w3047 w3066 w3081 w3119 w3152] -> w1120
            tunnel: [w1189 w1208 w1227 w1250 w1310 w1393 w1452 w1516 w1548 w1596 w1662 w1682 w1718 w1731 w1769 w1797 w1830 w1855 w1881 w1910 w1935 w1972 w1993 w2024 w2045 w2064 w2083 w2102 w2137 w2182 w2207 w2238 w2259 w2278 w2297 w2316 w2358 w2418 w2435 w2469 w2505 w2533 w2554 w2581 w2605 w2628 w2655 w2679 w2698 w2719 w2767 w2791 w2815 w2850 w2860 w2880 w2901 w2922 w2943 w2967 w3003 w3023 w3050 w3070 w3094 w3128 w3161] -> w1119
            tunnel: [w1188 w1207 w1226 w1249 w1309 w1392 w1451 w1515 w1547 w1595 w1661 w1681 w1717 w1730 w1768 w1796 w1829 w1854 w1880 w1909 w1934 w1971 w1992 w2023 w2044 w2063 w2082 w2101 w2136 w2181 w2206 w2237 w2258 w2277 w2296 w2315 w2357 w2417 w2434 w2468 w2504 w2532 w2553 w2580 w2604 w2627 w2654 w2678 w2697 w2718 w2766 w2790 w2816 w2832 w2857 w2890 w2911 w2932 w2953 w2975 w3002 w3022 w3049 w3069 w3093 w3127 w3160] -> w1118
            tunnel: w1117 -> [w1189 w1208 w1227 w1250 w1310 w1393 w1452 w1516 w1548 w1596 w1662 w1682 w1718 w1731 w1769 w1797 w1830 w1855 w1881 w1910 w1935 w1972 w1993 w2024 w2045 w2064 w2083 w2102 w2137 w2182 w2207 w2238 w2259 w2278 w2297 w2316 w2358 w2418 w2435 w2469 w2505 w2533 w2554 w2581 w2605 w2628 w2655 w2679 w2698 w2719 w2767 w2791 w2815 _ w2860 w2880 w2901 w2922 w2943 w2967 w3003 w3023 w3050 w3070 w3094 w3128 w3161]
            tunnel: w1116 -> [w1188 w1207 w1226 w1249 w1309 w1392 w1451 w1515 w1547 w1595 w1661 w1681 w1717 w1730 w1768 w1796 w1829 w1854 w1880 w1909 w1934 w1971 w1992 w2023 w2044 w2063 w2082 w2101 w2136 w2181 w2206 w2237 w2258 w2277 w2296 w2315 w2357 w2417 w2434 w2468 w2504 w2532 w2553 w2580 w2604 w2627 w2654 w2678 w2697 w2718 w2766 w2790 w2816 _ w2857 w2890 w2911 w2932 w2953 w2975 w3002 w3022 w3049 w3069 w3093 w3127 w3160]
            tunnel: w1115 -> [_ _ _ _ _ _ _ _ _ _ _ _ _ _ _ _ _ _ _ _ _ _ _ _ _ _ _ _ _ _ _ _ _ _ _ _ _ _ _ _ _ _ _ _ _ _ _ _ _ _ _ _ _ _ _ w2878 w2899 w2920 w2941 w2965 _ _ _ _ _ _ _]
            tunnel: w1113 -> [_ _ _ _ _ _ _ _ _ _ _ _ _ _ _ _ w1822 _ w1865 w1896 w1924 w1959 w1986 w2016 _ _ _ _ w2120 w2165 w2202 w2231 _ _ _ _ _ _ _ _ _ _ _ _ _ _ _ _ _ _ _ _ _ _ _ _ _ _ _ _ _ _ _ _ _ _ _]
            tunnel: w1110 -> [_ _ _ _ _ _ _ _ _ _ _ _ _ _ _ _ _ _ _ _ _ _ _ _ _ _ _ _ _ _ _ _ _ _ _ _ _ _ _ _ _ _ _ _ _ _ _ _ _ _ _ _ _ _ _ _ _ _ _ _ _ _ w3037 _ _ _ _]
            tunnel: [w1187 w1206 w1225 w1248 w1308 w1391 w1450 w1514 w1546 w1594 w1660 w1677 w1701 w1727 w1770 w1795 w1828 w1853 w1879 w1908 w1933 w1970 w1991 w2022 w2043 w2062 w2081 w2100 w2135 w2180 w2205 w2236 w2257 w2276 w2295 w2314 w2353 w2416 w2433 w2467 w2489 w2531 w2552 w2579 w2603 w2626 w2653 w2677 w2696 w2717 w2764 w2777 w2814 w2835 w2859 w2877 w2898 w2919 w2940 w2962 w2982 w3011 w3031 w3058 w3079 w3118 w3151] -> w1104
            tunnel: w1105 -> [w1187 w1206 w1225 w1248 w1308 w1391 w1450 w1514 w1546 w1594 w1660 w1677 _ w1727 w1770 w1795 w1828 w1853 w1879 w1908 w1933 w1970 w1991 w2022 w2043 w2062 w2081 w2100 w2135 w2180 w2205 w2236 w2257 w2276 w2295 w2314 w2353 w2416 w2433 w2467 w2489 w2531 w2552 w2579 w2603 w2626 w2653 w2677 w2696 w2717 w2764 w2778 w2814 w2835 w2859 w2877 w2898 w2919 w2940 w2962 w2982 w3011 w3031 w3058 w3079 w3118 w3151]
            tunnel: w1103 -> [w1186 w1205 w1224 w1247 w1307 w1390 w1449 w1513 w1545 w1593 w1659 w1676 w1700 w1726 w1762 w1794 w1827 w1852 w1878 w1907 w1932 w1969 w1990 w2021 w2042 w2061 w2080 w2099 w2134 w2179 w2204 w2235 w2256 w2275 w2294 w2313 w2352 w2415 w2432 w2466 w2503 w2530 w2551 w2578 w2602 w2625 w2652 w2676 w2695 w2716 w2763 w2789 w2813 w2834 w2862 w2876 w2897 w2918 w2939 w2961 w2981 w3010 w3030 w3057 w3078 w3117 w3150]
            tunnel: w1102 -> [w1185 w1204 w1223 w1246 w1306 w1389 w1448 w1512 w1544 w1592 w1658 w1675 w1699 w1725 w1761 w1793 w1826 w1851 w1877 w1906 w1931 w1968 w1989 w2020 w2041 w2060 w2079 w2098 w2133 w2178 w2203 w2234 w2255 w2274 w2293 w2312 w2351 w2414 w2431 w2465 w2500 w2529 w2550 w2577 w2601 w2624 w2651 w2675 w2694 w2715 w2762 w2788 w2812 w2833 w2861 w2875 w2896 w2917 w2938 w2960 w2980 w3009 w3029 w3056 w3077 w3116 w3149]
            tunnel: [w1186 w1205 w1224 w1247 w1307 w1390 w1449 w1513 w1545 w1593 w1659 w1676 w1700 w1726 w1762 w1794 w1827 w1852 w1878 w1907 w1932 w1969 w1990 w2021 w2042 w2061 w2080 w2099 w2134 w2179 w2204 w2235 w2256 w2275 w2294 w2313 w2352 w2415 w2432 w2466 w2502 w2530 w2551 w2578 w2602 w2625 w2652 w2676 w2695 w2716 w2763 w2789 w2813 w2834 w2862 w2876 w2897 w2918 w2939 w2961 w2981 w3010 w3030 w3057 w3078 w3117 w3150] -> w1101
            tunnel: [w1185 w1204 w1223 w1246 w1306 w1389 w1448 w1512 w1544 w1592 w1658 w1675 w1699 w1725 w1761 w1793 w1826 w1851 w1877 w1906 w1931 w1968 w1989 w2020 w2041 w2060 w2079 w2098 w2133 w2178 w2203 w2234 w2255 w2274 w2293 w2312 w2351 w2414 w2431 w2465 w2501 w2529 w2550 w2577 w2601 w2624 w2651 w2675 w2694 w2715 w2762 w2788 w2812 w2833 w2861 w2875 w2896 w2917 w2938 w2960 w2980 w3009 w3029 w3056 w3077 w3116 w3149] -> w1100
            tunnel: w1099 -> [_ _ _ _ _ _ _ _ _ _ w1651 _ _ _ w1773 w1783 _ _ _ _ _ _ _ _ _ _ _ _ _ w2175 _ _ _ _ _ _ w2349 w2413 _ _ _ _ _ _ _ w2623 _ _ _ _ w2743 _ _ _ _ _ _ _ _ _ _ _ _ _ _ _ _]
            tunnel: w1098 -> [_ _ _ _ _ _ _ _ _ _ w1652 _ _ _ w1772 w1782 _ _ _ _ _ _ _ _ _ _ _ _ _ w2174 _ _ _ _ _ _ w2350 w2412 _ _ _ _ _ _ _ w2622 _ _ _ _ w2742 _ _ _ _ _ _ _ _ _ _ _ _ _ _ _ _]
            tunnel: w1096 -> [_ _ _ _ _ _ _ _ _ _ _ _ _ _ _ _ w1821 _ w1864 w1895 w1923 w1958 w1985 w2017 _ _ _ _ w2119 w2164 w2201 w2230 _ _ _ _ _ _ _ _ _ _ _ _ _ _ _ _ _ _ _ _ _ _ _ _ _ _ _ _ _ _ _ _ _ _ _]
            tunnel: w1095 -> [_ _ _ _ _ _ _ _ _ _ _ _ _ _ _ _ w1820 _ _ w1892 w1926 w1963 w1988 w2018 _ _ _ _ w2125 w2169 w2200 w2233 _ _ _ _ _ _ _ _ _ _ _ _ _ _ _ _ _ _ _ _ _ _ _ _ _ _ _ _ _ _ _ _ _ _ _]
            tunnel: w1094 -> [_ _ _ _ _ _ _ _ _ _ _ _ _ _ _ _ w1819 _ _ w1891 w1925 w1962 w1987 w2019 _ _ _ _ w2124 w2168 w2199 w2232 _ _ _ _ _ _ _ _ _ _ _ _ _ _ _ _ _ _ _ _ _ _ _ _ _ _ _ _ _ _ _ _ _ _ _]
            tunnel: [_ _ _ _ _ _ _ _ _ _ _ _ _ _ _ _ w1820 _ w1867 w1892 w1926 w1963 w1988 w2018 _ _ _ _ w2125 w2169 w2200 w2233 _ _ _ _ _ _ _ _ _ _ _ _ _ _ _ _ _ _ _ _ _ _ _ _ _ _ _ _ _ _ _ _ _ _ _] -> w1093
            tunnel: [_ _ _ _ _ _ _ _ _ _ _ _ _ _ _ _ w1819 _ w1866 w1891 w1925 w1962 w1987 w2019 _ _ _ _ w2124 w2168 w2199 w2232 _ _ _ _ _ _ _ _ _ _ _ _ _ _ _ _ _ _ _ _ _ _ _ _ _ _ _ _ _ _ _ _ _ _ _] -> w1092
            tunnel: [_ _ _ _ _ _ _ _ _ _ _ _ _ _ _ _ w1822 w1845 w1865 w1896 w1924 w1959 w1986 w2016 _ _ _ _ w2120 w2165 w2202 w2231 _ _ _ _ _ _ _ _ _ _ _ _ _ _ _ _ _ _ _ _ _ _ _ _ _ _ _ _ _ _ _ _ _ _ _] -> w1091
            tunnel: [_ _ _ _ _ _ _ _ _ _ _ _ _ _ _ _ w1821 w1846 w1864 w1895 w1923 w1958 w1985 w2017 _ _ _ _ w2119 w2164 w2201 w2230 _ _ _ _ _ _ _ _ _ _ _ _ _ _ _ _ _ _ _ _ _ _ _ _ _ _ _ _ _ _ _ _ _ _ _] -> w1090
            tunnel: [_ _ _ _ _ _ _ _ _ _ _ _ _ _ _ _ _ _ _ _ _ w1957 _ _ _ _ _ _ _ w2166 _ _ _ _ _ _ w2332 w2391 _ _ _ _ _ _ _ _ _ _ _ _ _ _ _ _ _ _ _ _ _ _ _ _ _ _ _ _ _] -> w1087
            tunnel: [_ _ _ _ _ _ _ _ _ _ _ _ _ _ _ _ _ _ _ _ _ w1956 _ _ _ _ _ _ _ w2167 _ _ _ _ _ _ w2331 w2392 _ _ _ _ _ _ _ _ _ _ _ _ _ _ _ _ _ _ _ _ _ _ _ _ _ _ _ _ _] -> w1089
            tunnel: [_ _ _ _ _ _ _ _ _ _ _ _ _ _ _ _ _ _ w1863 w1894 _ _ _ _ _ _ _ _ _ _ _ _ _ _ _ _ _ _ _ _ _ _ _ _ _ _ _ _ _ _ _ _ _ _ _ _ _ _ _ _ _ _ _ _ _ _ _] -> w1084
            tunnel: [_ _ _ _ _ _ _ _ _ _ _ _ _ _ _ _ _ _ _ TRUE ("Recording") _ _ _ _ _ _ _ _ _ _ _ _ _ _ _ _ _ _ _ _ _ _ _ _ _ _ _ _ _ _ _ _ _ _ _ _ _ _ _ _ _ _ _ _ _ _ _] -> w1081
            tunnel: [_ _ _ _ _ _ _ _ _ _ _ _ _ _ _ _ _ _ w1863 _ _ _ _ _ _ _ _ _ _ _ _ _ _ _ _ _ _ _ _ _ _ _ _ _ _ _ _ _ _ _ _ _ _ _ _ _ _ _ _ _ _ _ _ _ _ _ _] -> w1077
            tunnel: [_ _ _ _ _ _ _ _ _ _ _ TRUE _ _ _ _ _ _ _ _ _ _ _ _ _ _ _ _ _ _ _ _ _ _ _ _ _ _ _ _ _ _ _ _ _ _ _ _ _ _ _ _ _ _ _ _ _ _ _ _ _ _ _ _ _ _ _] -> w1074
            tunnel: [_ _ _ _ _ _ _ _ _ _ _ w1672 _ _ _ _ _ _ _ _ _ _ _ _ _ _ _ _ _ _ _ _ _ _ _ _ _ _ _ _ _ _ _ _ _ _ _ _ _ _ _ _ _ _ _ _ _ _ _ _ _ _ _ _ _ _ _] -> w1072
            tunnel: [_ _ _ _ _ _ _ _ _ _ _ _ _ TRUE _ _ _ _ _ _ _ _ _ _ _ _ _ _ _ _ _ _ _ _ _ _ _ _ _ _ _ _ _ _ _ _ _ _ _ _ _ _ _ _ _ _ _ _ _ _ _ _ _ _ _ _ _] -> w1071
            tunnel: [_ _ _ _ _ _ _ _ _ _ _ _ _ w1719 _ _ _ _ _ _ _ _ _ _ _ _ _ _ _ _ _ _ _ _ _ _ _ _ _ _ _ _ _ _ _ _ _ _ _ _ _ _ _ _ _ _ _ _ _ _ _ _ _ _ _ _ _] -> w1070
            tunnel: w1059 -> [_ _ _ _ _ _ _ _ _ _ _ _ _ _ _ _ w1808 _ _ _ w1919 w1955 w1984 w2015 _ _ _ _ w2118 w2163 w2198 w2229 _ _ _ _ w2335 w2386 _ _ _ _ _ _ _ _ _ _ _ _ _ _ _ _ _ _ _ _ _ _ _ _ _ _ _ _ _]
            tunnel: [_ _ _ _ _ _ _ _ _ _ _ _ _ _ _ _ w1808 _ _ w1890 w1919 w1955 w1984 w2015 _ _ _ _ w2118 w2163 w2198 w2229 _ _ _ _ w2335 w2386 _ _ _ _ _ _ _ _ _ _ _ _ _ _ _ _ _ _ _ _ _ _ _ _ _ _ _ _ _] -> w1058
            tunnel: w1057 -> [_ _ _ _ _ _ _ _ _ _ _ _ _ _ _ _ w1807 _ _ _ w1918 w1954 w1983 w2014 _ _ _ _ w2117 w2162 w2197 w2228 _ _ _ _ w2333 w2390 _ _ _ _ _ _ _ _ _ _ _ _ _ _ _ _ _ _ _ _ _ _ _ _ _ _ _ _ _]
            tunnel: [_ _ _ _ _ _ _ _ _ _ _ _ _ _ _ _ w1807 _ _ w1889 w1918 w1954 w1983 w2014 _ _ _ _ w2117 w2162 w2197 w2228 _ _ _ _ w2333 w2390 _ _ _ _ _ _ _ _ _ _ _ _ _ _ _ _ _ _ _ _ _ _ _ _ _ _ _ _ _] -> w1056
            tunnel: w1051 -> [_ _ _ _ _ _ _ _ _ _ _ _ _ _ _ _ _ _ _ _ _ _ _ _ _ _ _ _ _ _ _ _ _ _ _ _ _ _ _ _ _ _ _ _ _ _ _ _ _ _ _ _ _ _ _ _ _ _ _ _ _ _ _ _ _ w3114 w3147]
            tunnel: [_ _ _ _ _ _ _ _ _ _ _ _ _ _ _ _ _ _ _ _ _ _ _ _ _ _ _ _ _ _ _ _ _ _ _ _ _ _ _ _ _ _ _ _ _ _ _ _ _ _ _ _ _ _ _ _ _ _ _ _ _ _ _ _ _ w3112 w3145] -> w1050
            frame 0, Default {
            }
            frame 1 {
            }
            frame 2 {
            }
            frame 3 {
              n607 = call "myRIO_BRig_RT_dataExp_Audio_freq__L.vi"() -> ("output_Audio_freq__L"=w1271:i32)  [unwired: 11 in]
              n608 = call "myRIO_BRig_RT_dataExp_Audio_freq__R.vi"() -> ("output_Audio_freq__R"=w1270:i32)  [unwired: 11 in]
              n609 = call "myRIO_BRig_RT_dataExp_Audio_amp__L.vi"() -> ("output_Audio_amp__L"=w1269:i32)  [unwired: 11 in]
              n610 = call "myRIO_BRig_RT_dataExp_Audio_amp__R.vi"() -> ("output_Audio_amp__R"=w1267:i32)  [unwired: 11 in]
              n611 = call "myRIO_BRig_RT_dataExp_TPB_min__L.vi"() -> ("output_TPB_min__L"=w1279:i32)  [unwired: 11 in]
              n612 = call "myRIO_BRig_RT_dataExp_TPB_min__R.vi"() -> ("output_TPB_min__R"=w1277:i32)  [unwired: 11 in]
              n613 = call "myRIO_BRig_RT_dataExp_TPB_max__L.vi"() -> ("output_TPB_max__L"=w1275:i32)  [unwired: 11 in]
              n614 = call "myRIO_BRig_RT_dataExp_TPB_max__R.vi"() -> ("output_TPB_max__R"=w1273:i32)  [unwired: 11 in]
              n615 = call "myRIO_BRig_RT_dataExp_ItrialUntilReward.vi"() -> ("output_I_trialUntilReward"=w1292:i32)  [unwired: 11 in]
              n616 = call "myRIO_BRig_RT_dataExp_IblockUntilReward.vi"() -> ("output_I_blockUntilReward"=w1288:i32)  [unwired: 11 in]
              n617 = call "myRIO_BRig_RT_dataExp_CueCycles.vi"() -> ("output_CueCycles"=w1287:i32)  [unwired: 11 in]
              n618 = call "myRIO_BRig_RT_dataExp_ENL_min.vi"() -> ("output_ENL_min"=w1285:i32)  [unwired: 11 in]
              n619 = call "myRIO_BRig_RT_dataExp_ENL_max.vi"() -> ("output_ENL_max"=w1283:i32)  [unwired: 11 in]
              n620 = call "myRIO_BRig_RT_dataExp_ENL_penalty.vi"() -> ("output_ENL_penalty"=w1281:i32)  [unwired: 11 in]
              n621 = local read "Audio_Freq__L"() -> (w1245:u8)
              n622 = local read "Audio_Freq__R"() -> (w1243:u8)
              n623 = local read "Audio_Amp__L"() -> (w1268:u16)
              n624 = local read "TpB_Min_L"() -> (w1278:u16)
              n625 = local read "TpB_Min_R"() -> (w1276:u16)
              n626 = local read "TpB_Max_L"() -> (w1274:u16)
              n627 = local read "TpB_Max_R"() -> (w1272:u16)
              n628 = local read "Audio_Amp__R"() -> (w1266:u16)
              n629 = local read "TrialUntilReward"() -> (w1291:bool)
              n630 = local read "CueCycles"() -> (w1286:u16)
              n631 = local read "Tcycle_ENL_min"() -> (w1284:u16)
              n632 = local read "Tcycle_ENL_max"() -> (w1282:u16)
              n633 = local read "Tcycle_ENLPenalty"() -> (w1280:u16)
              n634 = To Unsigned Word Integer(number=w1243) -> (unsigned 16bit integer=w1242:u16)
              n635 = To Unsigned Word Integer(number=w1245) -> (unsigned 16bit integer=w1244:u16)
              n636 = Boolean To (0,1)(Boolean=w1291) -> (0, 1=w1290:i16)
              n637 = To Unsigned Word Integer(number=w1290) -> (unsigned 16bit integer=w1289:u16)
              n638 = local read "BUR_min"() -> (w1260:u16)
              n639 = local read "BUR_max"() -> (w1261:u16)
              n640 = Not Equal To 0?(x=w1260) -> (x != 0?=w1259:bool)
              n641 = Not Equal To 0?(x=w1261) -> (x != 0?=w1258:bool)
              n642 = And(x=w1259, y=w1258) -> (x .and. y?=w1257:bool)
              n643 = Boolean To (0,1)(Boolean=w1257) -> (0, 1=w1262:i16)
              n644 = To Unsigned Word Integer(number=w1262) -> (unsigned 16bit integer=w1256:u16)
              n645 = Replace Array Subset(array=w1294, new element #1=w1289, index #1=w1292, new element #2=w1256, index #2=w1288, new element #3=w1286, index #3=w1287, new element #4=w1284, index #4=w1285, new element #5=w1282, index #5=w1283, new element #6=w1280, index #6=w1281, new element #7=w1278, index #7=w1279, new element #8=w1276, index #8=w1277, new element #9=w1274, index #9=w1275, new element #10=w1272, index #10=w1273, new element #11=w1244, index #11=w1271, new element #12=w1242, index #12=w1270, new element #13=w1268, index #13=w1269, new element #14=w1266, index #14=w1267) -> (w1293:u16[])
            }
            frame 4 {
              n646 = call "myRIO_BRig_RT_dataExp_Tcycle_RewardPost.vi"() -> ("output_Tcycle_RewardPost"=w1331:i32)  [unwired: 11 in]
              n647 = call "myRIO_BRig_RT_dataExp_Tcycle_Wrong.vi"() -> ("output_Tcycle_Wrong"=w1329:i32)  [unwired: 11 in]
              n648 = call "myRIO_BRig_RT_dataExp_Tcycle_Timeout.vi"() -> ("output_Tcycle_Timeout"=w1327:i32)  [unwired: 11 in]
              n649 = call "myRIO_BRig_RT_dataExp_Tcycle_Cue_min.vi"() -> ("output_Tcycle_Cue_min"=w1325:i32)  [unwired: 11 in]
              n650 = call "myRIO_BRig_RT_dataExp_Tcycle_Cue_max.vi"() -> ("output_Tcycle_Cue_max"=w1324:i32)  [unwired: 11 in]
              n651 = call "myRIO_BRig_RT_dataExp_Tcycle_CuePenalty.vi"() -> ("output_Tcycle_CuePenalty"=w1323:i32)  [unwired: 11 in]
              n652 = call "myRIO_BRig_RT_dataExp_SolenoidProbability_L.vi"() -> ("output_SolenoidProbability_L"=w1303:i32)  [unwired: 11 in]
              n653 = call "myRIO_BRig_RT_dataExp_SolenoidProbability_R.vi"() -> ("output_SolenoidProbability_R"=w1302:i32)  [unwired: 11 in]
              n654 = call "myRIO_BRig_RT_dataExp_nBlock.vi"() -> ("output_nBlock"=w1340:i32)  [unwired: 11 in]
              n655 = call "myRIO_BRig_RT_dataExp_nTrial.vi"() -> ("output_nTrial"=w1339:i32)  [unwired: 11 in]
              n656 = call "myRIO_BRig_RT_dataExp_runTime_seconds.vi"() -> ("output_RunTime_minutes"=w1338:i32)  [unwired: 11 in]
              n657 = call "myRIO_BRig_RT_dataExp_Tcycle_Selection.vi"() -> ("output_Tcycle_Selection"=w1337:i32)  [unwired: 11 in]
              n658 = call "myRIO_BRig_RT_dataExp_Tcycle_Reward__L.vi"() -> ("output_Tcycle_Reward__L"=w1335:i32)  [unwired: 11 in]
              n659 = call "myRIO_BRig_RT_dataExp_Tcycle_Reward__R.vi"() -> ("output_Tcycle_Reward__R"=w1333:i32)  [unwired: 11 in]
              n660 = local read "Tcycle_RewardPost"() -> (w1330:u16)
              n661 = local read "Tcycle_Wrong"() -> (w1328:u16)
              n662 = local read "Tcycle_Timeout"() -> (w1326:u16)
              n663 = local read "Tcycle_CuePenalty"() -> (w1316:u16)
              n664 = local read "Tcycle_Cue_max"() -> (w1304:u16)
              n665 = local read "Tcycle_Cue_min"() -> (w1305:u16)
              n666 = local read "Tcycle_Selection"() -> (w1336:u16)
              n667 = local read "Tcycle_Reward_L"() -> (w1334:u16)
              n668 = local read "Tcycle_Reward_R"() -> (w1332:u16)
              n669 = local read "SolenoidProbability_R"() -> (w1300:u16)
              n670 = local read "SolenoidProbability_L"() -> (w1301:u16)
              n671 = Replace Array Subset(array=w1342, new element #1=u16 0, index #1=w1340, new element #2=u16 0, index #2=w1339, new element #3=u16 0, index #3=w1338, new element #4=w1336, index #4=w1337, new element #5=w1334, index #5=w1335, new element #6=w1332, index #6=w1333, new element #7=w1330, index #7=w1331, new element #8=w1328, index #8=w1329, new element #9=w1326, index #9=w1327, new element #10=w1305, index #10=w1325, new element #11=w1304, index #11=w1324, new element #12=w1316, index #12=w1323, new element #13=w1301, index #13=w1303, new element #14=w1300, index #14=w1302) -> (w1341:u16[])
            }
            frame 5 {
              w1352 = 100.0 ("y")
              n672 = call "myRIO_BRig_RT_dataExp_laser1_Freq.vi"() -> ("output_laser1_Freq"=w1385:i32)  [unwired: 11 in]
              n673 = call "myRIO_BRig_RT_dataExp_laser1_Tpeak.vi"() -> ("output_laser1_Tpeak"=w1380:i32)  [unwired: 11 in]
              n674 = call "myRIO_BRig_RT_dataExp_laser1_Tshutter.vi"() -> ("output_laser1_Tshutter"=w1375:i32)  [unwired: 11 in]
              n675 = call "myRIO_BRig_RT_dataExp_FPGA_f_count2ms.vi"() -> ("output_FPGA_f_count2ms"=w1370:i32)  [unwired: 11 in]
              n676 = call "myRIO_BRig_RT_dataExp_laser1_Power_min.vi"() -> ("output_laser1_Power_min"=w1365:i32)  [unwired: 11 in]
              n677 = call "myRIO_BRig_RT_dataExp_laser1_Power_max.vi"() -> ("output_laser1_Power_max"=w1358:i32)  [unwired: 11 in]
              n678 = call "myRIO_BRig_RT_dataExp_laser1_Power_step.vi"() -> ("output_laser1_Power_step"=w1357:i32)  [unwired: 11 in]
              n679 = call "myRIO_BRig_RT_dataExp_laser1_duration.vi"() -> ("output_laser1_duration"=w1360:i32)  [unwired: 11 in]
              n680 = call "myRIO_BRig_RT_dataExp_BUR_min.vi"() -> ("output_BUR_min"=w1407:i32)  [unwired: 11 in]
              n681 = call "myRIO_BRig_RT_dataExp_BUR_max.vi"() -> ("output_BUR_max"=w1405:i32)  [unwired: 11 in]
              n682 = call "myRIO_BRig_RT_dataExp_Audio_sp__L.vi"() -> ("output_Audio_sp__L"=w1402:i32)  [unwired: 11 in]
              n683 = call "myRIO_BRig_RT_dataExp_Audio_sp__R.vi"() -> ("output_Audio_sp__R"=w1401:i32)  [unwired: 11 in]
              n684 = local read "laser_Tshutter"() -> (w1372:dbl)
              n685 = local read "f_millisec2count"() -> (w1367:dbl)
              n686 = local read "laser_Tpeak"() -> (w1377:dbl)
              n687 = local read "laser_power_min"() -> (w1362:dbl)
              n688 = local read "laser_power_max"() -> (w1351:dbl)
              n689 = local read "laser_power_step"() -> (w1350:dbl)
              n690 = local read "laser_Freq"() -> (w1384:dbl)
              n691 = local read "sp_LeftSpout"() -> (w1400:u16)
              n692 = local read "BUR_max"() -> (w1404:u16)
              n693 = local read "sp_RightSpout"() -> (w1399:u16)
              n694 = local read "BUR_min"() -> (w1406:u16)
              n695 = Multiply(x=w1384, y=w1352) -> (x*y=w1383:dbl)
              n696 = Multiply(x=w1377, y=w1352) -> (x*y=w1379:dbl)
              n697 = Multiply(x=w1372, y=w1352) -> (x*y=w1374:dbl)
              n698 = Multiply(x=w1367, y=w1352) -> (x*y=w1369:dbl)
              n699 = Multiply(x=w1362, y=w1352) -> (x*y=w1364:dbl)
              n700 = Multiply(x=w1351, y=w1352) -> (x*y=w1356:dbl)
              n701 = Multiply(x=w1350, y=w1352) -> (x*y=w1354:dbl)
              n702 = Round To Nearest(number=w1383) -> (nearest integer value=w1382:dbl)
              n703 = Round To Nearest(number=w1379) -> (nearest integer value=w1378:dbl)
              n704 = Round To Nearest(number=w1374) -> (nearest integer value=w1373:dbl)
              n705 = Round To Nearest(number=w1369) -> (nearest integer value=w1368:dbl)
              n706 = Round To Nearest(number=w1364) -> (nearest integer value=w1363:dbl)
              n707 = Round To Nearest(number=w1356) -> (nearest integer value=w1355:dbl)
              n708 = Round To Nearest(number=w1354) -> (nearest integer value=w1353:dbl)
              n709 = To Unsigned Word Integer(number=w1382) -> (unsigned 16bit integer=w1381:u16)
              n710 = To Unsigned Word Integer(number=w1378) -> (unsigned 16bit integer=w1376:u16)
              n711 = To Unsigned Word Integer(number=w1373) -> (unsigned 16bit integer=w1371:u16)
              n712 = To Unsigned Word Integer(number=w1368) -> (unsigned 16bit integer=w1366:u16)
              n713 = To Unsigned Word Integer(number=w1363) -> (unsigned 16bit integer=w1361:u16)
              n714 = To Unsigned Word Integer(number=w1355) -> (unsigned 16bit integer=w1349:u16)
              n715 = To Unsigned Word Integer(number=w1353) -> (unsigned 16bit integer=w1348:u16)
              n716 = local read "laser_duration"() -> (w1359:u16)
              n717 = call "myRIO_BRig_RT_dataCurrent_laser1_pulse_duration.vi"() -> ("output_laser1_pulse_duration"=w1386:i32)  [unwired: 11 in]
              n718 = Replace Array Subset(array=w1408, new element #1=w1406, index #1=w1407, new element #2=w1404, index #2=w1405, new element #3=w1400, index #3=w1402, new element #4=w1399, index #4=w1401, new element #5=w1381, index #5=w1385, new element #6=w1376, index #6=w1380, new element #7=w1371, index #7=w1375, new element #8=w1366, index #8=w1370, new element #9=w1361, index #9=w1365, new element #10=w1349, index #10=w1358, new element #11=w1348, index #11=w1357, new element #12=w1359, index #12=w1360) -> (w1403:u16[])
              n719 = Replace Array Subset(array=w1388, new element=w1359, index=w1386) -> (w1387:u16[])
            }
            frame 6 {
              # "Selection First"
              # "Count"
              # "Tdelay"
              # "Probability"
              # "OnOff"
              # "Block"
              # "delayOpt"
              # "Count"
              # "Tdelay"
              # "Probability"
              # "OnOff"
              # "Block"
              # "ENL1 All"
              # "delayOpt"
              # "Count"
              # "Tdelay"
              # "Probability"
              # "OnOff"
              # "Block"
              # "ENL1 First"
              n720 = call "myRIO_BRig_RT_dataLC_ENL1_All_Block.vi"() -> ("output_ENL1_All_Block"=w1443:i32)  [unwired: 11 in]
              n721 = call "myRIO_BRig_RT_dataLC_ENL1_All_OnOff.vi"() -> ("output_ENL1_All_OnOff"=w1433:i32)  [unwired: 11 in]
              n722 = call "myRIO_BRig_RT_dataLC_ENL1_All_Probability.vi"() -> ("output_ENL1_All_Probability"=w1432:i32)  [unwired: 11 in]
              n723 = call "myRIO_BRig_RT_dataLC_ENL1_All_Tdelay.vi"() -> ("output_ENL1_All_Tdelay"=w1431:i32)  [unwired: 11 in]
              n724 = call "myRIO_BRig_RT_dataLC_ENL1_All_Count.vi"() -> ("output_ENL1_All_Count"=w1430:i32)  [unwired: 11 in]
              n725 = call "myRIO_BRig_RT_dataLC_ENL1_All_delayOpt.vi"() -> ("output_ENL1_All_delayOpt"=w1429:i32)  [unwired: 11 in]
              n726 = call "myRIO_BRig_RT_dataLC_ENL1_First_Block.vi"() -> ("output_ENL1_First_Block"=w1469:i32)  [unwired: 11 in]
              n727 = call "myRIO_BRig_RT_dataLC_ENL1_First_OnOff.vi"() -> ("output_ENL1_First_OnOff"=w1467:i32)  [unwired: 11 in]
              n728 = call "myRIO_BRig_RT_dataLC_ENL1_First_Probability.vi"() -> ("output_ENL1_First_Probability"=w1463:i32)  [unwired: 11 in]
              n729 = call "myRIO_BRig_RT_dataLC_ENL1_First_Tdelay.vi"() -> ("output_ENL1_First_Tdelay"=w1461:i32)  [unwired: 11 in]
              n730 = call "myRIO_BRig_RT_dataLC_ENL1_First_Count.vi"() -> ("output_ENL1_First_Count"=w1459:i32)  [unwired: 11 in]
              n731 = call "myRIO_BRig_RT_dataLC_ENL1_First_delayOpt.vi"() -> ("output_ENL1_First_delayOpt"=w1445:i32)  [unwired: 11 in]
              n732 = local read "LC_ENL1_First_delayOpt"() -> (w1446:bool)
              n733 = local read "LC_ENL1_First_Count"() -> (w1458:u16)
              n734 = call "myRIO_BRig_RT_dataLC_Selection_First_Block.vi"() -> ("output_Selection_First_Block"=w1427:i32)  [unwired: 11 in]
              n735 = call "myRIO_BRig_RT_dataLC_Selection_First_OnOff.vi"() -> ("output_Selection_First_OnOff"=w1426:i32)  [unwired: 11 in]
              n736 = call "myRIO_BRig_RT_dataLC_Selection_First_Probability.vi"() -> ("output_Selection_First_Probability"=w1425:i32)  [unwired: 11 in]
              n737 = call "myRIO_BRig_RT_dataLC_Selection_First_Tdelay.vi"() -> ("output_Selection_First_Tdelay"=w1424:i32)  [unwired: 11 in]
              n738 = call "myRIO_BRig_RT_dataLC_Selection_First_Count.vi"() -> ("output_Selection_First_Count"=w1423:i32)  [unwired: 11 in]
              n739 = local read "LC_ENL1_First_Probability"() -> (w1462:u16)
              n740 = local read "LC_ENL1_First_Block"() -> (w1468:u16)
              n741 = local read "LC_ENL1_First_Tdelay"() -> (w1460:u16)
              n742 = local read "LC_ENL1_First_OnOff"() -> (w1466:bool)
              n743 = local read "LC_ENL1_All_OnOff"() -> (w1439:bool)
              n744 = local read "LC_ENL1_All_Probability"() -> (w1437:u16)
              n745 = local read "LC_ENL1_All_delayOpt"() -> (w1435:bool)
              n746 = local read "LC_ENL1_All_Tdelay"() -> (w1428:u16)
              n747 = local read "LC_ENL1_All_Block"() -> (w1440:u16)
              n748 = local read "LC_ENL1_All_Count"() -> (w1436:u16)
              n749 = local read "LC_Sel_First_Probability"() -> (w1418:u16)
              n750 = local read "LC_Sel_First_Tdelay"() -> (w1417:u16)
              n751 = local read "LC_Sel_First_OnOff"() -> (w1421:bool)
              n752 = local read "LC_Sel_First_Count"() -> (w1416:u16)
              n753 = local read "LC_Sel_First_Block"() -> (w1420:u16)
              n754 = Boolean To (0,1)(Boolean=w1446) -> (0, 1=w1447:i16)
              n755 = Boolean To (0,1)(Boolean=w1466) -> (0, 1=w1465:i16)
              n756 = Boolean To (0,1)(Boolean=w1439) -> (0, 1=w1442:i16)
              n757 = To Unsigned Word Integer(number=w1447) -> (unsigned 16bit integer=w1444:u16)
              n758 = To Unsigned Word Integer(number=w1465) -> (unsigned 16bit integer=w1464:u16)
              n759 = Boolean To (0,1)(Boolean=w1435) -> (0, 1=w1441:i16)
              n760 = To Unsigned Word Integer(number=w1442) -> (unsigned 16bit integer=w1438:u16)
              n761 = Boolean To (0,1)(Boolean=w1421) -> (0, 1=w1422:i16)
              n762 = To Unsigned Word Integer(number=w1441) -> (unsigned 16bit integer=w1434:u16)
              n763 = To Unsigned Word Integer(number=w1422) -> (unsigned 16bit integer=w1419:u16)
              n764 = Replace Array Subset(array=w1470, new element #1=w1468, index #1=w1469, new element #2=w1464, index #2=w1467, new element #3=w1462, index #3=w1463, new element #4=w1460, index #4=w1461, new element #5=w1458, index #5=w1459, new element #6=w1444, index #6=w1445, new element #7=w1440, index #7=w1443, new element #8=w1438, index #8=w1433, new element #9=w1437, index #9=w1432, new element #10=w1428, index #10=w1431, new element #11=w1436, index #11=w1430, new element #12=w1434, index #12=w1429, new element #13=w1420, index #13=w1427, new element #14=w1419, index #14=w1426, new element #15=w1418, index #15=w1425, new element #16=w1417, index #16=w1424, new element #17=w1416, index #17=w1423) -> (w1471:u16[])
            }
            frame 7 {
              # "Selection All"
              # "Count"
              # "Tdelay"
              # "Probability"
              # "OnOff"
              # "Block"
              # "delayOpt"
              # "Count"
              # "Tdelay"
              # "Probability"
              # "OnOff"
              # "Block"
              # "Cue1 All"
              # "delayOpt"
              # "Count"
              # "Tdelay"
              # "Probability"
              # "OnOff"
              # "Block"
              # "Cue1 First"
              n765 = call "myRIO_BRig_RT_dataLC_Cue1_First_delayOpt.vi"() -> ("output_Cue1_First_delayOpt"=w1510:i32)  [unwired: 11 in]
              n766 = call "myRIO_BRig_RT_dataLC_Cue1_First_Block.vi"() -> ("output_Cue1_First_Block"=w1533:i32)  [unwired: 11 in]
              n767 = call "myRIO_BRig_RT_dataLC_Cue1_First_OnOff.vi"() -> ("output_Cue1_First_OnOff"=w1531:i32)  [unwired: 11 in]
              n768 = call "myRIO_BRig_RT_dataLC_Cue1_First_Probability.vi"() -> ("output_Cue1_First_Probability"=w1527:i32)  [unwired: 11 in]
              n769 = call "myRIO_BRig_RT_dataLC_Cue1_First_Tdelay.vi"() -> ("output_Cue1_First_Tdelay"=w1525:i32)  [unwired: 11 in]
              n770 = call "myRIO_BRig_RT_dataLC_Cue1_First_Count.vi"() -> ("output_Cue1_First_Count"=w1523:i32)  [unwired: 11 in]
              n771 = call "myRIO_BRig_RT_dataLC_Cue1_l1_All_Block.vi"() -> ("output_Cue1_l1_All_Block"=w1507:i32)  [unwired: 11 in]
              n772 = call "myRIO_BRig_RT_dataLC_Cue1_All_OnOff.vi"() -> ("output_Cue1_All_OnOff"=w1506:i32)  [unwired: 11 in]
              n773 = call "myRIO_BRig_RT_dataLC_Cue1_All_Probability.vi"() -> ("output_Cue1_All_Probability"=w1505:i32)  [unwired: 11 in]
              n774 = call "myRIO_BRig_RT_dataLC_Cue1_All_Tdelay.vi"() -> ("output_Cue1_All_Tdelay"=w1504:i32)  [unwired: 11 in]
              n775 = call "myRIO_BRig_RT_dataLC_Cue1_l1_All_Count.vi"() -> ("output_Cue1_All_Count"=w1503:i32)  [unwired: 11 in]
              n776 = call "myRIO_BRig_RT_dataLC_Cue1_All_delayOpt.vi"() -> ("output_Cue1_All_delayOpt"=w1502:i32)  [unwired: 11 in]
              n777 = local read "LC_Cue1_First_delayOpt"() -> (w1509:bool)
              n778 = local read "LC_Cue1_First_Count"() -> (w1522:u16)
              n779 = local read "LC_Cue1_First_Probability"() -> (w1526:u16)
              n780 = local read "LC_Cue1_First_Block"() -> (w1532:u16)
              n781 = local read "LC_Cue1_First_Tdelay"() -> (w1524:u16)
              n782 = local read "LC_Cue1_First_OnOff"() -> (w1530:bool)
              n783 = call "myRIO_BRig_RT_dataLC_Selection_All_Block.vi"() -> ("output_Selection_All_Block"=w1491:i32)  [unwired: 11 in]
              n784 = call "myRIO_BRig_RT_dataLC_Selection_All_OnOff.vi"() -> ("output_Selection_All_OnOff"=w1490:i32)  [unwired: 11 in]
              n785 = call "myRIO_BRig_RT_dataLC_Selection_All_Probability.vi"() -> ("output_Selection_All_Probability"=w1489:i32)  [unwired: 11 in]
              n786 = call "myRIO_BRig_RT_dataLC_Selection_All_Tdelay.vi"() -> ("output_Selection_All_Tdelay"=w1488:i32)  [unwired: 11 in]
              n787 = call "myRIO_BRig_RT_dataLC_Selection_All_Count.vi"() -> ("output_Selection_All_Count"=w1481:i32)  [unwired: 11 in]
              n788 = local read "LC_Cue1_All_OnOff"() -> (w1498:bool)
              n789 = local read "LC_Cue1_All_delayOpt"() -> (w1499:bool)
              n790 = local read "LC_Cue1_All_Probability"() -> (w1495:u16)
              n791 = local read "LC_Cue1_All_Tdelay"() -> (w1494:u16)
              n792 = local read "LC_Cue1_All_Count"() -> (w1493:u16)
              n793 = local read "LC_Cue1_All_Block"() -> (w1497:u16)
              n794 = local read "LC_Sel_All_Probability"() -> (w1483:u16)
              n795 = local read "LC_Sel_All_Tdelay"() -> (w1482:u16)
              n796 = local read "LC_Sel_All_OnOff"() -> (w1485:bool)
              n797 = local read "LC_Sel_All_Count"() -> (w1480:u16)
              n798 = local read "LC_Sel_All_Block"() -> (w1487:u16)
              n799 = Boolean To (0,1)(Boolean=w1509) -> (0, 1=w1511:i16)
              n800 = Boolean To (0,1)(Boolean=w1530) -> (0, 1=w1529:i16)
              n801 = Boolean To (0,1)(Boolean=w1498) -> (0, 1=w1501:i16)
              n802 = To Unsigned Word Integer(number=w1511) -> (unsigned 16bit integer=w1508:u16)
              n803 = To Unsigned Word Integer(number=w1529) -> (unsigned 16bit integer=w1528:u16)
              n804 = To Unsigned Word Integer(number=w1501) -> (unsigned 16bit integer=w1496:u16)
              n805 = Boolean To (0,1)(Boolean=w1499) -> (0, 1=w1500:i16)
              n806 = Boolean To (0,1)(Boolean=w1485) -> (0, 1=w1486:i16)
              n807 = To Unsigned Word Integer(number=w1500) -> (unsigned 16bit integer=w1492:u16)
              n808 = To Unsigned Word Integer(number=w1486) -> (unsigned 16bit integer=w1484:u16)
              n809 = Replace Array Subset(array=w1534, new element #1=w1532, index #1=w1533, new element #2=w1528, index #2=w1531, new element #3=w1526, index #3=w1527, new element #4=w1524, index #4=w1525, new element #5=w1522, index #5=w1523, new element #6=w1508, index #6=w1510, new element #7=w1497, index #7=w1507, new element #8=w1496, index #8=w1506, new element #9=w1495, index #9=w1505, new element #10=w1494, index #10=w1504, new element #11=w1493, index #11=w1503, new element #12=w1492, index #12=w1502, new element #13=w1487, index #13=w1491, new element #14=w1484, index #14=w1490, new element #15=w1483, index #15=w1489, new element #16=w1482, index #16=w1488, new element #17=w1480, index #17=w1481) -> (w1535:u16[])
            }
            frame 8 {
              # "Trial"
              # "Tdelay"
              # "Probability"
              # "OnOff"
              # "Block"
              # "Wrong"
              # "Trial"
              # "Tdelay"
              # "Probability"
              # "OnOff"
              # "Block"
              # "Reward"
              n810 = call "myRIO_BRig_RT_dataLC_Wrong_Block.vi"() -> ("output_Wrong_Block"=w1565:i32)  [unwired: 11 in]
              n811 = call "myRIO_BRig_RT_dataLC_Wrong_OnOff.vi"() -> ("output_Wrong_OnOff"=w1564:i32)  [unwired: 11 in]
              n812 = call "myRIO_BRig_RT_dataLC_Wrong_Probability.vi"() -> ("output_Wrong_Probability"=w1563:i32)  [unwired: 11 in]
              n813 = call "myRIO_BRig_RT_dataLC_Wrong_Tdelay.vi"() -> ("output_Wrong_Tdelay"=w1562:i32)  [unwired: 11 in]
              n814 = call "myRIO_BRig_RT_dataLC_Wrong_Trial.vi"() -> ("output_Wrong_Trial"=w1561:i32)  [unwired: 11 in]
              n815 = call "myRIO_BRig_RT_dataLC_Reward_Block.vi"() -> ("output_Reward_Block"=w1577:i32)  [unwired: 11 in]
              n816 = call "myRIO_BRig_RT_dataLC_Reward_OnOff.vi"() -> ("output_Reward_OnOff"=w1575:i32)  [unwired: 11 in]
              n817 = call "myRIO_BRig_RT_dataLC_Reward_Probability.vi"() -> ("output_Reward_Probability"=w1571:i32)  [unwired: 11 in]
              n818 = call "myRIO_BRig_RT_dataLC_Reward_Tdelay.vi"() -> ("output_Reward_Tdelay"=w1569:i32)  [unwired: 11 in]
              n819 = call "myRIO_BRig_RT_dataLC_Reward_Trial.vi"() -> ("output_Reward_Trial"=w1567:i32)  [unwired: 11 in]
              n820 = local read "LC_Wrong_OnOff"() -> (w1559:bool)
              n821 = local read "LC_Wrong_Probability"() -> (w1556:u16)
              n822 = local read "LC_Wrong_Block"() -> (w1558:u16)
              n823 = local read "LC_Wrong_Tdelay"() -> (w1555:u16)
              n824 = local read "LC_Wrong_Trial"() -> (w1554:u16)
              n825 = local read "LC_Reward_Probability"() -> (w1570:u16)
              n826 = local read "LC_Reward_Block"() -> (w1576:u16)
              n827 = local read "LC_Reward_Tdelay"() -> (w1568:u16)
              n828 = local read "LC_Reward_OnOff"() -> (w1574:bool)
              n829 = local read "LC_Reward_Trial"() -> (w1566:u16)
              n830 = Boolean To (0,1)(Boolean=w1559) -> (0, 1=w1560:i16)
              n831 = Boolean To (0,1)(Boolean=w1574) -> (0, 1=w1573:i16)
              n832 = To Unsigned Word Integer(number=w1560) -> (unsigned 16bit integer=w1557:u16)
              n833 = To Unsigned Word Integer(number=w1573) -> (unsigned 16bit integer=w1572:u16)
              n834 = Replace Array Subset(array=w1578, new element #1=w1576, index #1=w1577, new element #2=w1572, index #2=w1575, new element #3=w1570, index #3=w1571, new element #4=w1568, index #4=w1569, new element #5=w1566, index #5=w1567, new element #6=w1558, index #6=w1565, new element #7=w1557, index #7=w1564, new element #8=w1556, index #8=w1563, new element #9=w1555, index #9=w1562, new element #10=w1554, index #10=w1561) -> (w1579:u16[])
            }
            frame 12 {
              # "amp_L"
              # "amp_R"
              # "freq_L"
              # "freq_R"
              n835 = call "myRIO_BRig_RT_dataExp_Audio_amp__L.vi"() -> ("output_Audio_amp__L"=w1604:i32)  [unwired: 11 in]
              n836 = call "myRIO_BRig_RT_dataExp_Audio_amp__R.vi"() -> ("output_Audio_amp__R"=w1603:i32)  [unwired: 11 in]
              n837 = call "myRIO_BRig_RT_dataExp_Audio_freq__L.vi"() -> ("output_Audio_freq__L"=w1602:i32)  [unwired: 11 in]
              n838 = call "myRIO_BRig_RT_dataExp_Audio_freq__R.vi"() -> ("output_Audio_freq__R"=w1601:i32)  [unwired: 11 in]
              n839 = Index Array(array=w1600, index #1=w1604, index #2=w1603, index #3=w1602, index #4=w1601) -> (element #1=w1599:u16, element #2=w1598:u16, element #3=w1591:u16, element #4=w1589:u16)
              n840 = To Unsigned Byte Integer(number=w1591) -> (unsigned 8bit integer=w1590:u8)
              n841 = To Unsigned Byte Integer(number=w1589) -> (unsigned 8bit integer=w1588:u8)
            }
            frame 13 {
              (unwired) u32 0 ("tDelay_laser_rew")
              # "Wrong tDelay"
              # "Reward tDelay"
              n842 = call "myRIO_BRig_RT_dataLC_Reward_Tdelay.vi"() -> ("output_Reward_Tdelay"=w1631:i32)  [unwired: 11 in]
              n843 = call "myRIO_BRig_RT_dataLC_Wrong_Tdelay.vi"() -> ("output_Wrong_Tdelay"=w1632:i32)  [unwired: 11 in]
              n844 = Index Array(array=w1628, index #1=w1631, index #2=w1632) -> (element #1=w1630:u16, element #2=w1629:u16)
              n845 = call "myRIO_BRig_RT__calc_Tvalley.vi"("input_peakWidth"="laser_Tpeak", "input_freq"="laser_Freq") -> ("output_Tvalley"=w1638:dbl)  [unwired: 9 in]
              n846 = To Double Precision Float(number=w1630) -> (double precision float=w1625:dbl)
              n847 = To Double Precision Float(number=w1629) -> (double precision float=w1622:dbl)
              n848 = Multiply(x="f_millisec2count", y="laser_Tpeak") -> (x*y=w1647:dbl)
              n849 = Multiply(x="f_millisec2count", y=w1638) -> (x*y=w1644:dbl)
              n850 = Multiply(x="f_millisec2count", y="laser_Tshutter") -> (x*y=w1642:dbl)
              n851 = Round Toward +Infinity(x="laser_Tshutter") -> (ceil(x): smallest int >= x=w1633:dbl)
              n852 = Multiply(x="f_millisec2count", y=w1625) -> (x*y=w1626:dbl)
              n853 = Multiply(x="f_millisec2count", y=w1622) -> (x*y=w1623:dbl)
              n854 = To Unsigned Word Integer(number="f_millisec2count") -> (unsigned 16bit integer=w1613:u16)
              n855 = Round Toward +Infinity(x=w1647) -> (ceil(x): smallest int >= x=w1648:dbl)
              n856 = Round Toward +Infinity(x=w1644) -> (ceil(x): smallest int >= x=w1645:dbl)
              n857 = Round Toward +Infinity(x=w1642) -> (ceil(x): smallest int >= x=w1637:dbl)
              n858 = Round Toward +Infinity(x=w1626) -> (ceil(x): smallest int >= x=w1627:dbl)
              n859 = Round Toward +Infinity(x=w1623) -> (ceil(x): smallest int >= x=w1624:dbl)
              n860 = To Unsigned Long Integer(number=w1648) -> (unsigned 32bit integer=w1646:u32)
              n861 = To Unsigned Long Integer(number=w1645) -> (unsigned 32bit integer=w1643:u32)
              n862 = To Unsigned Long Integer(number=w1637) -> (unsigned 32bit integer=w1641:u32)
              n863 = To Unsigned Word Integer(number=w1633) -> (unsigned 16bit integer=w1636:u16)
              n864 = To Unsigned Long Integer(number=w1627) -> (unsigned 32bit integer=w1621:u32)
              n865 = To Unsigned Long Integer(number=w1624) -> (unsigned 32bit integer=w1620:u32)
              n866 = Add(x="laser_duration", y=w1636) -> (x+y=w1617:u16)
              n867 = To Double Precision Float(number=w1617) -> (double precision float=w1616:dbl)
              n868 = Multiply(x=w1616, y="f_millisec2count") -> (x*y=w1618:dbl)
              n869 = call "myRIO_BRig_RT_dataCurrent_laser1_pulse_duration.vi"() -> ("output_laser1_pulse_duration"=w1649:i32)  [unwired: 11 in]
              n870 = Round Toward +Infinity(x=w1618) -> (ceil(x): smallest int >= x=w1619:dbl)
              n871 = To Unsigned Long Integer(number=w1619) -> (unsigned 32bit integer=w1615:u32)
              n872 = xnode "Read/Write Control"("FPGA VI Reference In"=w1651, "error in"=w1652, "laser_Npeak"=w1646, "laser_Nvalley"=w1643, "laser_Nshutter"=w1641, "laser_selRew_Ndelay"=w1621, "laser_selWro_NDelay"=w1620, "laser_selRew_Ntotal"=w1615, "laser_selWro_Ntotal"=w1615, "k1__counter_per_ms"=w1613) -> ("error out"=→"error out":errorcluster)  [unwired: 1 out]
              n873 = Replace Array Subset(array=w1628, new element=w1617, index=w1649) -> (w1650:u16[])
            }
            frame 15 {
              n874 = call "myRIO_Brig_RT__Case_Exp_State_initBlock.vi"("input_spout"=w1696, "input_dataExp"=w1694, "input_dataCurrent"=w1695) -> ("output_spout"=w1674:enum16{"Left", "Right"}, "output_state"=w1697:T2, "output_dataExp"=w1693:u16[], "output_dataCurrent"=w1679:u16[], "output_TpB_target"=→"TpB_target":u16)  [unwired: 4 in]
              "cSpout" <- w1674
              n875 = call "myRIO_BRig_RT_dataCurrent_iBlock.vi"() -> ("output_iBlock"=w1678:i32)  [unwired: 11 in]
              n876 = Index Array(array=w1679, index=w1678) -> (element=w1672:u16)
              "iBlock" <- w1672
            }
            frame 16 {
              n877 = local write "nRewards_cur"(u16 0 ("nRewards_cur")) -> ()
              n878 = call "myRIO_BRig_RT__Case_Exp_State_initBlock2.vi"("input_spout"=w1705, "input_dataBlock"=w1706, "input_dataCurrent"=w1704) -> ("idxDataBlock"=w1701:i32, "output_dataBlock"=w1703:u16[][])  [unwired: 7 in]
            }
            frame 19 {
              n879 = call "myRIO_Brig_RT__Case_Exp_State_initTrial.vi"("input_spout"=w1724, "input_dataExp"=w1740, "input_dataCurrent"=w1741) -> ("output_state"=w1742:T2, "output_dataExp"=w1739:u16[], "output_dataCurrent"=w1729:u16[])  [unwired: 6 in]
              n880 = call "myRIO_BRig_RT_dataCurrent_iTrial.vi"() -> ("output_iTrial"=w1728:i32)  [unwired: 11 in]
              n881 = call "myRIO_BRig_RT_dataCurrent_SolenoidReward.vi"() -> ("output_SolenoidReward"=w1723:i32)  [unwired: 11 in]
              n882 = Index Array(array=w1729, index #1=w1728, index #2=w1723) -> (element #1=w1719:u16, element #2=w1722:u16)
              "iTrial" <- w1719
              n883 = Not Equal To 0?(x=w1722) -> (x != 0?=→"SolenoidReward":bool)
            }
            frame 20 {
              # "trialUntilReward"
              n884 = call "myRIO_BRig_RT__Case_Exp_subState_LC__initTrial.vi"("input_dataTrial"=w1749, "input_spout"=w1758, "input_dataCurrent"=w1747, "input_dataLC"=w1746) -> ("output_LC_Wrong"=w1759:bool, "output_LC_led_Wrong"=w1751:bool, "output_LC_Reward"=w1760:bool, "output_LC_led_Reward"=w1750:bool, "output_dataTrial"=w1748:u16[][])  [unwired: 2 in]
              n885 = Equal?(x=w1758, y=enum16{"Left", "Right"}."Right") -> (x = y?=w1756:bool)
              n886 = call "myRIO_BRig_RT_dataExp_ItrialUntilReward.vi"() -> ("output_I_trialUntilReward"=w1754:i32)  [unwired: 11 in]
              n887 = Index Array(array=w1755, index=w1754) -> (element=w1753:u16)
              n888 = Not Equal To 0?(x=w1753) -> (x != 0?=w1752:bool)
              n889 = xnode "Read/Write Control"("FPGA VI Reference In"=w1773, "error in"=w1772, "SelectionState"=FALSE, "laserResponse_reward"=w1760, "laserResponse_wrong"=w1759, "laserResponse_reward_LED"=w1750, "laserResponse_wrong_LED"=w1751, "Left(F)_or_Right(T)"=w1756, "ignoreWrong"=w1752) -> ("error out"=→"error_initTrial":errorcluster)  [unwired: 1 out]
            }
            frame 21 {
              n890 = call "myRIO_BRig_RT__Case_Exp_State_initTrial_dataTrial.vi"("input_spout"=w1788, "input_dataCurrent"=w1789, "input_dataExp"=w1787, "input_dataTrial"=w1791) -> ("output_dataTrial"=w1790:u16[][], "output_laserPower"=w1784:u16)  [unwired: 6 in]
              n891 = To Double Precision Float(number=w1784) -> (double precision float=w1786:dbl)
              n892 = Divide(x=w1786, y=100.0 ("x")) -> (x/y=w1780:dbl)
              "output_PortA" <- w1780
              n893 = call "myRIO__convert__Voltage_to_FPGAvalue.vi"("input_voltage"=w1780) -> ("output_PortC"=w1779:i16)  [unwired: 9 in, 1 out]
              n894 = xnode "Read/Write Control"("FPGA VI Reference In"=w1783, "error in"=w1782, "AnaOut_0"=w1779) -> ("error out"=→"error out 4":errorcluster)  [unwired: 1 out]
            }
            frame 22 {
              n895 = call "myRIO_BRig_RT_dataCurrent_idxDataTrial.vi"() -> ("output_idxDataTrial"=w1816:i32)  [unwired: 11 in]
              n896 = call "myRIO_BRig_RT_dataTrial_activeRecording.vi"() -> ("output_activeRecording"=w1813:i32)  [unwired: 11 in]
              n897 = Index Array(array=w1818, index=w1816) -> (element=w1815:u16)
              n898 = Boolean To (0,1)(Boolean="Recording") -> (0, 1=w1812:i16)
              n899 = To Long Integer(number=w1815) -> (32bit integer=w1814:i32)
              n900 = To Unsigned Word Integer(number=w1812) -> (unsigned 16bit integer=w1811:u16)
              n901 = Replace Array Subset(array=w1817, new element=w1811, index (row)=w1814, index (col)=w1813) -> (w1810:u16[][])
            }
            frame 23 {
              n902 = call "myRIO_BRig_RT__Case_Exp_State_initTrial_LC_ENL1__v2.vi"("input_dataTrial"=w1842, "input_spout"=w1847, "input_dataBlock"=w1840, "input_dataLC"=w1848, "input_dataCurrent"=w1844) -> ("output_LC__ENL1"=w1846:bool, "output_LC_led__ENL1"=w1845:bool, "output_dataTrial"=w1841:u16[][], "output_dataCurrent"=w1843:u16[])  [unwired: 3 in]
            }
            frame 24 {
              w1863 = TRUE ("Recording")
              n903 = call "myRIO_BRig_RT__Case_Exp_State_initTrial_LC_Cue1__v2.vi"("input_dataTrial"=w1870, "input_spout"=w1873, "input_dataBlock"=w1868, "input_dataLC"=w1874, "input_dataCurrent"=w1872) -> ("output_LC__Cue1"=w1866:bool, "output_LC_led__Cue1"=w1867:bool, "output_dataTrial"=w1869:u16[][], "output_dataCurrent"=w1871:u16[])  [unwired: 3 in]
            }
            frame 25 {
              n904 = call "myRIO_BRig_RT__Case_Exp_State_initTrial_LC_Sel__v2.vi"("input_dataTrial"=w1899, "input_spout"=w1902, "input_dataBlock"=w1897, "input_dataLC"=w1903, "input_dataCurrent"=w1901) -> ("output_LC__Sel"=w1889:bool, "output_LC_led__Sel"=w1890:bool, "output_dataTrial"=w1898:u16[][], "output_dataCurrent"=w1900:u16[])  [unwired: 3 in]
              n905 = local read "Recording"() -> (w1894:bool)
            }
            frame 27 {
              # "ENL1_n"
              # "Tcycle"
              # "counter"
              n906 = call "myRIO_BRig_RT_dataCurrent_Tcycle_generic.vi"() -> ("output_Tcycle_generic"=w1949:i32)  [unwired: 11 in]
              n907 = call "myRIO_BRig_RT_dataCurrent_count_generic.vi"() -> ("output_count_generic"=w1951:i32)  [unwired: 11 in]
              n908 = call "myRIO_BRig_RT_dataCurrent_ENL.vi"() -> ("output_ENL"=w1948:i32)  [unwired: 11 in]
              n909 = call "myRIO_BRig_RT_dataCurrent_nENL1.vi"() -> ("output_nENL1"=w1922:i32)  [unwired: 11 in]
              n910 = Index Array(array=w1942, index #1=w1948, index #2=w1922) -> (element #1=w1947:u16, element #2=w1921:u16)
              n911 = Increment(x=w1921) -> (x+1=w1920:u16)
              n912 = Replace Array Subset(array=w1942, new element #1=u16 0 ("new element/subarray"), index #1=w1951, new element #2=w1947, index #2=w1949, new element #3=w1920, index #3=w1922) -> (w1946:u16[])
              n913 = Select(t=myRIO_BRig_RT__Case_Exp_stateList."ENL1Penalty_pre" ("Enum"), s=w1930, f=myRIO_BRig_RT__Case_Exp_stateList."ENL1" ("Enum")) -> (s? t:f=w1927:T2)
            }
            frame 28 {
              n914 = call "myRIO_BRig_RT__Case_Exp_State_ENL1__v2.vi"("input_LC"=w1958, "I_lick"=w1961, "input_LC_led"=w1959, "input_state"=w1967, "input_dataCurrent"=w1966) -> ("output_trigger_laser_led"=w1957:bool, "output_state"=w1964:T2, "output_dataCurrent"=w1965:u16[], "output_trigger_laser"=w1956:bool)  [unwired: 3 in]
            }
            frame 30 {
              # "Tcycle"
              # "counter"
              n915 = call "myRIO_BRig_RT_dataCurrent_Tcycle_generic.vi"() -> ("output_Tcycle_generic"=w2007:i32)  [unwired: 11 in]
              n916 = call "myRIO_BRig_RT_dataCurrent_count_generic.vi"() -> ("output_count_generic"=w2009:i32)  [unwired: 11 in]
              n917 = call "myRIO_BRig_RT_dataExp_ENL_penalty.vi"() -> ("output_ENL_penalty"=w2002:i32)  [unwired: 11 in]
              n918 = Index Array(array=w2003, index=w2002) -> (element=w2006:u16)
              n919 = Replace Array Subset(array=w2004, new element #1=u16 0 ("new element/subarray"), index #1=w2009, new element #2=w2006, index #2=w2007) -> (w2005:u16[])
            }
            frame 31 {
              n920 = call "myRIO_BRig_RT__Case_Exp_State_ENL1Penalty.vi"("input_state"=w2032, "input_dataCurrent"=w2036) -> ("output_state"=w2033:T2, "output_dataCurrent"=w2035:u16[])  [unwired: 8 in]
            }
            frame 32 {
            }
            frame 33 {
            }
            frame 34 {
            }
            frame 35 {
            }
            frame 36 {
              # "Cue1_n"
              # "Tcycle_Cue1"
              # "0 = L, 1 = R, 2 = both"
              # "sp_R"
              # "sp_L"
              # "Tcycle"
              # "counter"
              n921 = Equal?(x=w2147, y=enum16{"Left", "Right"}."Left") -> (x = y?=w2146:bool)
              n922 = call "myRIO_BRig_RT_dataExp_Audio_sp__L.vi"() -> ("output_Audio_sp__L"=w2145:i32)  [unwired: 11 in]
              n923 = call "myRIO_BRig_RT_dataExp_Audio_sp__R.vi"() -> ("output_Audio_sp__R"=w2144:i32)  [unwired: 11 in]
              n924 = call "myRIO_BRig_RT_dataCurrent_Tcycle_generic.vi"() -> ("output_Tcycle_generic"=w2157:i32)  [unwired: 11 in]
              n925 = call "myRIO_BRig_RT_dataCurrent_count_generic.vi"() -> ("output_count_generic"=w2159:i32)  [unwired: 11 in]
              n926 = Select(t=w2145, s=w2146, f=w2144) -> (s? t:f=w2143:i32)
              n927 = call "myRIO_BRig_RT_dataCurrent_nCue1.vi"() -> ("output_nCue1"=w2121:i32)  [unwired: 11 in]
              n928 = call "myRIO_BRig_RT_dataCurrent_Tcycle_cue.vi"() -> ("output_Tcycle_cue"=w2130:i32)  [unwired: 11 in]
              n929 = Index Array(array=w2149, index=w2143) -> (element=w2141:u16)
              n930 = Index Array(array=w2131, index #1=w2130, index #2=w2121) -> (element #1=w2132:u16, element #2=w2123:u16)
              n931 = Increment(x=w2123) -> (x+1=w2122:u16)
              n932 = Not Equal To 0?(x=w2141) -> (x != 0?=w2139:bool)
              n933 = Not Equal?(x=w2141, y=u16 1) -> (x != y?=w2140:bool)
              n934 = Replace Array Subset(array=w2131, new element #1=u16 0 ("new element/subarray"), index #1=w2159, new element #2=w2132, index #2=w2157, new element #3=w2122, index #3=w2121) -> (w2156:u16[])
              n935 = Select(t=myRIO_BRig_RT__Case_Exp_stateList."Cue1Penalty_pre" ("Enum"), s=w2127, f=myRIO_BRig_RT__Case_Exp_stateList."Cue1" ("Enum")) -> (s? t:f=w2128:T2)
            }
            frame 37 {
              n936 = call "myRIO_BRig_RT__Case_Exp_State_Cue1__v2.vi"("input_LC"=w2168, "I_lick"=w2171, "input_LC_led"=w2169, "input_state"=w2173, "input_dataCurrent"=w2191) -> ("output_trigger_laser_led"=w2166:bool, "output_state"=w2172:T2, "output_dataCurrent"=w2190:u16[], "output_trigger_laser"=w2167:bool)  [unwired: 3 in]
              n937 = Equal?(x=myRIO_BRig_RT__Case_Exp_stateList."Selection_pre", y=w2172) -> (x = y?=w2176:bool)
              n938 = xnode "Read/Write Control"("FPGA VI Reference In"=w2175, "error in"=w2174, "SelectionState"=w2176) -> ()  [unwired: 2 out]
            }
            frame 39 {
              # "Tcycle"
              # "counter"
              n939 = call "myRIO_BRig_RT_dataCurrent_Tcycle_generic.vi"() -> ("output_Tcycle_generic"=w2222:i32)  [unwired: 11 in]
              n940 = call "myRIO_BRig_RT_dataCurrent_count_generic.vi"() -> ("output_count_generic"=w2224:i32)  [unwired: 11 in]
              n941 = call "myRIO_BRig_RT_dataExp_Tcycle_CuePenalty.vi"() -> ("output_Tcycle_CuePenalty"=w2221:i32)  [unwired: 11 in]
              n942 = Index Array(array=w2216, index=w2221) -> (element=w2220:u16)
              n943 = Replace Array Subset(array=w2218, new element #1=u16 0 ("new element/subarray"), index #1=w2224, new element #2=w2220, index #2=w2222) -> (w2217:u16[])
            }
            frame 40 {
              # "reset laserOccurred"
              n944 = call "myRIO_BRig_RT__Case_Exp_State_Cue1Penalty.vi"("input_state"=w2250, "input_dataCurrent"=w2251) -> ("output_state"=w2248:T2, "output_dataCurrent"=w2249:u16[])  [unwired: 8 in]
            }
            frame 41 {
              n945 = call "myRIO_BRig_RT__Case_Exp_subState_LC__Cue2.vi"("input_spout"=w2268, "input_dataCurrent"=w2269, "input_dataLC"=w2267) -> ()  [unwired: 6 in, 2 out]
            }
            frame 42 {
            }
            frame 43 {
            }
            frame 44 {
            }
            frame 45 {
              # "Tcycle"
              # "counter"
              n946 = call "myRIO_BRig_RT_dataCurrent_laser1_tSel_start.vi"() -> ("output_laser1_tSel_start"=w2339:i32)  [unwired: 11 in]
              n947 = xnode "Read/Write Control"("FPGA VI Reference In"=w2349, "error in"=w2350) -> ("error out"=→"error_Selection_pre":errorcluster, "SelectReward"=w2343:bool, "SelectWrong"=w2344:bool)  [unwired: 1 out]
              n948 = call "myRIO_BRig_RT_dataExp_Tcycle_Selection.vi"() -> ("output_Tcycle_Selection"=w2369:i32)  [unwired: 11 in]
              n949 = call "myRIO_BRig_RT_dataCurrent_Tcycle_generic.vi"() -> ("output_Tcycle_generic"=w2370:i32)  [unwired: 11 in]
              n950 = call "myRIO_BRig_RT_dataCurrent_count_generic.vi"() -> ("output_count_generic"=w2372:i32)  [unwired: 11 in]
              n951 = Index Array(array=w2340, index=w2339) -> (element=w2338:u16)
              n952 = Index Array(array=w2366, index=w2369) -> (element=w2368:u16)
              n953 = Equal To 0?(x=w2338) -> (x = 0?=w2336:bool)
              n954 = Replace Array Subset(array=w2340, new element #1=u16 0 ("new element/subarray"), index #1=w2372, new element #2=w2368, index #2=w2370) -> (w2367:u16[])
              n955 = Or(x=w2343, y=w2344) -> (x .or. y?=w2334:bool)
              n956 = Not(x=w2334) -> (.not. x?=w2337:bool)
              n957 = Compound Arithmetic op=AND(w2337, w2336, w2335) -> (w2332:bool)
              n958 = And(x=w2332, y=w2333) -> (x .and. y?=w2331:bool)
              n959 = Select(t=myRIO_BRig_RT__Case_Exp_stateList."SelectReward_pre" ("Enum"), s=w2343, f=myRIO_BRig_RT__Case_Exp_stateList."SelectWrong_pre" ("Enum")) -> (s? t:f=w2348:T2)
              n960 = Select(t=w2348, s=w2334, f=myRIO_BRig_RT__Case_Exp_stateList."Selection" ("Enum")) -> (s? t:f=w2345:T2)
            }
            frame 46 {
              # "counter\nSelection"
              # "increment"
              # "get Tcycle"
              # "get count"
              n961 = call "myRIO_BRig_RT_dataCurrent_Tcycle_generic.vi"() -> ("output_Tcycle_generic"=w2406:i32)  [unwired: 11 in]
              n962 = call "myRIO_BRig_RT_dataCurrent_count_generic.vi"() -> ("output_count_generic"=w2402:i32)  [unwired: 11 in]
              n963 = call "myRIO_BRig_RT_dataCurrent_laser1_tSel_start.vi"() -> ("output_laser1_tSel_start"=w2394:i32)  [unwired: 11 in]
              n964 = call "myRIO_BRig_RT_dataCurrent_laser1_tSel_end.vi"() -> ("output_laser1_tSel_end"=w2393:i32)  [unwired: 11 in]
              n965 = call "myRIO_BRig_RT__increment_u16.vi"() -> ("output_increment__u16"=w2380:u16)  [unwired: 11 in]
              n966 = xnode "Read/Write Control"("FPGA VI Reference In"=w2413, "error in"=w2412) -> ("error out"=→"error_Selection":errorcluster, "SelectReward"=w2409:bool, "SelectWrong"=w2410:bool)  [unwired: 1 out]
              n967 = call "myRIO_BRig_RT_dataCurrent_laser1_triggered_Sel.vi"() -> ("output_laser1_triggered_Selection"=w2381:i32)  [unwired: 11 in]
              n968 = Index Array(array=w2407, index #1=w2406, index #2=w2402, index #3=w2394, index #4=w2393, index #5=w2381) -> (element #1=w2401:u16, element #2=w2379:u16, element #3=w2378:u16, element #4=w2384:u16, element #5=w2375:u16)
              n969 = Increment(x=w2375) -> (x+1=w2376:u16)
              n970 = Equal?(x=w2379, y=w2378) -> (x = y?=w2377:bool)
              n971 = Add(x=w2379, y=w2380) -> (x+y=w2385:u16)
              n972 = Greater Or Equal?(x=w2385, y=w2378) -> (x >= y?=w2382:bool)
              n973 = Less Or Equal?(x=w2385, y=w2384) -> (x <= y?=w2383:bool)
              n974 = Greater?(x=w2401, y=w2385) -> (0:w2387:bool)
              n975 = Select(t=w2376, s=w2377, f=w2375) -> (s? t:f=w2374:u16)
              n976 = Select(t=myRIO_BRig_RT__Case_Exp_stateList."SelectReward_pre" ("Enum"), s=w2409, f=myRIO_BRig_RT__Case_Exp_stateList."SelectWrong_pre" ("Enum")) -> (s? t:f=w2408:T2)
              n977 = Or(x=w2409, y=w2410) -> (x .or. y?=w2388:bool)
              n978 = Not(x=w2388) -> (.not. x?=w2389:bool)
              n979 = Select(t=w2405, s=w2387, f=myRIO_BRig_RT__Case_Exp_stateList."SelectTimeout_pre" ("Enum")) -> (s? t:f=w2396:u16)
              n980 = Compound Arithmetic op=AND(w2387, w2389, w2382, w2383, w2386) -> (w2391:bool)
              n981 = Select(t=w2385, s=w2387, f=w2401) -> (s? t:f=w2399:u16)
              n982 = Select(t=w2408, s=w2388, f=w2396) -> (s? t:f=w2411:u16)
              n983 = And(x=w2391, y=w2390) -> (x .and. y?=w2392:bool)
              n984 = call "myRIO_BRig_RT_dataCurrent_count_selection.vi"() -> ("output_count_generic"=w2400:i32)  [unwired: 11 in]
              n985 = Replace Array Subset(array=w2407, new element #1=w2399, index #1=w2402, new element #2=w2399, index #2=w2400, new element #3=w2374, index #3=w2381) -> (w2404:u16[])
            }
            frame 48 {
              # "iState"
              # "Tcycle\nReward"
              # "nRewTrials"
              # "Tcycle\nGeneric"
              # "counter"
              n986 = call "myRIO_BRig_RT_dataCurrent_nRewTrials.vi"() -> ("output_nRewTrials"=w2445:i32)  [unwired: 11 in]
              n987 = Equal?(x=w2454, y=enum16{"Left", "Right"}."Left") -> (x = y?=w2455:bool)
              n988 = Index Array(array=w2446, index=w2445) -> (element=w2444:u16)
              n989 = call "myRIO_BRig_RT_dataExp_Tcycle_Reward__L.vi"() -> ("output_Tcycle_Reward__L"=w2458:i32)  [unwired: 11 in]
              n990 = call "myRIO_BRig_RT_dataExp_Tcycle_Reward__R.vi"() -> ("output_Tcycle_Reward__R"=w2459:i32)  [unwired: 11 in]
              n991 = Increment(x=w2444) -> (x+1=w2443:u16)
              n992 = Select(t=w2458, s=w2455, f=w2459) -> (s? t:f=w2457:i32)
              n993 = call "myRIO_BRig_RT__Case_Exp_subState_LC__Reward.vi"("input_spout"=w2454, "input_dataCurrent"=w2446, "input_dataLC"=w2453) -> ()  [unwired: 6 in, 2 out]
              n994 = call "myRIO_BRig_RT_dataCurrent_count_generic.vi"() -> ("output_count_generic"=w2448:i32)  [unwired: 11 in]
              n995 = call "myRIO_BRig_RT_dataCurrent_Tcycle_generic.vi"() -> ("output_Tcycle_generic"=w2449:i32)  [unwired: 11 in]
              n996 = Index Array(array=w2460, index=w2457) -> (element=w2450:u16)
              n997 = call "myRIO_BRig_RT_dataCurrent_iState.vi"() -> ("output_iState"=w2438:i32)  [unwired: 11 in]
              n998 = Replace Array Subset(array=w2446, new element #1=w2443, index #1=w2445, new element #2=u16 0 ("new element/subarray"), index #2=w2448, new element #3=w2450, index #3=w2449, new element #4=u16 1 ("new element/subarray"), index #4=w2438) -> (w2461:u16[])
            }
            frame 49 {
              n999 = call "myRIO_BRig_RT__Case_Exp_State_Reward.vi"("input_dataCurrent"=w2482, "input_state"=w2479, "input_spout"=w2477) -> ("output_dataCurrent"=w2481:u16[], "output_state"=w2480:T2, "output__L"=w2475:bool, "output__R"=w2476:bool)  [unwired: 9 in]
            }
            frame 50 {
              # "nRewards"
              # "nRewTrials"
              # "Tcycle"
              # "counter"
              n1000 = call "myRIO_BRig_RT_dataBlock_nRewards__L.vi"() -> ("output_nRewards__L"=w2498:i32)  [unwired: 11 in]
              n1001 = call "myRIO_BRig_RT_dataBlock_nRewards__R.vi"() -> ("output_nRewards__R"=w2497:i32)  [unwired: 11 in]
              n1002 = call "myRIO_BRig_RT_dataCurrent_Tcycle_generic.vi"() -> ("output_Tcycle_generic"=w2517:i32)  [unwired: 11 in]
              n1003 = call "myRIO_BRig_RT_dataCurrent_count_generic.vi"() -> ("output_count_generic"=w2519:i32)  [unwired: 11 in]
              n1004 = case shown="\"Left\", Default" w2491 {
                tunnel: w2503 -> [w2524 w2528]
                tunnel: [w2523 w2528] -> w2502
                tunnel: [w2525 w2526] -> w2501
                tunnel: w2500 -> [w2525 w2527]
                frame "Left", Default {
                  n1005 = Increment(x=w2524) -> (x+1=w2523:u16)
                }
                frame "Right" {
                  n1006 = Increment(x=w2527) -> (x+1=w2526:u16)
                }
              }
              "nRewards_Left" <- w2502
              "nRewards_Right" <- w2501
              n1007 = Equal?(x=w2491, y=enum16{"Left", "Right"}."Left") -> (x = y?=w2490:bool)
              n1008 = Select(t=w2498, s=w2490, f=w2497) -> (s? t:f=w2496:i32)
              n1009 = call "myRIO_BRig_RT_dataExp_Tcycle_RewardPost.vi"() -> ("output_Tcycle_RewardPost"=w2513:i32)  [unwired: 11 in]
              n1010 = call "myRIO_BRig_RT_dataCurrent_nRewTrials.vi"() -> ("output_nRewTrials"=w2499:i32)  [unwired: 11 in]
              n1011 = Index Array(array=w2514, index=w2513) -> (element=w2516:u16)
              n1012 = Index Array(array=w2493, index=w2499) -> (element=w2488:u16)
              n1013 = Replace Array Subset(array=w2493, new element #1=u16 0 ("new element/subarray"), index #1=w2519, new element #2=w2516, index #2=w2517) -> (w2515:u16[])
              n1014 = Replace Array Subset(array=w2495, new element=w2488, index (row)=w2489, index (col)=w2496) -> (w2494:u16[][])
              n1015 = local write "nRewards_cur"(w2488) -> ()
            }
            frame 51 {
              n1016 = call "myRIO_BRig_RT__Case_Exp_State_RewardPost.vi"("input_state"=w2543, "input_dataCurrent"=w2546) -> ("output_state"=w2544:T2, "output_dataCurrent"=w2545:u16[])  [unwired: 8 in]
            }
            frame 52 {
              # "iState"
              # "Tcycle"
              # "counter"
              n1017 = call "myRIO_BRig_RT_dataCurrent_Tcycle_generic.vi"() -> ("output_Tcycle_generic"=w2571:i32)  [unwired: 11 in]
              n1018 = call "myRIO_BRig_RT_dataCurrent_count_generic.vi"() -> ("output_count_generic"=w2573:i32)  [unwired: 11 in]
              n1019 = call "myRIO_BRig_RT_dataExp_Tcycle_Wrong.vi"() -> ("output_Tcycle_Wrong"=w2569:i32)  [unwired: 11 in]
              n1020 = call "myRIO_BRig_RT__Case_Exp_subState_LC__Wrong.vi"("input_spout"=w2565, "input_dataCurrent"=w2566, "input_dataLC"=w2563) -> ()  [unwired: 6 in, 2 out]
              n1021 = Index Array(array=w2567, index=w2569) -> (element=w2570:u16)
              n1022 = call "myRIO_BRig_RT_dataCurrent_iState.vi"() -> ("output_iState"=w2557:i32)  [unwired: 11 in]
              n1023 = Replace Array Subset(array=w2566, new element #1=u16 0 ("new element/subarray"), index #1=w2573, new element #2=w2570, index #2=w2571, new element #3=u16 2 ("new element/subarray"), index #3=w2557) -> (w2568:u16[])
            }
            frame 53 {
              n1024 = call "myRIO_BRig_RT__Case_Exp_State_Wrong.vi"("input_state"=w2587, "input_dataCurrent"=w2596) -> ("output_state"=w2584:T2, "output_dataCurrent"=w2595:u16[])  [unwired: 8 in]
              n1025 = Not Equal?(x=w2587, y=w2584) -> (x != y?=w2586:bool)
              n1026 = Select(t=myRIO_BRig_RT__Case_Exp_stateList."SelectWrong_post" ("Enum"), s=w2586, f=w2584) -> (s? t:f=w2583:T2)
            }
            frame 54 {
            }
            frame 55 {
              # "iState"
              # "Tcycle"
              # "counter"
              n1027 = xnode "Read/Write Control"("FPGA VI Reference In"=w2623, "error in"=w2622, "SelectionState"=FALSE) -> ("error out"=→"error out 3":errorcluster)  [unwired: 1 out]
              n1028 = call "myRIO_BRig_RT_dataCurrent_Tcycle_generic.vi"() -> ("output_Tcycle_generic"=w2645:i32)  [unwired: 11 in]
              n1029 = call "myRIO_BRig_RT_dataCurrent_count_generic.vi"() -> ("output_count_generic"=w2643:i32)  [unwired: 11 in]
              n1030 = call "myRIO_BRig_RT_dataExp_Tcycle_Timeout.vi"() -> ("output_Tcycle_Timeout"=w2647:i32)  [unwired: 11 in]
              n1031 = call "myRIO_BRig_RT__Case_Exp_subState_LC__Timeout.vi"("input_spout"=w2638, "input_dataCurrent"=w2639, "input_dataLC"=w2637) -> ()  [unwired: 6 in, 2 out]
              n1032 = Index Array(array=w2641, index=w2647) -> (element=w2646:u16)
              n1033 = call "myRIO_BRig_RT_dataCurrent_iState.vi"() -> ("output_iState"=w2631:i32)  [unwired: 11 in]
              n1034 = Replace Array Subset(array=w2639, new element #1=u16 0 ("new element/subarray"), index #1=w2643, new element #2=w2646, index #2=w2645, new element #3=u16 3 ("new element/subarray"), index #3=w2631) -> (w2642:u16[])
            }
            frame 56 {
              n1035 = call "myRIO_BRig_RT__Case_Exp_State_Timeout.vi"("input_dataLC"=w2666, "input_state"=w2657, "input_dataCurrent"=w2671) -> ("output_state"=w2658:T2, "output_dataCurrent"=w2670:u16[])  [unwired: 6 in, 1 out]
              n1036 = Not Equal?(x=w2657, y=w2658) -> (x != y?=w2661:bool)
              n1037 = Select(t=myRIO_BRig_RT__Case_Exp_stateList."SelectTimeout_post" ("Enum"), s=w2661, f=w2658) -> (s? t:f=w2659:T2)
            }
            frame 57 {
            }
            frame 59 {
              # "Update dataBlock"
              n1038 = call "myRIO_BRig_RT__Case_Exp_State_endTrial1.vi"("input_spout"=w2704, "input_dataBlock"=w2703, "input_dataCurrent"=w2701) -> ("output_dataBlock"=w2702:u16[][], "output_dataCurrent"=w2700:u16[])  [unwired: 7 in]
            }
            frame 60 {
              # "update dataTrial"
              n1039 = call "myRIO_BRig_RT__Case_Exp_State_endTrial2.vi"("input_spout"=w2723, "input_dataTrial"=w2727, "input_dataCurrent"=w2725) -> ("output_dataTrial"=w2726:u16[][], "output_dataCurrent"=w2724:u16[])  [unwired: 7 in]
            }
            frame 61 {
              # "nRewTrials"
              # "iTrial"
              # "I_blockUntilReward"
              # "TPB"
              # "end block?"
              n1040 = local read "STOP_endTrial"() -> (w2753:bool)
              n1041 = local read "STOP_abort"() -> (w2752:bool)
              n1042 = xnode "Read/Write Control"("FPGA VI Reference In"=w2743, "error in"=w2742, "SelectionState"=FALSE) -> ("error out"=→"error out 2":errorcluster)  [unwired: 1 out]
              n1043 = local read "START"() -> (w2750:bool)
              n1044 = call "myRIO_BRig_RT_dataExp_IblockUntilReward.vi"() -> ("output_I_blockUntilReward"=w2760:i32)  [unwired: 11 in]
              n1045 = Index Array(array=w2746, index=w2760) -> (element=w2744:u16)
              n1046 = Not(x=w2750) -> (.not. x?=w2751:bool)
              n1047 = Not Equal To 0?(x=w2744) -> (x != 0?=w2758:bool)
              n1048 = Compound Arithmetic op=OR(w2753, w2751, w2752) -> (w2738:bool)
              n1049 = call "myRIO_BRig_RT_dataCurrent_nRewTrials.vi"() -> ("output_nRewTrials"=w2756:i32)  [unwired: 11 in]
              n1050 = call "myRIO_BRig_RT_dataCurrent_iTrial.vi"() -> ("output_iTrial"=w2757:i32)  [unwired: 11 in]
              n1051 = Select(t=w2756, s=w2758, f=w2757) -> (s? t:f=w2755:i32)
              n1052 = call "myRIO_BRig_RT_dataCurrent_TpB.vi"() -> ("output_TpB"=w2759:i32)  [unwired: 11 in]
              n1053 = Index Array(array=w2747, index #1=w2759, index #2=w2755) -> (element #1=w2748:u16, element #2=w2749:u16)
              n1054 = Less Or Equal?(x=w2748, y=w2749) -> (x <= y?=w2739:bool)
              n1055 = Or(x=w2738, y=w2739) -> (x .or. y?=w2736:bool)
              n1056 = Select(t=myRIO_BRig_RT__Case_Exp_stateList."saveData_dataBlock" ("Enum"), s=w2736, f=myRIO_BRig_RT__Case_Exp_stateList."dummyState" ("Enum")) -> (s? t:f=w2745:T2)
            }
            frame 64 {
              # "R"
              # "L"
              # "idxDataBlock"
              n1057 = Equal?(x=w2784, y=enum16{"Left", "Right"}."Left") -> (x = y?=w2783:bool)
              n1058 = call "myRIO_BRig_RT_dataCurrent_idxDataBlockL.vi"() -> ("output_idxDataBlock__L"=w2787:i32)  [unwired: 11 in]
              n1059 = call "myRIO_BRig_RT_dataCurrent_idxDataBlockR.vi"() -> ("output_idxDataBlock__R"=w2786:i32)  [unwired: 11 in]
              n1060 = Increment(x=w2778) -> (x+1=w2777:i32)
              n1061 = local read "START"() -> (w2807:bool)
              n1062 = local read "STOP_endBlock"() -> (w2802:bool)
              n1063 = local read "STOP_endTrial"() -> (w2805:bool)
              n1064 = local read "STOP_abort"() -> (w2804:bool)
              n1065 = Select(t=w2787, s=w2783, f=w2786) -> (s? t:f=w2781:i32)
              n1066 = To Unsigned Word Integer(number=w2777) -> (unsigned 16bit integer=w2779:u16)
              n1067 = Not(x=w2807) -> (.not. x?=w2806:bool)
              n1068 = Replace Array Subset(array=w2782, new element=w2779, index=w2781) -> (w2780:u16[])
              n1069 = Compound Arithmetic op=OR(w2806, w2802, w2805, w2804) -> (w2803:bool)
              n1070 = Select(t=myRIO_BRig_RT__Case_Exp_stateList."endExp" ("Enum"), s=w2803, f=myRIO_BRig_RT__Case_Exp_stateList."dummyState_endBlock" ("Enum")) -> (s? t:f=w2811:T2)
            }
            frame 66 {
            }
            frame 67 {
              n1071 = call "myRIO_BRig_RT_comm_webdav_connect.vi"("input_password"="Host Password", "input_username"="Host UserName") -> ("output_Iconnected"=w2832:bool, "output_hSession"=w2850:T7)  [unwired: 7 in, 1 out]
              "Connected To Host?" <- w2832
              n1072 = case shown="False" w2832 {
                frame False {
                  n1073 = One Button Dialog(message="Connection Failed!\nData not being saved!") -> ()  [unwired: 1 in, 1 out]
                }
                frame True {
                }
              }
            }
            frame 68 {
              n1074 = Select(t=myRIO_BRig_RT__Case_Exp_stateList."commUpload_dataBlock" ("Enum"), s=w2857, f=myRIO_BRig_RT__Case_Exp_stateList."endBlock") -> (s? t:f=w2855:T2)
            }
            frame 69 {
              n1075 = call "myRIO_BRig_RT_comm_webdav_uploadFile__data.vi"("input_fileName_prefix"=w2878, "input_fileName"="dataBlock" ("input_filename"), "input_hSession"=w2880) -> ()  [unwired: 8 in, 1 out]
            }
            frame 70 {
              n1076 = call "myRIO_BRig_RT_comm_webdav_uploadFile__data.vi"("input_fileName_prefix"=w2899, "input_fileName"="dataCurrent" ("input_filename"), "input_hSession"=w2901) -> ()  [unwired: 8 in, 1 out]
            }
            frame 71 {
              n1077 = call "myRIO_BRig_RT_comm_webdav_uploadFile__data.vi"("input_fileName_prefix"=w2920, "input_fileName"="dataExp" ("input_filename"), "input_hSession"=w2922) -> ()  [unwired: 8 in, 1 out]
            }
            frame 72 {
              n1078 = call "myRIO_BRig_RT_comm_webdav_uploadFile__data.vi"("input_fileName_prefix"=w2941, "input_fileName"="dataLC" ("input_filename"), "input_hSession"=w2943) -> ()  [unwired: 8 in, 1 out]
            }
            frame 73 {
              n1079 = call "myRIO_BRig_RT_comm_webdav_uploadFile__data.vi"("input_fileName_prefix"=w2965, "input_fileName"="dataTrial" ("input_filename"), "input_hSession"=w2967) -> ()  [unwired: 8 in, 1 out]
            }
            frame 76 {
              # "idxDataBlockR"
              # "idxDataBlockL"
              n1080 = call "myRIO_BRig_RT_dataCurrent_idxDataBlockL.vi"() -> ("output_idxDataBlock__L"=w2991:i32)  [unwired: 11 in]
              n1081 = call "myRIO_BRig_RT_dataCurrent_idxDataBlockR.vi"() -> ("output_idxDataBlock__R"=w2992:i32)  [unwired: 11 in]
              n1082 = Index Array(array=w2993, index #1=w2991, index #2=w2992) -> (element #1=w2990:u16, element #2=w2989:u16)
              n1083 = Greater?(x=w2990, y=w2989) -> (0:w2988:bool)
              n1084 = Select(t=w2990, s=w2988, f=w2989) -> (s? t:f=w2986:u16)
              n1085 = Increment(x=w2986) -> (x+1=w2985:u16)
              n1086 = To Long Integer(number=w2985) -> (32bit integer=w2984:i32)
              n1087 = Array Subset(array=w2987, length (row)=w2984) -> (w2983:u16[][])  [unwired: 3 in]
              n1088 = call "myRIO_BRig_RT_comm_webdav_saveArrayToFile__2D_u16.vi"("Array"=w2983, "input_filename"="dataBlock") -> ()  [unwired: 10 in]
            }
            frame 77 {
              n1089 = call "myRIO_BRig_RT_comm_webdav_saveArrayToFile__1D_u16.vi"("Array"=w3012, "input_filename"="dataCurrent") -> ()  [unwired: 10 in]
            }
            frame 78 {
              # "runTime"
              n1090 = Get Date/Time In Seconds() -> (seconds since 1Jan1904=w3040:timestamp)
              n1091 = To Double Precision Float(number=w3040) -> (double precision float=w3039:dbl)
              n1092 = call "myRIO_BRig_RT_dataExp_runTime_seconds.vi"() -> ("output_RunTime_minutes"=w3038:i32)  [unwired: 11 in]
              n1093 = Subtract(x=w3039, y=w3037) -> (x-y=w3034:dbl)
              n1094 = To Unsigned Word Integer(number=w3034) -> (unsigned 16bit integer=w3033:u16)
              n1095 = Replace Array Subset(array=w3032, new element=w3033, index=w3038) -> (w3035:u16[])
              n1096 = call "myRIO_BRig_RT_comm_webdav_saveArrayToFile__1D_u16.vi"("Array"=w3035, "input_filename"="dataExp") -> ()  [unwired: 10 in]
            }
            frame 79 {
              n1097 = call "myRIO_BRig_RT_comm_webdav_saveArrayToFile__1D_u16.vi"("Array"=w3059, "input_filename"="dataLC") -> ()  [unwired: 10 in]
            }
            frame 80 {
              # "idxTrial"
              n1098 = call "myRIO_BRig_RT_dataCurrent_idxDataTrial.vi"() -> ("output_idxDataTrial"=w3083:i32)  [unwired: 11 in]
              n1099 = Index Array(array=w3084, index=w3083) -> (element=w3076:u16)
              n1100 = Increment(x=w3076) -> ()  [unwired: 1 out]
              n1101 = To Long Integer(number=w3076) -> (32bit integer=w3080:i32)
              n1102 = Array Subset(array=w3081, length (row)=w3080) -> (w3082:u16[][])  [unwired: 3 in]
              n1103 = call "myRIO_BRig_RT_comm_webdav_saveArrayToFile__2D_u16.vi"("Array"=w3082, "input_filename"="dataTrial") -> ()  [unwired: 10 in]
            }
            frame 89 {
              n1104 = call "myRIO_BRig_RT_dataCurrent_iTrial.vi"() -> ("output_iTrial"=w3106:i32)  [unwired: 11 in]
              n1105 = Index Array(array=w3107, index=w3106) -> (element=w3105:u16)
              n1106 = Equal?(x=w3105, y=u16 1) -> (x = y?=w3103:bool)
              n1107 = Equal To 0?(x=w3114) -> (x = 0?=w3115:bool)
              n1108 = Select(t=u16 13, s=w3103, f=u16 15) -> (s? t:f=w3100:u16)
              n1109 = Select(t=w3100, s=w3115, f=w3114) -> (s? t:f=w3113:u16)
              n1110 = Decrement(x=w3113) -> (x-1=w3112:u16)
              n1111 = Equal To 0?(x=w3112) -> (x = 0?=w3111:bool)
              n1112 = Select(t=myRIO_BRig_RT__Case_Exp_stateList."initTrial" ("Enum"), s=w3111, f=w3109) -> (s? t:f=w3108:u16)
            }
            frame 90 {
              n1113 = call "myRIO_BRig_RT_dataCurrent_iTrial.vi"() -> ("output_iTrial"=w3139:i32)  [unwired: 11 in]
              n1114 = Index Array(array=w3140, index=w3139) -> (element=w3138:u16)
              n1115 = Equal?(x=w3138, y=u16 1) -> (x = y?=w3136:bool)
              n1116 = Equal To 0?(x=w3147) -> (x = 0?=w3148:bool)
              n1117 = Select(t=u16 1, s=w3136, f=u16 3) -> (s? t:f=w3133:u16)
              n1118 = Select(t=w3133, s=w3148, f=w3147) -> (s? t:f=w3146:u16)
              n1119 = Decrement(x=w3146) -> (x-1=w3145:u16)
              n1120 = Equal To 0?(x=w3145) -> (x = 0?=w3144:bool)
              n1121 = Select(t=myRIO_BRig_RT__Case_Exp_stateList."initBlock" ("Enum"), s=w3144, f=w3142) -> (s? t:f=w3141:u16)
            }
          }
          n1122 = Select(t=w1081, s=w1084, f=w1082) -> (s? t:f=w1083:bool)
          n1123 = case shown="True" w1155 {
            tunnel: w1152 -> [w1176 w1184]
            tunnel: w1154 -> [_ w1180]
            tunnel: w1153 -> [_ w1179]
            tunnel: w1055 -> [_ w1178]
            tunnel: w1122 -> [_ w1177]
            tunnel: [w1176 w1183] -> w1151
            tunnel: w1150 -> [w1175 w1182]
            tunnel: [w1175 w1181] -> w1149
            frame False {
            }
            frame True {
              n1124 = call "myRIO_BRig_RT__Case_Exp__recordLick.vi"("intput_state__trialEnd"=w1177, "intput_state__trialStart"=w1178, "input_lick__R"=w1179, "input_lick__L"=w1180, "input_dataCurrent"=w1182, "input_dataLick"=w1184) -> ("output_dataCurrent"=w1181:u16[], "output_dataLick"=w1183:u16[][])  [unwired: 4 in]
            }
          }
          n1125 = Or(x=w1124, y=w1125) -> (x .or. y?=w1111:bool)
          n1126 = Or(x=w1128, y=w1108) -> (x .or. y?=w1097:bool)
          n1127 = Or(x=w1107, y=w1129) -> (x .or. y?=w1123:bool)
          n1128 = Or(x=w1127, y=w1126) -> (x .or. y?=w1112:bool)
          n1129 = Or(x=w1156, y="STOP_abort") -> (x .or. y?=w1158:bool)
          n1130 = Or(x=w1087, y=w1088) -> (x .or. y?=w1085:bool)
          n1131 = Or(x=w1089, y=w1088) -> (x .or. y?=w1086:bool)
          n1132 = Select(t=w1070, s=w1071, f=w1069) -> (s? t:f=w1054:u16)
          n1133 = Select(t=w1072, s=w1074, f=w1073) -> (s? t:f=w1053:u16)
          n1134 = Select(t=u16 0, s=w1077, f=w1076) -> (s? t:f=w1061:u16)
          n1135 = xnode "Read/Write Control"("FPGA VI Reference In"=w1099, "error in"=w1098, "A1_SR"=w1112, "A3_SL"=w1111, "A6_Act"=w1083, "audioTrigger_L"=w1097, "audioAmp_L"=w1138, "audioFreq_L_kHz"=w1106, "audioTrigger_R"=w1123, "audioAmp_R"=w1139, "audioFreq_R_kHz"=w1140, "laserledMTrig"=w1085, "laserMTrig"=w1086) -> ("FPGA VI Reference Out"=w1148:refnum<k20>, "error out"=w1147:errorcluster, "AnaIn_0"=w1047:i16, "AnaIn_1"=w1060:i16)
          n1136 = call "myRIO_BRig_RT_dataAnalog_enterData__PortC.vi"("input_iState"=w1055, "input_AI0"=w1047, "input_iEvent"=w1061, "input_AI1"=w1060, "input_iTrial"=w1054, "input_iBlock"=w1053, "input_index"=w1062, "input_dataAnalog"=w1080) -> ("output_dataAnalog"=w1079:u16[][])  [unwired: 3 in]
          n1137 = call "myRIO_BRig_RT_TCP__v3__PortC.vi"("input_hTCP"=w1067, "input_AI1"=w1060, "input_AI0"=w1047, "input_I_connected_TCP"=w1063, "input_iBlock"=w1053, "input_spout"=w1052, "input_iTrial"=w1054, "input_error"=w1065, "input_countTrial"=w1049, "input_iState"=w1055) -> ("output_hTCP"=w1066:refnum<k5>, "output_countTrial"=w1048:u16, "output_error"=w1064:errorcluster)  [unwired: 3 in]
          n1138 = node-c288() -> ()  [unwired: 1 in, 1 out]
          n1139 = Increment(x=w1061) -> (x+1=w1068:u16)
          n1140 = Increment(x=w1062) -> (x+1=w1078:i32)
          "cState" <- w1055
        }
        n1141 = node-c288(w997) -> ()  [unwired: 1 out]
        n1142 = flat-sequence {
          tunnel: w993 -> [w1042]
          tunnel: w992 -> [w1041]
          tunnel: [w1040] -> w985
          tunnel: [w1039] -> w984
          tunnel: [w1045] -> w986
          tunnel: [w1046] -> w991
          tunnel: w985 -> [w1046]
          tunnel: w984 -> [w1045]
          frame #0 {
            w1036 = u8 0
            w1037 = u16 0 ("AudioLeft_phase_inc")
            w1038 = FALSE
            n1143 = xnode "Read/Write Control"("FPGA VI Reference In"=w1042, "error in"=w1041, "Counts_Reset"=TRUE, "audioTrigger_L"=w1038, "audioFreq_L_kHz"=w1036, "audioAmp_L"=w1037, "audioTrigger_R"=w1038, "audioFreq_R_kHz"=w1036, "audioAmp_R"=w1037, "A3_SL"=w1038, "A1_SR"=w1038, "A6_Act"=w1038) -> ("FPGA VI Reference Out"=w1040:refnum<k20>, "error out"=w1039:errorcluster)
          }
          frame #1 {
            w1044 = FALSE ("START")
            n1144 = local write "START"(w1044) -> ()
            n1145 = local write "STOP_endTrial"(w1044) -> ()
            n1146 = local write "STOP_endBlock"(w1044) -> ()
          }
        }
        n1147 = stacked-sequence {
          tunnel: w969 -> [w1016 _]
          tunnel: w967 -> [w1017 _]
          tunnel: w966 -> [_ w1022]
          tunnel: w965 -> [_ w1021]
          tunnel: w964 -> [_ w1020]
          tunnel: w963 -> [w1010 _]
          tunnel: w938 -> [w1007 _]
          tunnel: w937 -> [w1006 _]
          frame #0 {
            n1148 = call "myRIO_BRig_RT_dataCurrent_idxDataLick.vi"() -> ("output_idxDataLick"=w1011:i32)  [unwired: 11 in]
            n1149 = Index Array(array=w1010, index=w1011) -> (element=w1013:u16)
            n1150 = Array Subset(array=w1007, length (row)=w1006) -> (w1008:u16[][])  [unwired: 3 in]
            n1151 = Increment(x=w1013) -> (x+1=w1014:u16)
            n1152 = call "myRIO_BRig_RT_comm_webdav_saveArrayToFile__1D_u16.vi"("Array"=w1017, "input_filename"="dataMTrig") -> ()  [unwired: 10 in]
            n1153 = To Long Integer(number=w1014) -> (32bit integer=w1012:i32)
            n1154 = Array Subset(array=w1016, length (row)=w1012) -> (w1015:u16[][])  [unwired: 3 in]
            n1155 = call "myRIO_BRig_RT_comm_webdav_saveArrayToFile__2D_u16.vi"("Array"=w1015, "input_filename"="dataLick") -> ()  [unwired: 10 in]
            n1156 = call "myRIO_BRig_RT_comm_webdav_saveArrayToFile__2D_u16.vi"("Array"=w1008, "input_filename"="dataAnalog") -> ()  [unwired: 10 in]
          }
          frame #1 {
            n1157 = case shown="True" w1022 {
              tunnel: w1021 -> [_ w1024]
              tunnel: w1020 -> [_ w1023]
              frame False {
              }
              frame True {
                n1158 = stacked-sequence {
                  tunnel: w1024 -> [w1026 w1033 w1035]
                  tunnel: w1023 -> [w1027 w1032 _]
                  frame #0 {
                    n1159 = call "myRIO_BRig_RT_comm_webdav_uploadFile__announce.vi"("input_addText"=TRUE, "input_fileName_prefix"=w1027, "intput_fileName"="curExp_end", "intput_hSession"=w1026) -> ("output_Isuccess"=w1025:bool)  [unwired: 6 in, 1 out]
                    n1160 = case shown="True" w1025 {
                      frame False {
                        n1161 = One Button Dialog(message="!!! Warning !!! Your data is located at C:\\BehaviorRig\\commTransfer") -> ()  [unwired: 1 in, 1 out]
                      }
                      frame True {
                        n1162 = Wait (ms)(milliseconds to wait=u32 20) -> ()  [unwired: 1 out]
                      }
                    }
                  }
                  frame #1 {
                    n1163 = call "myRIO_BRig_RT__endExp_sendData.vi"("input_fileName_prefix"=w1032, "input_hSession"=w1033) -> ()  [unwired: 8 in, 2 out]
                  }
                  frame #2 {
                    n1164 = local write "Connected To Host?"(FALSE ("Connected To Host?")) -> ()
                    n1165 = call <vilib>:"Close Session.vi"("session handle"=w1035) -> ()  [unwired: 14 in, 1 out]
                  }
                }
              }
            }
          }
        }
      }
    }
    n1166 = local read "STOP_abort"() -> (w44:bool)
  }
  n1167 = case shown="True" w5 {
    tunnel: w4 -> [_ w3171]
    tunnel: w3 -> [_ w3170]
    frame False {
    }
    frame True {
      n1168 = call "myRIO__TCP_disconnect_forWrite.vi"("input_error"=w3170, "input_hTCP"=w3171) -> ()  [unwired: 9 in, 1 out]
    }
  }
  n1169 = xnode "Read/Write Control"("FPGA VI Reference In"=w16, "error in"=w15, "FPGA_Stop"=TRUE) -> ("FPGA VI Reference Out"=w21:refnum<k20>, "error out"=w22:errorcluster)
  n1170 = xnode "Close FPGA VI Reference"("FPGA VI Reference In"=w21, "error in"=w22) -> ("error out"=w20:errorcluster)
  n1171 = call <vilib>:"Reset myRIO.vi"("error in (no error)"=w20) -> ()  [unwired: 10 in, 1 out]
